vi "myRIO_BRig_RT_v0,86.vi"() -> ()   [LabVIEW 2014]
uses:
  myRIO_BRig_RT__Case_Exp_stateList.ctl
  myRIO_BRig_RT__Case_NonExp_stateList.ctl
  <vilib>/Platform/TimedLoop/XDataNode/timing_clust.ctl
  <vilib>/Platform/TimedLoop/XDataNode/nitl_modes.ctl
  <vilib>/Platform/TimedLoop/XDataNode/wakeup.ctl
  <vilib>/WebDAVClient/Advanced/SessionHandle.ctl
  <vilib>/myRIO/Common/Instrument Driver Framework/myRIO v1.0/UART/vis/myRIO v1.0 Close UART.vi
  <vilib>/FPGAPlugInAG/myRIO-1900/niLvFpga_Open_myRIO-1900.vi
  <vilib>/rvi/interface/common/dynamic/niFpgaDynamicAddResources.vi
  <vilib>/Utility/error.llb/Error Cluster From Error Code.vi
  <vilib>/rvi/errors/niLvFpgaAdjustHostInterfaceError.vi
  <vilib>/FPGAPlugInAG/Dynamic/niLvFpga_Close_Dynamic.vi
  <vilib>/myRIO/Common/Instrument Driver Framework/Utilities/vis/FPGA Ref Manager.vi
  <vilib>/myRIO/Common/Instrument Driver Framework/myRIO v1.0/myRIO v1.0 Reset FPGA.vi
  <vilib>/myRIO/Common/Instrument Driver Framework/myRIO v1.0/IRQ/vis/myRIO v1.0 IRQ Info FGV.vi
  <vilib>/myRIO/Common/Instrument Driver Framework/myRIO v1.0/IRQ/vis/myRIO v1.0 Timer IRQ Info FGV.vi
  <vilib>/myRIO/Common/Instrument Driver Framework/myRIO v1.0/IRQ/vis/myRIO v1.0 ISR Agent.vi
  <vilib>/rvi/interface/nirviOpenFPGA/nirviOpenFPGA.xnode
  myRIO_BRig_FPGA_v3,81_build.lvbitx
  myRIO_BRig_FPGA_v3,81.vi
  <vilib>/rvi/interface/nirviReadWriteControl/nirviReadWriteControl.xnode
  <vilib>/Platform/TimedLoop/XDataNode/XDataNode.xnode
  <vilib>/rvi/interface/nirviCloseFPGA/nirviCloseFPGA.xnode
  <vilib>/Platform/TimedLoop/XDataNode/XDNodeRunTimeDep.lvlib
  <vilib>/rvi/interface/Simulation/niFpgaSimulationCallBeginRW.vi
  <vilib>/myRIO/Instrument Drivers/Utilities/Utilities.lvlib
  <vilib>/WebDAVClient/NI_WebDAV.lvlib
  NiFpgaLv.dll
panel:
  in  "Laser2_baseline":bool
  in  "Laser1_baseline":bool
  in  "CueLed_baseline":bool
  out "allReward_R":bool
  out "allReward_L":bool
  in  "I_allReward":bool caption="NonSpecific Lick Direction"
  in  "Tcycle_Reward_max_R":u16=1000 caption="Max" min=5 max=5000 step=5
  in  "Tcycle_Reward_min_R":u16=1000 caption="Min" min=5 max=5000 step=5
  in  "Tcycle_Reward_step_R":u16=1000 caption="Penalty" min=1 max=10000 step=1
  in  "Tcycle_Reward_max_L":u16=1000 caption="Max" min=5 max=5000 step=5
  in  "Tcycle_Reward_min_L":u16=1000 caption="Min" min=5 max=5000 step=5
  in  "Tcycle_Reward_step_L":u16=1000 caption="Penalty" min=1 max=10000 step=1
  in  "MTrig_CueLed":bool
  out "Threshold":bool
  out "tLoop":dbl
  in  "Tcycle_Cue_LED_max":u16=1000 caption="Max" min=5 max=5000 step=5
  in  "Tcycle_Cue_LED_min":u16=1000 caption="Min" min=5 max=5000 step=5
  in  "Tcycle_CuePenalty_LED":u16=1000 caption="Penalty" min=1 max=10000 step=1
  out "power_l2":dbl
  in  "MTrig_Laser_Switch":bool
  in  "Cue1Param_AudioLed_Count_NS":u16
  in  "Cue1Param_AudioLed_Count_Switch":u16
  in  "Cue1Param_AudioLed_Probability_NS":u16
  in  "Cue1Param_CueType_NS":u16(slide) max=3 step=1 scale=0.0..3.0
  in  "Cue1Param_AudioLed_Probability_Switch":u16
  in  "Cue1Param_CueType_Switch":u16(slide) max=3 step=1 scale=0.0..3.0
  in  "CueLed_Freq":dbl=10.0
  in  "CueLed_Tpeak":dbl=2.0
  in  "Laser_power_step_l2":dbl
  in  "Laser_power_max_l2":dbl
  in  "Laser_power_min_l2":dbl
  in  "Laser_Tshutter_l2":dbl=2.0
  in  "Laser_Freq_l2":dbl=10.0
  in  "Laser_Tpeak_l2":dbl=2.0
  in  "Laser_duration_l2":u16
  in  "LC_Sel_Count_NS_l2":u16
  in  "LC_Sel_Count_Switch_l2":u16
  in  "LC_Sel_Probability_NS_l2":u16
  in  "LC_Sel_Block_NS_l2":u16(slide) max=2 step=1 scale=0.0..2.0
  in  "LC_Sel_OnOff_NS_l2":bool
  in  "LC_Sel_Probability_Switch_l2":u16
  in  "LC_Sel_Block_Switch_l2":u16(slide) max=2 step=1 scale=0.0..2.0
  in  "LC_Sel_OnOff_Switch_l2":bool
  in  "LC_Sel_Tdelay_NS_l2":u16
  in  "LC_Sel_Tdelay_Switch_l2":u16
  in  "LC_Cue1_Count_NS_l2":u16
  in  "LC_Cue1_Count_Switch_l2":u16
  in  "LC_Cue1_delayOpt_NS_l2":bool
  in  "LC_ENL1_delayOpt_NS_l2":bool
  in  "LC_ENL1_Count_NS_l2":u16
  in  "LC_ENL1_Count_Switch_l2":u16
  in  "LC_Cue1_delayOpt_Switch_l2":bool
  in  "LC_ENL1_delayOpt_Switch_l2":bool
  in  "LC_Cue1_Probability_NS_l2":u16
  in  "LC_Cue1_Block_NS_l2":u16(slide) max=2 step=1 scale=0.0..2.0
  in  "LC_Cue1_OnOff_NS_l2":bool
  in  "LC_Cue1_Probability_Switch_l2":u16
  in  "LC_Cue1_Block_Switch_l2":u16(slide) max=2 step=1 scale=0.0..2.0
  in  "LC_Cue1_OnOff_Switch_l2":bool
  in  "LC_ENL1_Probability_NS_l2":u16 max=100 step=1
  in  "LC_ENL1_Block_NS_l2":u16(slide) max=2 step=1 scale=0.0..2.0
  in  "LC_ENL1_OnOff_NS_l2":bool
  in  "LC_ENL1_Probability_Switch_l2":u16 max=100 step=1
  in  "LC_ENL1_Block_Switch_l2":u16(slide) max=2 step=1 scale=0.0..2.0
  in  "LC_Cue1_Tdelay_NS_l2":u16
  in  "LC_ENL1_Tdelay_NS_l2":u16
  in  "LC_Cue1_Tdelay_Switch_l2":u16
  in  "LC_ENL1_Tdelay_Switch_l2":u16
  in  "LC_ENL1_OnOff_Switch_l2":bool
  in  "LC_Wrong_Probability_l2":u16
  in  "LC_Wrong_Trial_l2":u16(slide) max=2 step=1 scale=0.0..2.0
  in  "LC_Wrong_Block_l2":u16(slide) max=2 step=1 scale=0.0..2.0
  in  "LC_Wrong_OnOff_l2":bool
  in  "LC_Reward_Probability_l2":u16
  in  "LC_Reward_Trial_l2":u16(slide) max=2 step=1 scale=0.0..2.0
  in  "LC_Reward_Block_l2":u16(slide) max=2 step=1 scale=0.0..2.0
  in  "LC_Reward_OnOff_l2":bool
  in  "LC_Wrong_Tdelay_l2":u16
  in  "LC_Reward_Tdelay_l2":u16
  in  "LC_Sel_Count_NS_l1":u16
  in  "LC_Sel_Count_Switch_l1":u16
  in  "LC_Sel_Probability_NS_l1":u16
  in  "LC_Sel_Block_NS_l1":u16(slide) max=2 step=1 scale=0.0..2.0
  in  "LC_Sel_OnOff_NS_l1":bool
  in  "LC_Sel_Probability_Switch_l1":u16
  in  "LC_Sel_Block_Switch_l1":u16(slide) max=2 step=1 scale=0.0..2.0
  in  "LC_Sel_OnOff_Switch_l1":bool
  in  "LC_Sel_Tdelay_NS_l1":u16
  in  "LC_Sel_Tdelay_Switch_l1":u16
  out "I_connect_TCP":bool
  in  "get_countPerMS":bool
  in  "count_warmup_R_reset":bool
  in  "count_warmup_L_reset":bool
  out "count_warmup_R":u16
  out "count_warmup_L":u16
  out "SolenoidReward":bool
  in  "SolenoidProbability_L":u16=100 caption="Reward Time [ms]" min=1 max=1000 step=1
  in  "SolenoidProbability_R":u16=100 caption="Reward Time [ms]" min=1 max=1000 step=1
  out "power_l1":dbl caption="LaserPower"
  in  "Laser_power_step_l1":dbl
  in  "Laser_power_max_l1":dbl
  in  "Recording":bool
  in  "Laser_power_min_l1":dbl
  in  "FPGA_count2ms":dbl=159.0
  in  "Laser_Tshutter_l1":dbl=2.0
  in  "Laser_Freq_l1":dbl=10.0
  in  "Laser_Tpeak_l1":dbl=2.0
  in  "Laser_duration_l1":u16
  out "error out":errorcluster
  in  "LC_Cue1_Count_NS_l1":u16
  in  "LC_Cue1_Count_Switch_l1":u16
  in  "LC_Cue1_delayOpt_NS_l1":bool
  in  "LC_ENL1_delayOpt_NS_l1":bool
  in  "LC_ENL1_Count_NS_l1":u16
  in  "LC_ENL1_Count_Switch_l1":u16
  in  "LC_Cue1_delayOpt_Switch_l1":bool
  in  "LC_ENL1_delayOpt_Switch_l1":bool
  in  "Tcycle_Cue_Audio_max":u16=1000 caption="Max" min=5 max=5000 step=5
  in  "Tcycle_Cue_Audio_min":u16=1000 caption="Min" min=5 max=5000 step=5
  in  "SendData":bool
  out "cSpout":enum16{"Left", "Right"}(ring) caption="Left or Right Spout"
  out "A4":u32 caption="LickCounter_Right"
  out "A2":u32 caption="LickCounter_Left"
  in  "LR_wrong_Event":bool
  out "SelectWrong":bool
  out "SelectReward":bool
  in  "Left(F)_or_Right(T)":bool
  in  "ignoreWrong":bool
  in  "SelectionState":bool
  in  "LR_wrong_Laser":bool
  in  "LR_reward_Laser":bool
  in  "LR_reward_Event":bool
  out "nRewards_Right":u16 caption="# Rewards Total (Right)"
  out "nRewards_Left":u16 caption="# Rewards Total (Left)"
  out "nRewards_cur":u16 caption="# Rewards in Current Block"
  out "TpB_target":u16 caption="Target Trials Per Block"
  out "cState_NonExp":T1 caption="WarmUp State"
  out "iBlock":u16 caption="Current Block"
  out "cState":T2 caption="Experimental State"
  out "iTrial":u16 caption="Current Trial"
  in  "warmupType":u8(slide) max=2 step=1 scale=0.0..2.0
  in  "TestConnection":bool
  in  "warmup":bool caption="WarmUp"
  in  "Data Set Prefix":string="Exp1_TM2"
  out "Connected To Host?":bool
  in  "Host Password":string="sabalab"
  in  "Host UserName":string="Test2"
  in  "sp_RightSpout":u16(slide)=2 max=2 step=1 scale=0.0..2.0
  in  "sp_LeftSpout":u16(slide)=2 max=2 step=1 scale=0.0..2.0
  in  "BUR_max":u16 caption="Count Reward Structure  (0 = off)"
  in  "LC_Wrong_Probability_l1":u16
  in  "LC_Wrong_Trial_l1":u16(slide) max=2 step=1 scale=0.0..2.0
  in  "LC_Wrong_Block_l1":u16(slide) max=2 step=1 scale=0.0..2.0
  in  "LC_Wrong_OnOff_l1":bool
  in  "LC_Reward_Probability_l1":u16
  in  "LC_Reward_Trial_l1":u16(slide) max=2 step=1 scale=0.0..2.0
  in  "LC_Reward_Block_l1":u16(slide) max=2 step=1 scale=0.0..2.0
  in  "LC_Reward_OnOff_l1":bool
  in  "LC_Cue1_Probability_NS_l1":u16
  in  "LC_Cue1_Block_NS_l1":u16(slide) max=2 step=1 scale=0.0..2.0
  in  "LC_Cue1_OnOff_NS_l1":bool
  in  "LC_Cue1_Probability_Switch_l1":u16
  in  "LC_Cue1_Block_Switch_l1":u16(slide) max=2 step=1 scale=0.0..2.0
  in  "LC_Cue1_OnOff_Switch_l1":bool
  in  "LC_ENL1_Probability_NS_l1":u16 max=100 step=1
  in  "LC_ENL1_Block_NS_l1":u16(slide) max=2 step=1 scale=0.0..2.0
  in  "LC_ENL1_OnOff_NS_l1":bool
  in  "LC_ENL1_Probability_Switch_l1":u16 max=100 step=1
  in  "LC_ENL1_Block_Switch_l1":u16(slide) max=2 step=1 scale=0.0..2.0
  in  "Tcycle_Timeout":u16=1000 caption="Timeout Time [ms]" min=10 max=10000 step=1
  in  "Tcycle_Wrong":u16=1000 caption="Wrong Time [ms]" min=10 max=10000 step=1
  in  "Tcycle_Selection":u16=1000 caption="Answer Time [ms]" min=1 max=10000 step=1
  in  "Tcycle_RewardPost":u16=1000 caption="Consumption Time [ms]" min=250 max=10000 step=250
  in  "TpB_Max_R":u16=4 caption="Max TrialsPerBlock" min=1 max=12 step=1
  in  "TpB_Min_R":u16=4 caption="Min TrialsPerBlock" min=1 max=12 step=1
  in  "TpB_Max_L":u16=4 caption="Max TrialsPerBlock" min=1 max=12 step=1
  in  "TpB_Min_L":u16=4 caption="Min TrialsPerBlock" min=1 max=12 step=1
  in  "BUR_min":u16 caption="Count Reward Structure\n(0 = off)"
  in  "TrialUntilReward":bool caption="Ignore Wrong Selection"
  in  "CueCycles":u16=1 caption="Cue Structure" min=1 max=1 step=1
  in  "MTrig_Laser_Tcycle":u16=10 caption="Time [ms]"
  in  "MTrig_Laser_trig":bool
  in  "MTrig_Audio_trig__R":bool caption="Trigger Audio"
  in  "MTrig_Audio_trig__L":bool caption="Trigger Audio"
  in  "RewCalib_Trig_R":bool caption="Calibrate_R"
  in  "RewCalib_Trig_L":bool caption="Calibrate_L"
  in  "MTrig_Solenoid_Tcycle__R":u16=300 caption="Time [ms]"
  in  "MTrig_Solenoid_Tcycle__L":u16=300 caption="Time [ms]"
  in  "MTrig_Solenoid_trig__R":bool caption="Solenoid"
  in  "MTrig_Solenoid_trig__L":bool caption="Solenoid"
  in  "STOP_abort":bool caption="Stop LabView\n(Stops myRio and FPGA)"
  in  "STOP_endBlock":bool caption="Stop Experiment\n@ End of Block"
  in  "STOP_endTrial":bool caption="Stop Experiment\n@ End of Trial"
  in  "START":bool caption="Start Experiment"
  in  "Tcycle_CuePenalty_Audio":u16=1000 caption="Penalty" min=1 max=10000 step=1
  in  "Audio_Amp__R":u16=100 caption="Amp"
  in  "Audio_Freq__R":u8=5 caption="Freq [kHz]" max=14 step=1
  in  "Audio_Amp__L":u16=100 caption="Amp"
  in  "Audio_Freq__L":u8=5 caption="Freq [kHz]" max=14 step=1
  in  "LC_Wrong_Tdelay_l1":u16
  in  "LC_Cue1_Tdelay_NS_l1":u16
  in  "LC_ENL1_Tdelay_NS_l1":u16
  in  "LC_Reward_Tdelay_l1":u16
  in  "LC_Cue1_Tdelay_Switch_l1":u16
  in  "LC_ENL1_Tdelay_Switch_l1":u16
  in  "LC_ENL1_OnOff_Switch_l1":bool
  in  "Tcycle_ENLPenalty":u16=100 caption="Penalty" min=10 max=10000 step=10
  in  "Tcycle_ENL_max":u16=1000 caption="Max" min=250 max=10000 step=250
  in  "Tcycle_ENL_min":u16=1000 caption="Min" min=250 max=10000 step=250
  # "Communication (Host PC)"
  # "Recording Rig"
  # "Experimental Run"
  # "Experiment Task Structure"
  # "STOP experiment at"
  # "(1) = Switching\n(2) = Two Choice"
  # "Min            Max            Penalty"
  # "Enforced\nNonLick"
  # "FPGA Count per [ms]"
  # "Cue Audio"
  # "Current State"
  # "Cue LED"
  # "Global Parameters                                                         Trial Parameters"
  # "Selection"
  # "WarmUp"
  # "Reward - Dispense Water"
  # "Left/Right        Give Reward?        Laser Power [V]"
  # "Min            Max            StepSize"
  # "Laser1      Laser2"
  # "Left"
  # "Cue then reward (no lick)\n \nLeft                    Right"
  # "Right"
  # "Min"
  # "Max"
  # "Dispense Water Probability"
  # "Block                   Trial            Target Trials       # Rewards \n                                                            Per Block             Current"
  # "%"
  # "Left"
  # "WarmUp State"
  # "Trial Per Block Structure \n               Left                        Right"
  # "Lick Counter"
  # "Right"
  # "%"
  # "Left           Right"
  # "Reward - Consumption"
  # "Manual Control"
  # "Min"
  # "# Rewards Total\n                                                                  Left                    Right"
  # "Experimental State"
  # "Penalty - Wrong Choice"
  # "Solenoid\n \nLeft              Right"
  # "Speaker\n \nLeft                    Right"
  # "Laser 1  |  Laser 2"
  # "Max"
  # "Penalty - Choice Timeout"
  # "Time\n[ms]"
  # "Time\n[ms]"
  # "Time = Cue Min"
  # "Cue LED"
  # "Power = Min"
  # "Cue1 Control\n                                  Cue Type           LED Probability [%]      Count"
  # "Laser1 Control\n                               On/Off      Block        Probability [%]   Delay [ms]                              Count"
  # "Laser2 Control\n                               On/Off      Block        Probability [%]   Delay [ms]                              Count"
  # "Audio or LED"
  # "Cue 1"
  # "Enforced\nNonLick\n      1"
  # "Enforced\nNonLick\n      1"
  # "from end"
  # "from end"
  # "Switch\nTrial"
  # "Switch\nTrial"
  # "Switch\nTrial"
  # "from start"
  # "from start"
  # "from end"
  # "from end"
  # "NonSwitch\nTrials"
  # "NonSwitch\nTrials"
  # "NonSwitch\nTrials"
  # "from start"
  # "from start"
  # "Cue 1"
  # "Cue 1"
  # "from end"
  # "from end"
  # "Switch\nTrial"
  # "Switch\nTrial"
  # "Cue Audio Parameters"
  # "Cue LED Parameters"
  # "from start"
  # "from start"
  # "Left                  Right"
  # "Frequency\n[Hz]"
  # "Frequency\n[kHz]"
  # "from end"
  # "from end"
  # "NonSwitch\nTrials"
  # "NonSwitch\nTrials"
  # "Timing [ms]\n                    Peak Width"
  # "from start"
  # "from start"
  # "Amp\n(0 - 32,000)"
  # "Selection"
  # "Selection"
  # "from start"
  # "from start"
  # "Switch\nTrial"
  # "Switch\nTrial"
  # "Speaker\nPattern\nDuring Cue"
  # "from start"
  # "from start"
  # "NonSwitch\nTrials"
  # "NonSwitch\nTrials"
  # "Laser1 Parameters"
  # "Laser2 Parameters"
  # "Laser1 Response\n                               On/Off      Block       Trial       Probability [%]   Delay [ms]"
  # "Laser2 Response\n                               On/Off      Block       Trial       Probability [%]   Delay [ms]"
  # "Frequency\n[Hz]"
  # "Frequency\n[Hz]"
  # "Timing [ms]\n Duration     Peak Width   Shutter"
  # "Timing [ms]\n Duration     Peak Width   Shutter"
  # "Selection Reward"
  # "Selection Reward"
  # "Laser Power [V]\nMin          Max              Step"
  # "Laser Power [V]\nMin          Max              Step"
  # "Selection Wrong"
  # "Selection Wrong"
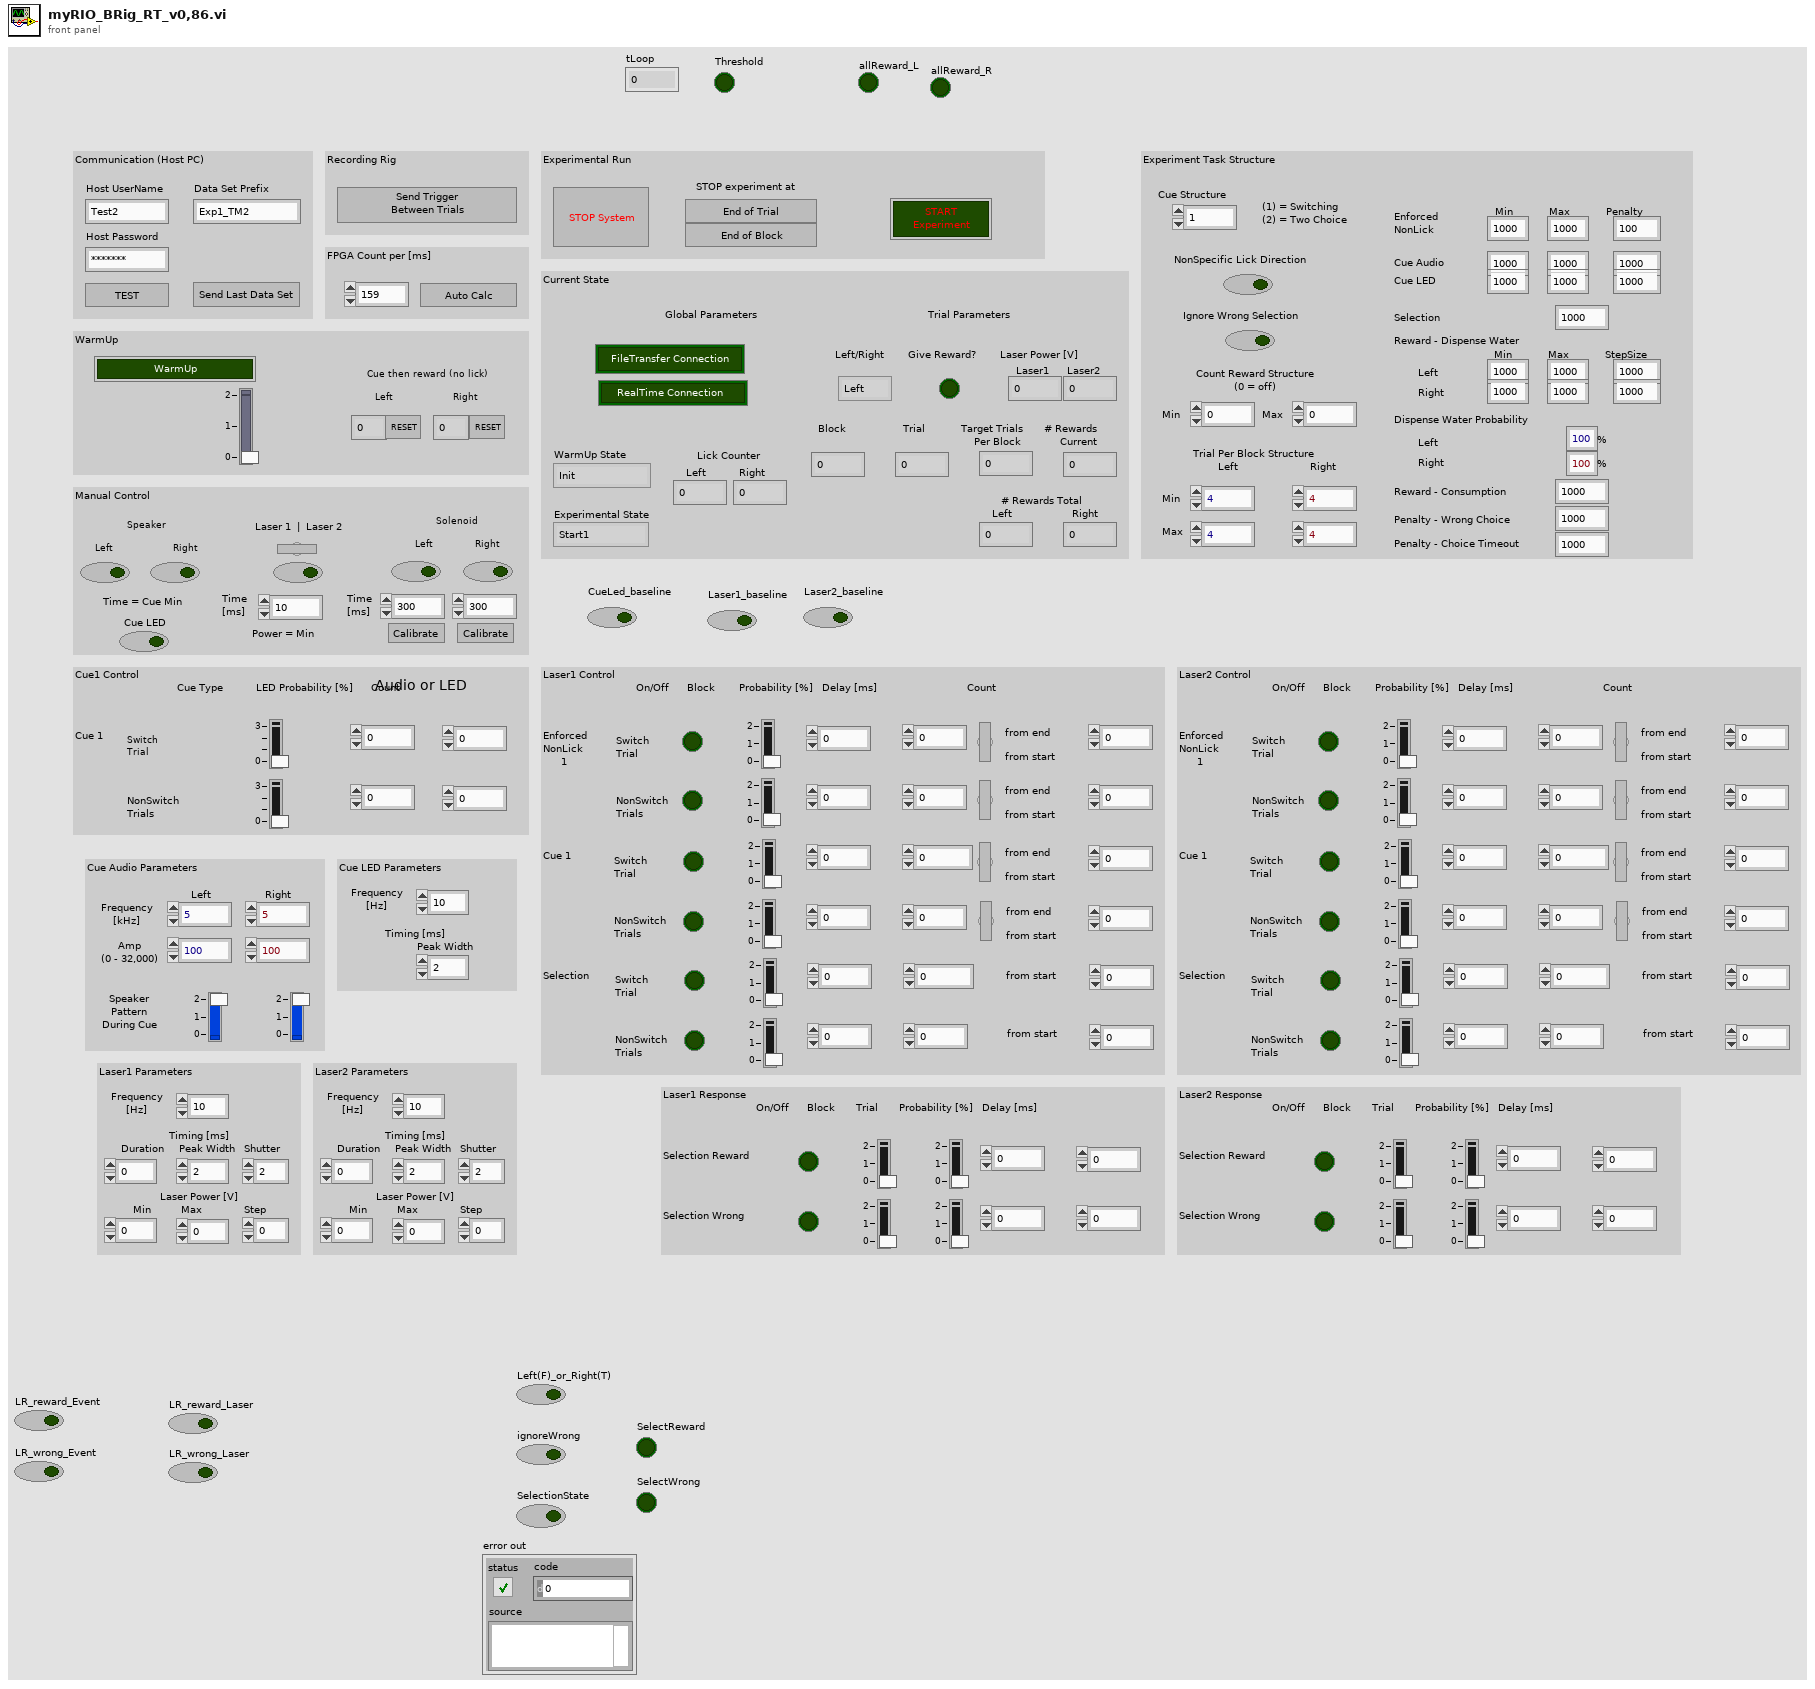
[diagram p1: front panel]
types:
  T1 = typedef "myRIO_BRig_RT__Case_NonExp_stateList.ctl" = enum16{"Init", "UploadSettings_pre", "UploadSettings_Read_dataExp", "UploadSettings_dataExp_1", "UploadSettings_dataExp_2", "UploadSettings_Read_dataLC", "UploadSettings_dataLC_1", "UploadSettings_dataLC_2", "UploadSettings_dataLC_3", "UploadSettings_dataLC_4", "UploadSettings_Read_dataMTrig", "UploadSettings_dataMTrig_1", "UploadSettings_post", "Idle_pre", "IdleEmpty", "IdleEmpty2", "IdleEmpty3", "IdleEmpty4", "Idle", "Idle_2", "Idle_3", "Idle_4", "Idle_5", "Idle_6", "Idle_post", "Cue_pre__pre", "Cue_pre", "Cue", "Cue_LED", "Cue_post", "RewardCalibration_pre", "DispenseWater_pre__pre", "DispenseWater_pre", "DispenseWater", "DispenseWater_post", "TestConnection", "SendData", "Get_FPGA_count_per_ms", "End"}
  T2 = typedef "myRIO_BRig_RT__Case_Exp_stateList.ctl" = enum16{"Start1", "Start2", "Start3", "saveSettings1", "saveSettings2", "saveSettings3", "saveSettings4", "saveSettings_LC_ENL_l1", "saveSettings_LC_ENL_l2", "saveSettings_LC_Cue_l1", "saveSettings_LC_Cue_l2", "saveSettings6_LC_l1_Other", "SaveSettings6_LC_l2_Other", "setSettings_Audio", "setSettings_Laser", "initBlock_pre", "initBlock", "initBlock2", "initBlock_post", "initTrial_pre", "initTrial", "initTrial2", "initTrial3", "initTrial4", "initTrial_LC_ENL1", "initTrial_LC_Cue1", "initTrial_LC_Cue1_2", "initTrial_LC_Sel", "initTrial_post", "ENL1_pre", "ENL1", "ENL1_post", "ENL1Penalty_pre", "ENL1Penalty", "ENL2_pre", "ENL2", "ENL2Penalty_pre", "ENL2Penalty", "Cue1_pre", "Cue1", "Cue1_post", "Cue1Penalty_pre", "Cue1Penalty", "Cue2_pre", "Cue2", "Cue2Penalty_pre", "Cue2Penalty", "Selection_pre", "Selection", "Select_post", "SelectReward_pre", "SelectReward", "SelectRewardPost_pre", "SelectRewardPost", "SelectWrong_pre", "SelectWrong", "SelectWrong_post", "SelectTimeout_pre", "SelectTimeout", "SelectTimeout_post", "endTrial_pre", "endTrial1", "endTrial2", "endTrial3", "endTrial_post", "endBlock_pre", "endBlock", "endBlock_post", "endExp", "commConnect", "commUpload_pre", "commUpload_dataBlock", "commUpload_dataCurrent", "commUpload_dataExp", "commUpload_dataLC", "commUpload_dataTrial", "commUpload_post", "saveData_pre", "saveData_dataBlock", "saveData_dataCurrent", "saveData_dataExp", "saveData_dataLC", "saveData_dataTrial", "saveData_post", "empty_endBlock1", "empty_endBlock2", "empty_endTrial1", "empty_endTrial2", "empty_endTrial3", "empty_endTrial4", "empty_endTrial5", "dummyState", "dummyState_endBlock"}
  T3 = typedef "XDNodeRunTimeDep.lvlib/timing_clust.ctl" = cluster{"Expected End [f-1]":u64, "Actual End [f-1]":u64, "Finished Late? [f-1]":bool, "Expected End [i-1]":u64, "Actual End [i-1]":u64, "Finished Late? [i-1]":bool, "Expected Start [i]":u64, "Actual Start [i]":u64, "Expected Start [f]":u64, "Actual Start [f]":u64, "Source Name":string, "Structure Name":string, "Period":i64, "Deadline":i64, "Offset":i64, "Start":i64, "Priority":i32, "Timeout":i32, "Mode":T4, "Wakeup Reason":T5, "Error":errorcluster, "Source Type":string, "Secondary Source Type":string, "Global End Time":u64, "Global Start Time":u64, "Frame Duration":u64, "Iteration Duration":u64, "Assigned CPU":i32, "I/O Scan Engine Mode":u32}
  T4 = typedef "XDNodeRunTimeDep.lvlib/nitl_modes.ctl" = enum32{"No Change", "Process missed periods, maintain original phase", "Discard missed periods, maintain original phase", "Process missed periods, ignore original phase", "Discard missed periods, ignore original phase"}
  T5 = typedef "XDNodeRunTimeDep.lvlib/wakeup.ctl" = enum32{"Normal", "Aborted", "Asynchronous wakeup", "Timing source error", "Timed loop error", "Timeout"}
  T6 = typedef "NI_WebDAV.lvlib/SessionHandle.ctl" = refnum<k1>
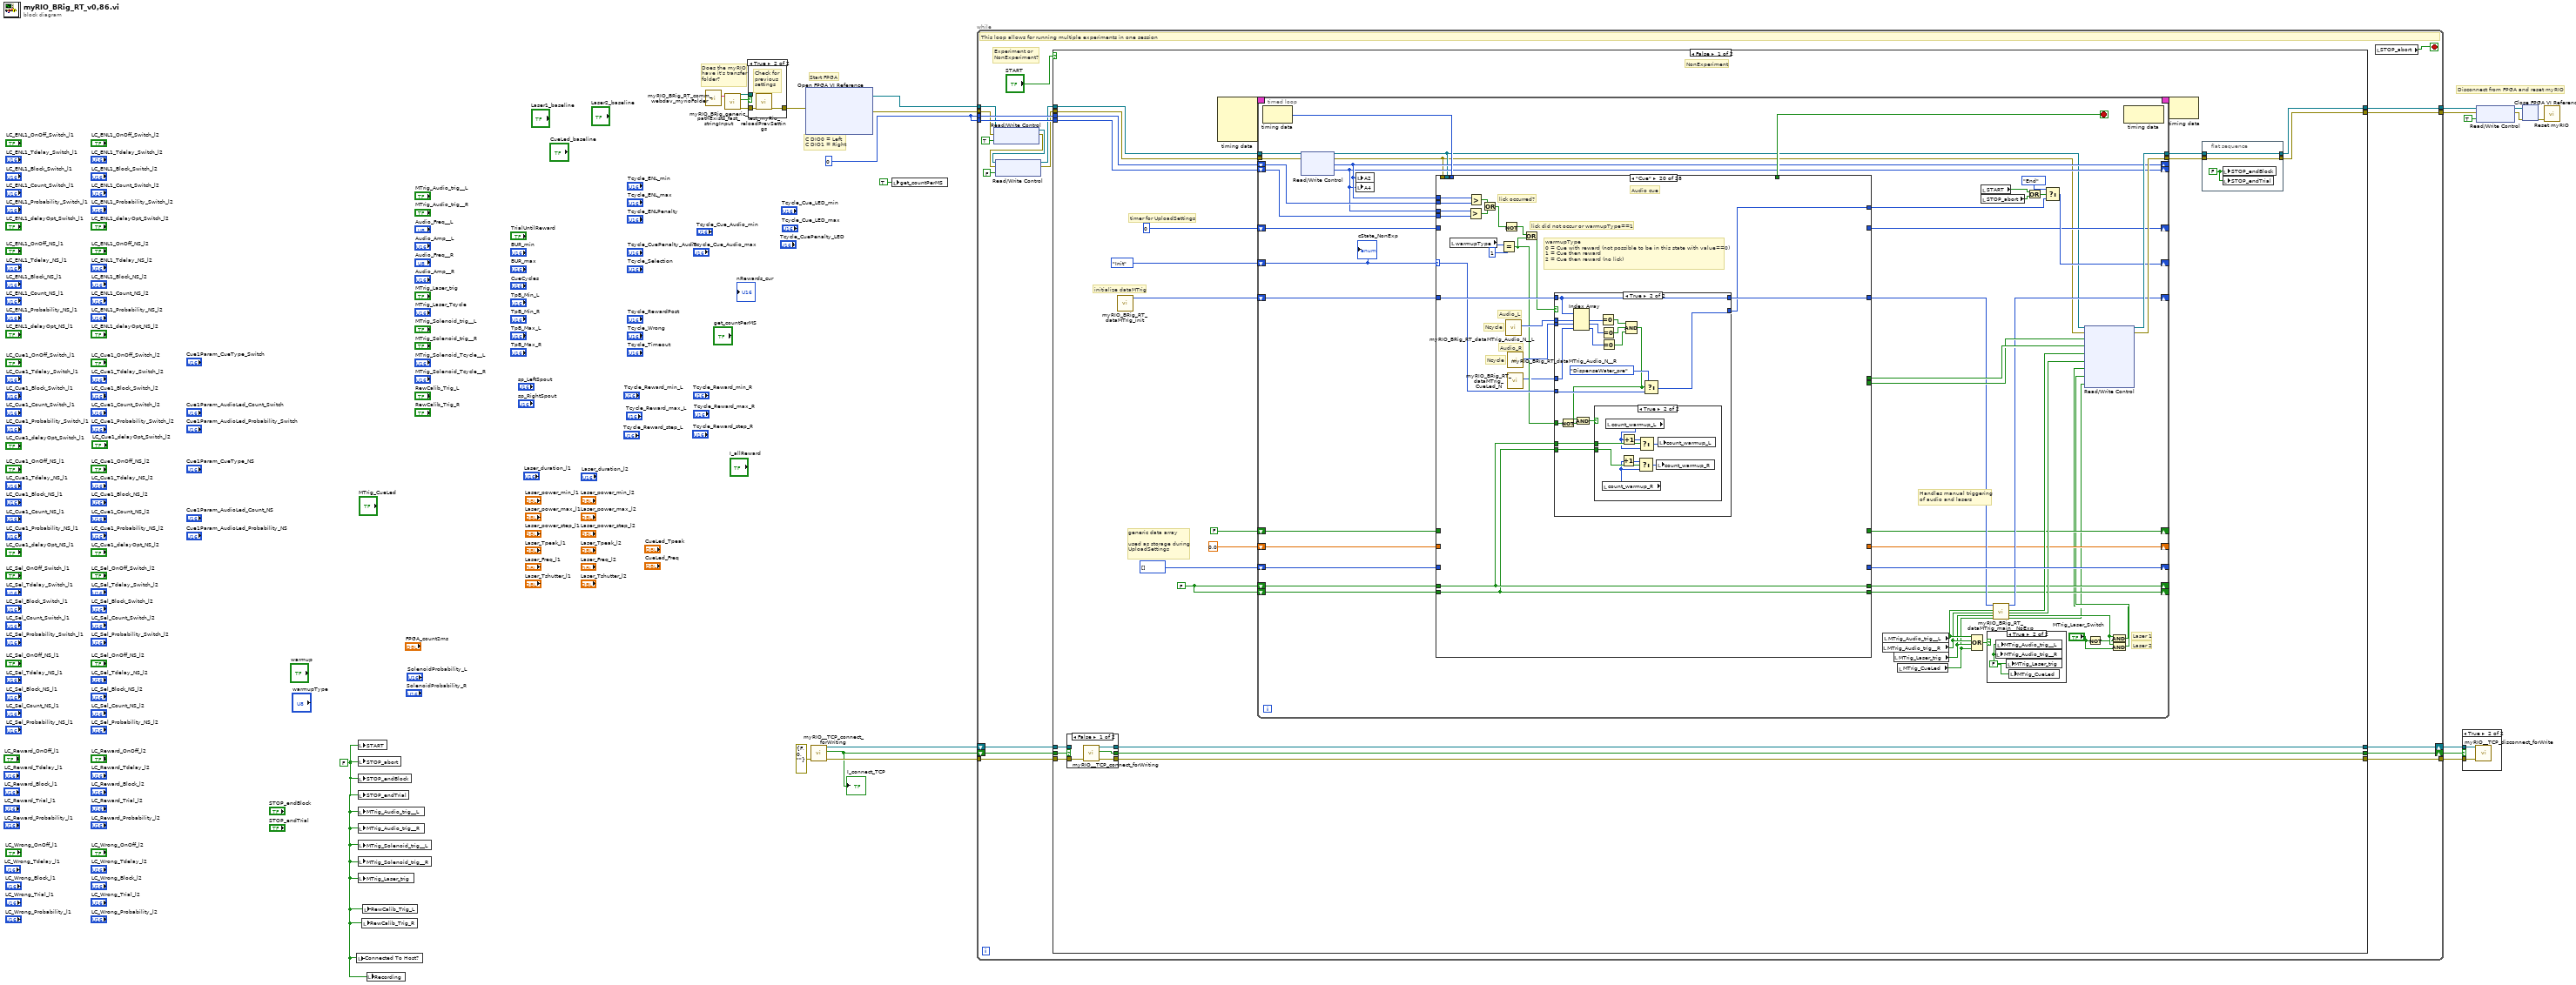
[diagram p0: block diagram]
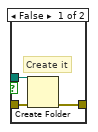
[diagram p3: hidden frame]
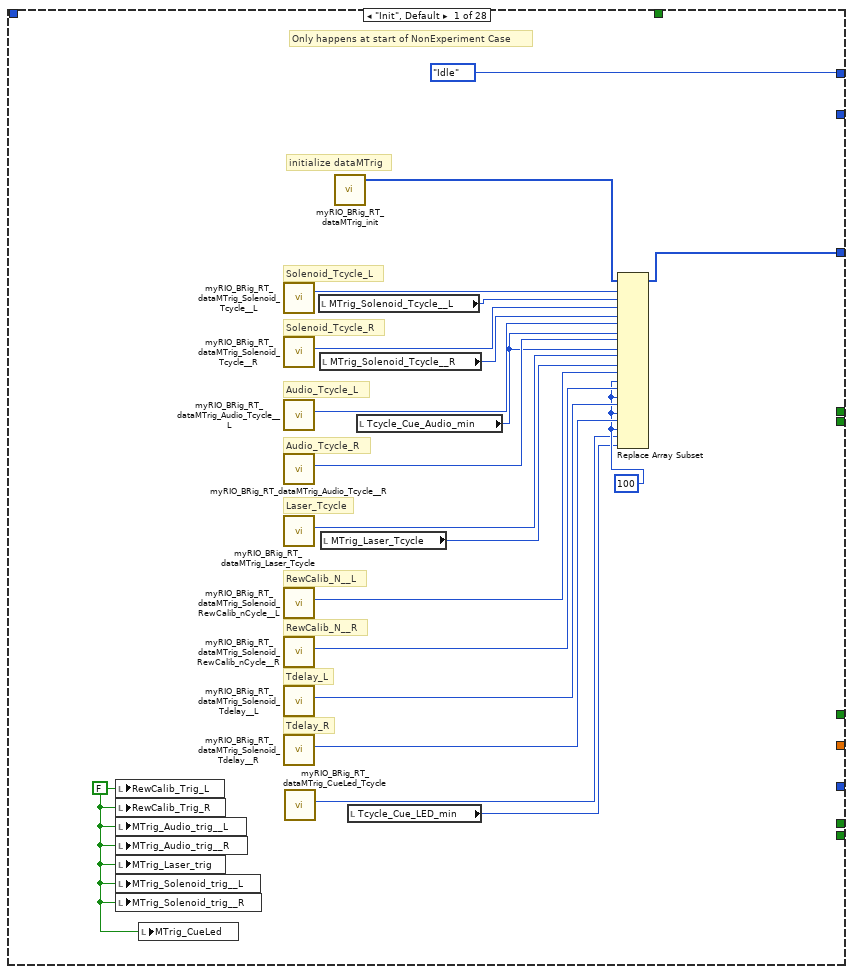
[diagram p6: hidden frame]
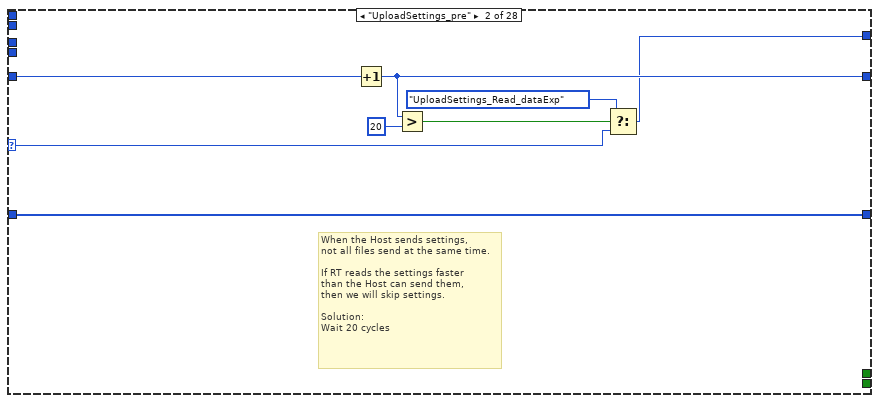
[diagram p7: hidden frame]
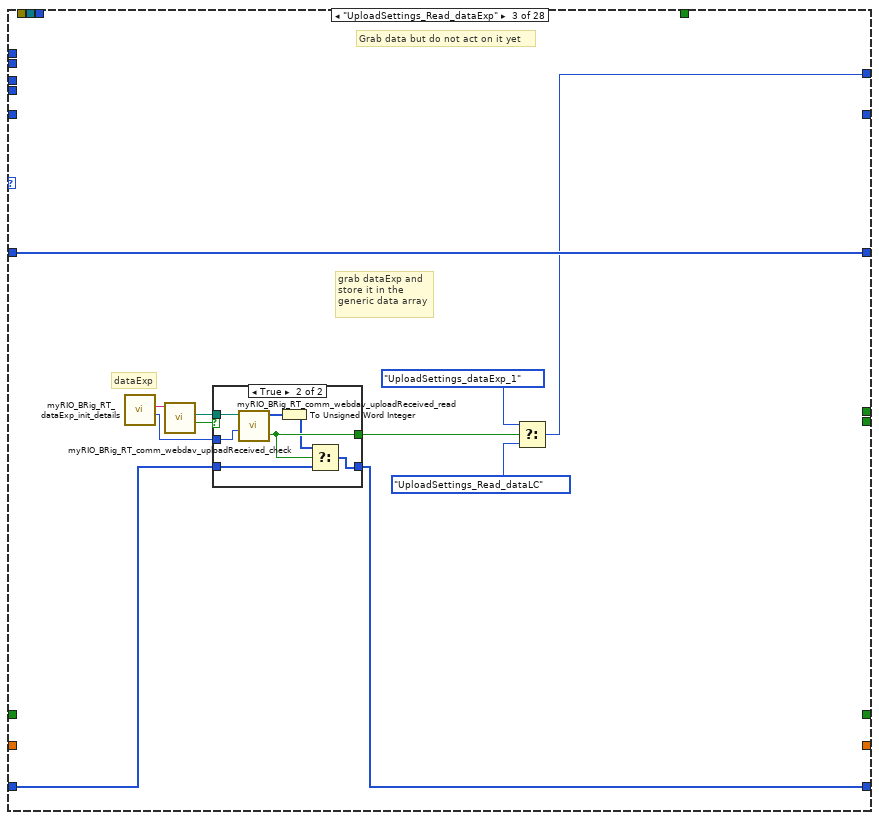
[diagram p8: hidden frame]
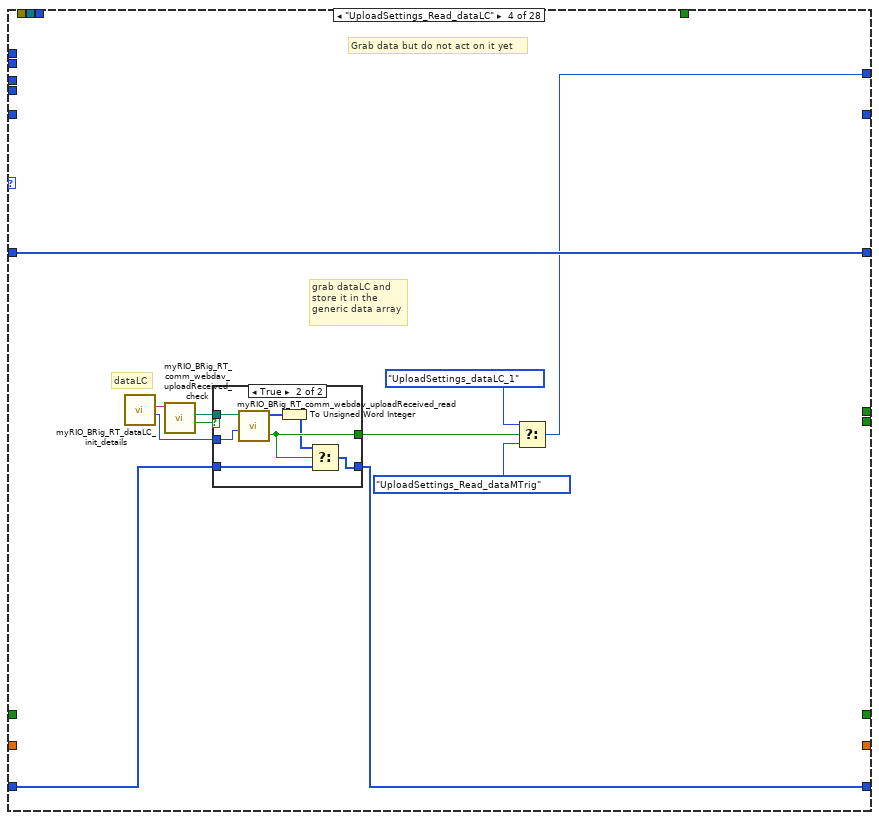
[diagram p10: hidden frame]
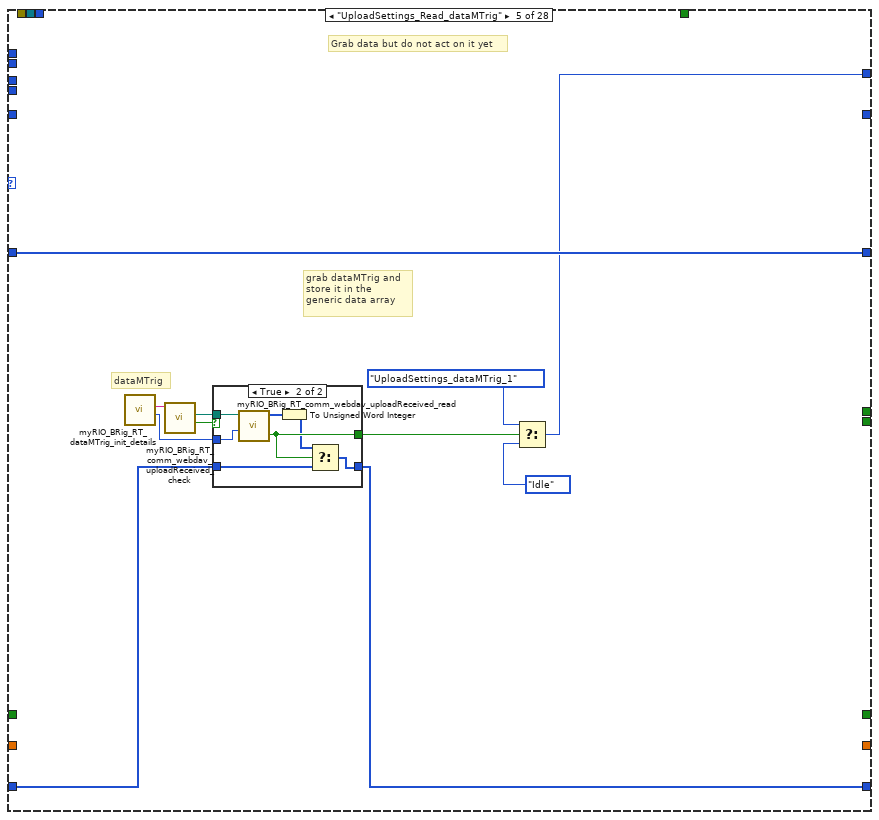
[diagram p12: hidden frame]
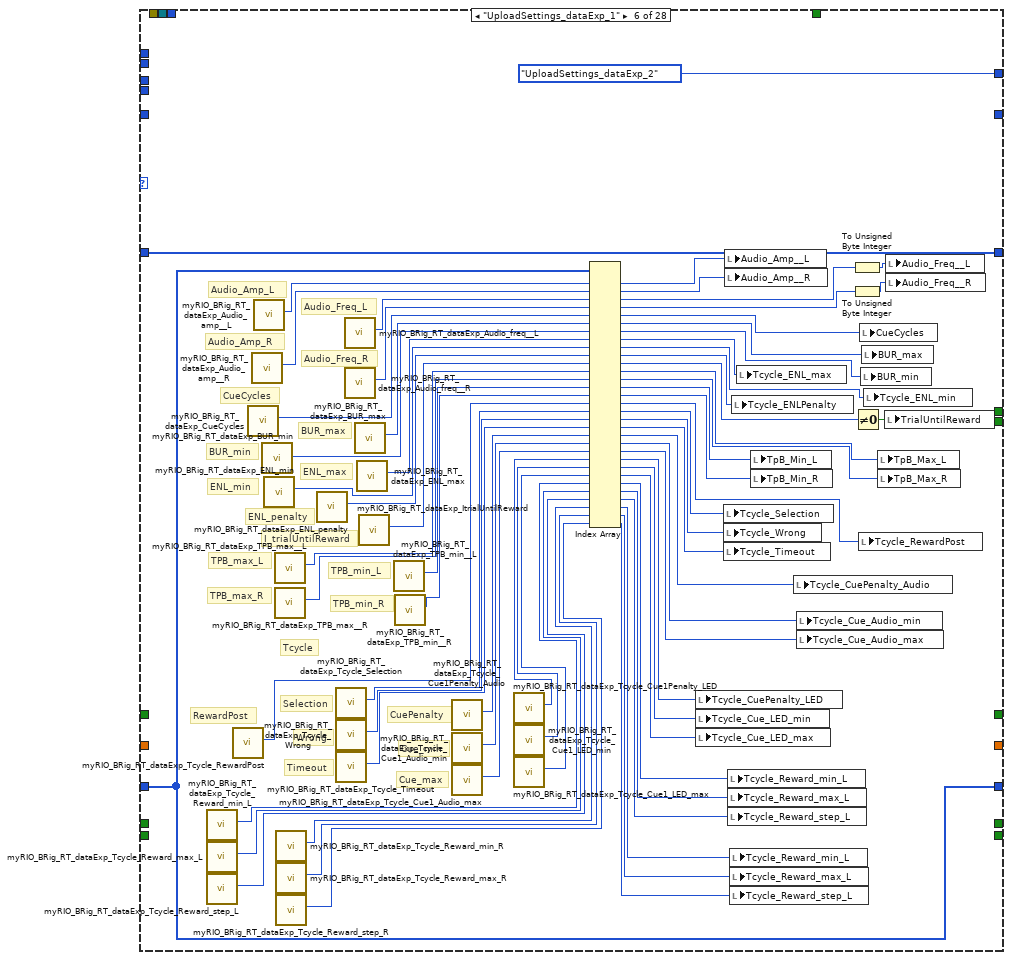
[diagram p14: hidden frame]
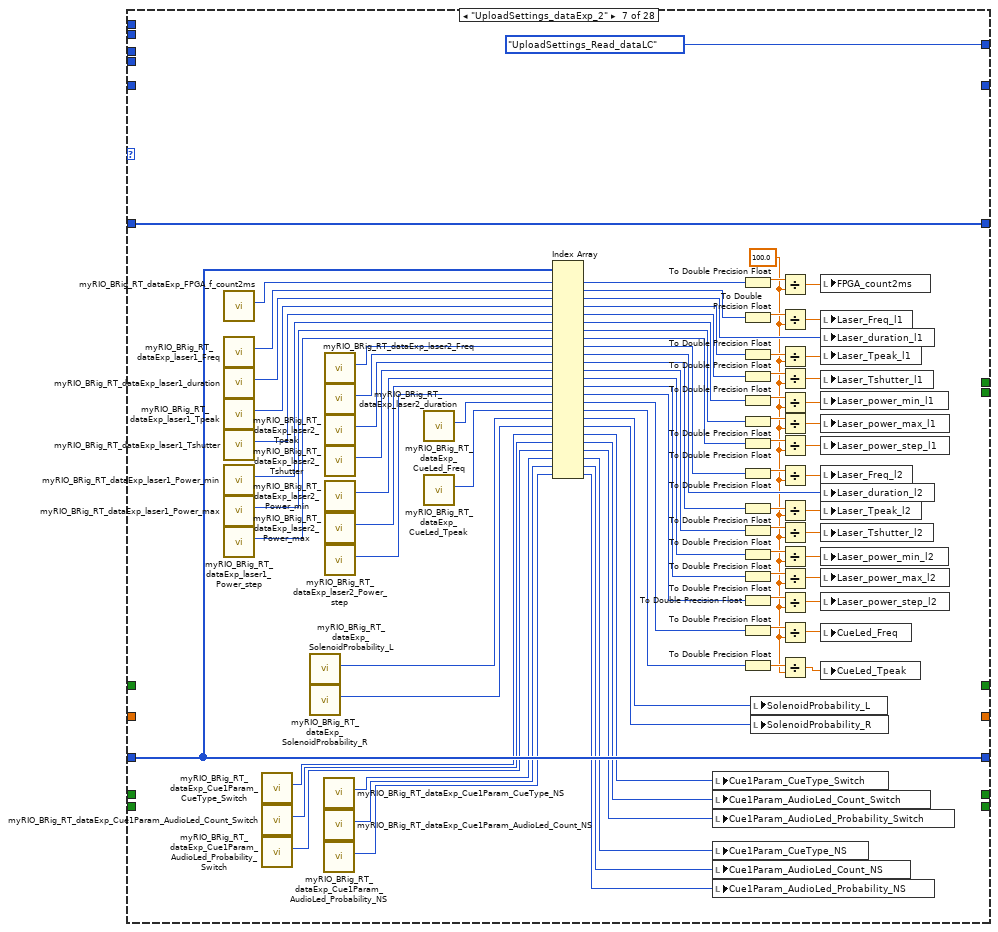
[diagram p15: hidden frame]
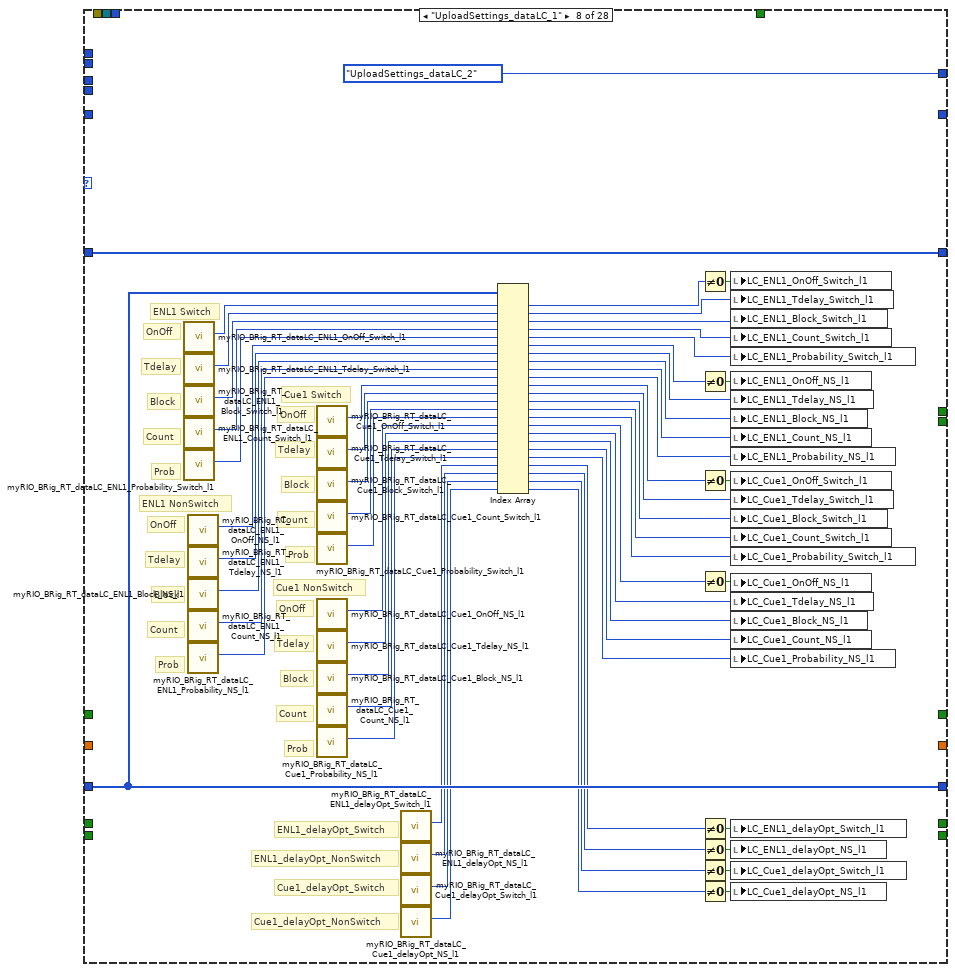
[diagram p16: hidden frame]
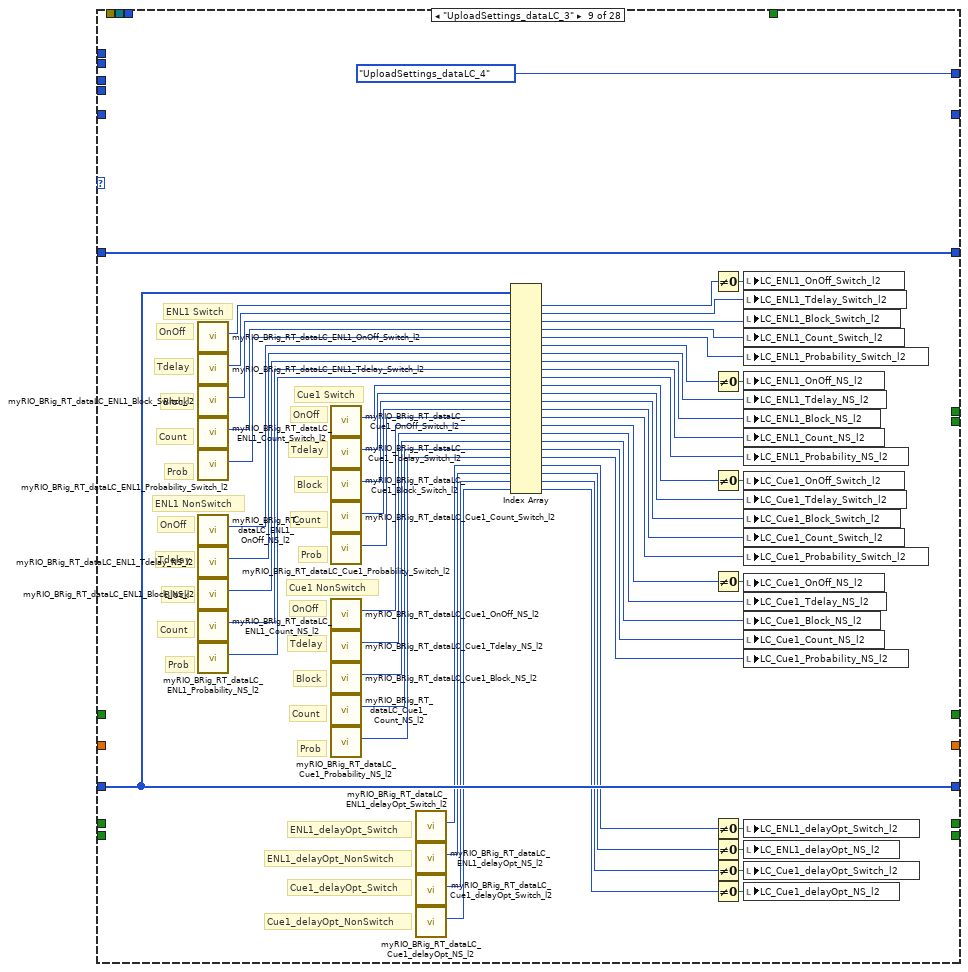
[diagram p17: hidden frame]
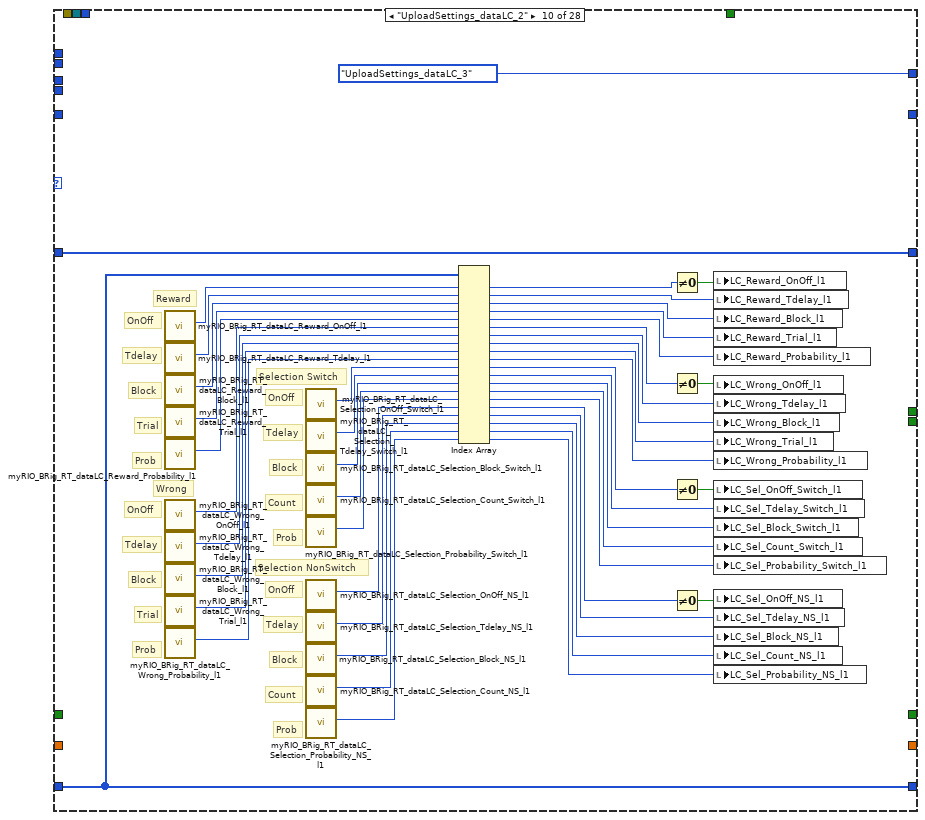
[diagram p18: hidden frame]
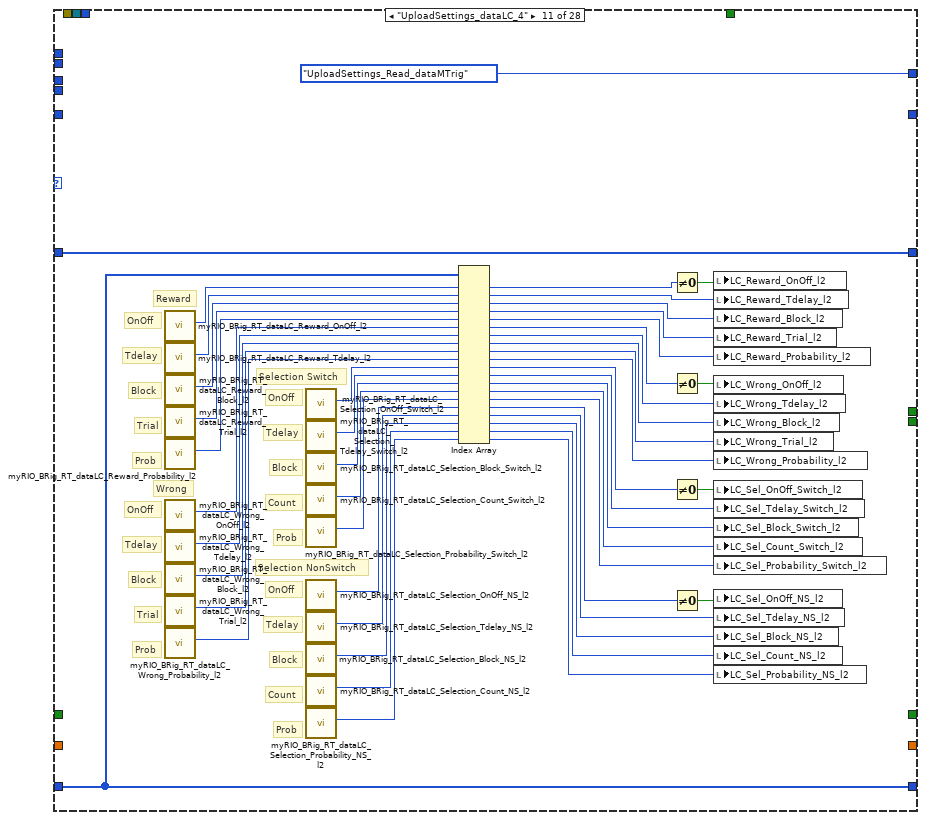
[diagram p19: hidden frame]
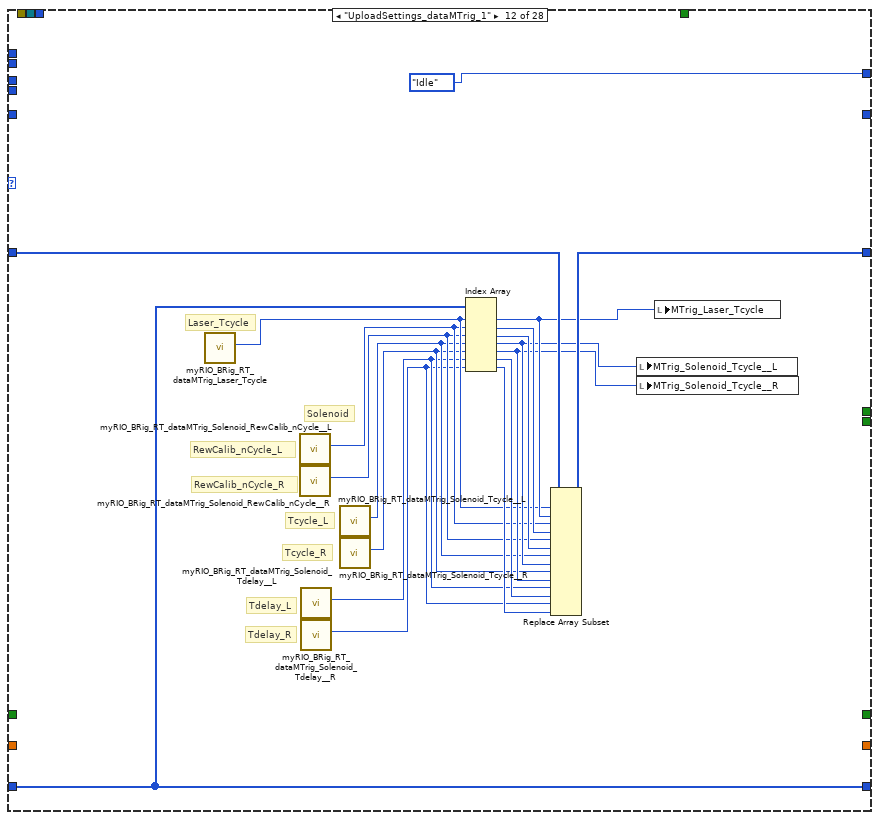
[diagram p20: hidden frame]
diagram:
  w17 = u32 0
  w1 = FALSE
  # "Does the myRIO\nhave it's transfer\nfolder?"
  # "C DIO0 = Left\nC DIO1 = Right"
  # "Start FPGA"
  # "Disconnect from FPGA and reset myRIO"
  n1 = local write "Connected To Host?"(w1) -> ()
  n2 = local write "START"(w1) -> ()
  n3 = local write "STOP_abort"(w1) -> ()
  n4 = local write "STOP_endBlock"(w1) -> ()
  n5 = local write "STOP_endTrial"(w1) -> ()
  n6 = local write "MTrig_Audio_trig__L"(w1) -> ()
  n7 = local write "MTrig_Audio_trig__R"(w1) -> ()
  n8 = local write "MTrig_Solenoid_trig__L"(w1) -> ()
  n9 = local write "MTrig_Solenoid_trig__R"(w1) -> ()
  n10 = local write "MTrig_Laser_trig"(w1) -> ()
  n11 = local write "RewCalib_Trig_R"(w1) -> ()
  n12 = local write "RewCalib_Trig_L"(w1) -> ()
  n13 = local write "Recording"(w1) -> ()
  n14 = call "myRIO_BRig_RT_comm_webdav_myrioFolder.vi"() -> ("output_myrioFolder"=w14:string)  [unwired: 11 in]
  n15 = call "myRIO_BRig_generic_pathExists_fast_stringInput.vi"("input_filePath"=w14) -> ("output_error"=w13:errorcluster, "output_Iexist"=w12:bool, "output_filePath"=w11:path)  [unwired: 8 in]
  n16 = case shown="True" w12 {
    tunnel: w11 -> [w26 _]
    tunnel: w13 -> [w25 w28]
    tunnel: [w24 w27] -> w9
    frame False {
      # "Create it"
      n17 = Create Folder(path (use dialog)=w26, error in=w25) -> (error out=w24:errorcluster)  [unwired: 1 in, 2 out]
    }
    frame True {
      # "Check for\nprevious\nsettings"
      n18 = call "test_myRio_reloadPrevSettings.vi"("input_error"=w28) -> ("output_error"=w27:errorcluster)  [unwired: 10 in]
    }
  }
  n19 = xnode "Open FPGA VI Reference"("error in"=w9) -> ("FPGA VI Reference Out"=w19:refnum<k20>, "error out"=w18:errorcluster)  [unwired: 1 in]
  n20 = call "myRIO__TCP_connect_forWriting.vi"("input_error"=errorcluster {"status"=FALSE, "code"=0, "source"=""}) -> ("output_error"=w7:errorcluster, "output_connected"=w6:bool, "output_hTCP"=w10:refnum<k5>)  [unwired: 8 in]
  "I_connect_TCP" <- w6
  n21 = local write "get_countPerMS"(TRUE ("get_countPerMS")) -> ()
  n22 = while {
    tunnel: w19 -> [w38]
    tunnel: w18 -> [w43]
    tunnel: w17 -> [w46]
    tunnel: w17 -> [w45]
    tunnel: [w36] -> w16
    tunnel: [w35] -> w15
    shift-right: [w32] -> w5
    shift-left: w6 -> [w33]
    tunnel: w7 -> [w31]
    shift-right: [w30] -> w4
    shift-left: w10 -> [w34]
    tunnel: [w29] -> w3
    stop <- w44 stop-if-true
    # "Experiment or\nNonExperiment?"
    # "This loop allows for running multiple experiments in one session"
    n23 = xnode "Read/Write Control"("FPGA VI Reference In"=w38, "error in"=w43, "Counts_Reset"=TRUE) -> ("FPGA VI Reference Out"=w40:refnum<k20>, "error out"=w41:errorcluster)
    n24 = xnode "Read/Write Control"("FPGA VI Reference In"=w40, "error in"=w41, "Counts_Reset"=FALSE) -> ("FPGA VI Reference Out"=w37:refnum<k20>, "error out"=w39:errorcluster)
    n25 = case shown="False" "START" {
      tunnel: w46 -> [w67 w1436]
      tunnel: w45 -> [w66 w1435]
      tunnel: w39 -> [w64 w1370]
      tunnel: w37 -> [w65 w1371]
      tunnel: [w62 w1432] -> w36
      tunnel: [w60 w1427] -> w35
      tunnel: w34 -> [w53 w1381]
      tunnel: [w51 w1385] -> w30
      tunnel: w33 -> [w52 w1383]
      tunnel: [w50 w1384] -> w32
      tunnel: w31 -> [w54 w1382]
      tunnel: [w49 w1380] -> w29
      frame False {
        w57 = FALSE
        # "generic data array\n\nused as storage during\nUploadSettings"
        # "timer for UploadSettings"
        # "initialize dataMTrig"
        # "NonExperiment"
        n26 = case shown="False" w52 {
          selector: w52 -> [_ w76]
          tunnel: w54 -> [w73 w78]
          tunnel: [w74 w78] -> w49
          tunnel: w53 -> [_ w77]
          tunnel: [w75 w77] -> w51
          tunnel: [w72 w76] -> w50
          frame False {
            n27 = call "myRIO__TCP_connect_forWriting.vi"("input_error"=w73) -> ("output_error"=w74:errorcluster, "output_connected"=w72:bool, "output_hTCP"=w75:refnum<k5>)  [unwired: 8 in]
          }
          frame True {
          }
        }
        n28 = call "myRIO_BRig_RT_dataMTrig_init.vi"() -> ("output_dataMTrig"=w68:u16[])  [unwired: 5 in]
        n29 = node-c288() -> (w71:T3)  [unwired: 4 in]
        n30 = timed-loop {
          timing: w71 -> [_]
          timing-out: [_] -> w70
          shift-right: [w117] -> _
          shift-left: w68 -> [w129]
          shift-right: [w111] -> _
          shift-left: myRIO_BRig_RT__Case_NonExp_stateList."Init" ("Enum") -> [w123]
          shift-right: [w105] -> _
          shift-left: w67 -> [w106]
          shift-right: [w103] -> _
          shift-left: w66 -> [w104]
          tunnel: [w125] -> w63
          tunnel: [w124] -> w61
          tunnel: w64 -> [w127]
          tunnel: w65 -> [w126]
          shift-right: [w122] -> _
          shift-left: u16[] [] ("output_data") -> [w121]
          shift-right: [w107] -> _
          shift-left: u16 0 ("Audio_Amp__L") -> [w108]
          shift-right: [w100] -> _
          shift-left: w57 -> [w102]
          shift-right: [w99] -> _
          shift-left: w57 -> [w101]
          shift-right: [w95] -> _
          shift-left: FALSE -> [w96]
          shift-right: [w93] -> _
          shift-left: 0.0 -> [w94]
          stop <- w130 stop-if-true
          # "Laser 2"
          # "Laser 1"
          # "Handles manual triggering\nof audio and lasers"
          n31 = node-c288() -> (w128:i64)  [unwired: 1 in]
          n32 = xnode "Read/Write Control"("FPGA VI Reference In"=w126, "error in"=w127) -> ("FPGA VI Reference Out"=w98:refnum<k20>, "error out"=w97:errorcluster, "A2_LickL"=w105:u32, "A4_LickR"=w103:u32)
          n33 = local write "A2"(w105) -> ()
          n34 = local write "A4"(w103) -> ()
          n35 = case shown="\"Cue\"" w123 {
            selector: w123 -> [_ w155 _ _ _ _ _ _ _ _ _ _ _ _ _ _ _ _ _ w1042 _ _ w1249 _ _ _ w1322 w1363]
            tunnel: [myRIO_BRig_RT__Case_NonExp_stateList."Idle" ("Enum") w153 w160 w179 w198 myRIO_BRig_RT__Case_NonExp_stateList."UploadSettings_dataExp_2" ("Enum") myRIO_BRig_RT__Case_NonExp_stateList."UploadSettings_Read_dataLC" ("Enum") myRIO_BRig_RT__Case_NonExp_stateList."UploadSettings_dataLC_2" ("Enum") myRIO_BRig_RT__Case_NonExp_stateList."UploadSettings_dataLC_4" ("Enum") myRIO_BRig_RT__Case_NonExp_stateList."UploadSettings_dataLC_3" ("f") myRIO_BRig_RT__Case_NonExp_stateList."UploadSettings_Read_dataMTrig" ("f") myRIO_BRig_RT__Case_NonExp_stateList."Idle" ("Enum") w621 w657 myRIO_BRig_RT__Case_NonExp_stateList."Idle_5" ("Enum") w730 w849 w978 myRIO_BRig_RT__Case_NonExp_stateList."Cue" ("t") w1037 myRIO_BRig_RT__Case_NonExp_stateList."DispenseWater_pre" ("Enum") w1195 w1247 w1269 myRIO_BRig_RT__Case_NonExp_stateList."Idle" ("Enum") myRIO_BRig_RT__Case_NonExp_stateList."Idle" ("Enum") w1321 w1363] -> w112
            tunnel: [w143 w152 w170 w189 w208 w284 w368 w421 w480 w533 w580 w596 w625 w672 w716 w735 w853 w976 w1014 w1043 w1106 w1232 w1254 w1280 w1314 w1319 w1331 w1361] -> w118
            tunnel: [_ _ _ _ _ _ _ _ _ _ _ _ _ _ _ _ _ _ _ _ _ _ _ _ _ _ _ TRUE] -> w130
            tunnel: w129 -> [_ w152 w170 w189 w208 w284 w368 w421 w480 w533 w580 w597 w624 w672 w716 w736 w854 w976 w1015 w1044 w1092 w1228 w1255 w1281 w1314 w1319 w1331 w1361]
            tunnel: w128 -> [_ _ _ _ _ _ _ _ _ _ _ _ _ _ _ _ _ _ _ _ _ _ w1259 _ _ _ _ _]
            tunnel: [_ _ w161 w180 w199 w249 w366 w422 w481 w529 w576 w581 _ _ _ _ _ _ w1006 _ _ _ _ _ _ _ _ _] -> w122
            tunnel: w121 -> [_ _ w162 w181 w200 w249 w366 w422 w481 w529 w576 w581 _ _ _ _ _ _ _ _ _ _ _ _ _ _ _ _]
            tunnel: [_ _ _ _ _ _ _ _ _ _ _ _ _ _ _ _ _ _ _ _ _ _ w1256 _ _ _ _ _] -> w120
            tunnel: [_ _ _ _ _ _ _ _ _ _ _ _ _ _ _ _ _ _ _ _ _ _ w1238 _ _ _ _ _] -> w119
            tunnel: w108 -> [_ w159 _ _ _ _ _ _ _ _ _ _ _ _ _ _ _ _ _ _ _ _ _ _ _ _ _ _]
            tunnel: [_ w158 _ _ _ _ _ _ _ _ _ _ _ _ _ _ _ _ _ _ _ _ _ _ _ _ _ _] -> w107
            tunnel: w106 -> [_ _ _ _ _ _ _ _ _ _ _ _ _ _ _ _ _ _ _ w1048 _ _ _ _ _ _ _ _]
            tunnel: w105 -> [_ _ _ _ _ _ _ _ _ _ _ _ _ _ _ _ _ _ _ w1049 _ _ _ _ _ _ _ _]
            tunnel: w104 -> [_ _ _ _ _ _ _ _ _ _ _ _ _ _ _ _ _ _ _ w1046 _ _ _ _ _ _ _ _]
            tunnel: w103 -> [_ _ _ _ _ _ _ _ _ _ _ _ _ _ _ _ _ _ _ w1047 _ _ _ _ _ _ _ _]
            tunnel: w102 -> [_ _ _ _ _ _ _ _ _ _ _ _ _ _ _ _ _ _ _ w1034 _ _ _ _ _ _ _ _]
            tunnel: w101 -> [_ _ _ _ _ _ _ _ _ _ _ _ _ _ _ _ _ _ _ w1033 _ _ _ _ _ _ _ _]
            tunnel: [_ _ _ _ _ _ _ _ _ _ _ _ _ _ _ _ _ _ w1008 w1034 _ _ _ _ _ _ _ _] -> w100
            tunnel: [_ _ _ _ _ _ _ _ _ _ _ _ _ _ _ _ _ _ w1007 w1033 _ _ _ _ _ _ _ _] -> w99
            tunnel: w98 -> [_ _ _ _ _ _ _ _ _ _ _ _ w614 w630 w718 _ _ _ _ _ _ _ _ _ _ _ w1326 _]
            tunnel: w97 -> [_ _ _ _ _ _ _ _ _ _ _ _ w613 w631 w717 _ _ _ _ _ _ _ _ _ _ _ w1325 _]
            tunnel: w96 -> [_ _ _ _ _ _ _ _ _ _ _ _ _ _ _ _ _ _ _ _ _ _ _ _ _ _ w1330 _]
            tunnel: [_ _ _ _ _ _ _ _ _ _ _ _ _ _ _ _ _ _ _ _ _ _ _ _ _ _ TRUE _] -> w95
            tunnel: w94 -> [_ _ _ _ _ _ _ _ _ _ _ _ _ _ _ _ _ _ _ _ _ _ _ _ _ _ w1328 _]
            tunnel: [_ _ _ _ _ _ _ _ _ _ _ _ _ _ _ _ _ _ _ _ _ _ _ _ _ _ w1327 _] -> w93
            frame "Init", Default {
              w134 = FALSE ("RewCalib_Trig_L")
              w135 = u16 100 ("new element/subarray")
              # "Only happens at start of NonExperiment Case"
              # "Tdelay_R"
              # "Tdelay_L"
              # "RewCalib_N__R"
              # "RewCalib_N__L"
              # "Solenoid_Tcycle_R"
              # "Solenoid_Tcycle_L"
              # "Laser_Tcycle"
              # "Audio_Tcycle_R"
              # "Audio_Tcycle_L"
              # "initialize dataMTrig"
              n36 = local write "RewCalib_Trig_L"(w134) -> ()
              n37 = local write "RewCalib_Trig_R"(w134) -> ()
              n38 = local write "MTrig_Audio_trig__L"(w134) -> ()
              n39 = local write "MTrig_Audio_trig__R"(w134) -> ()
              n40 = local write "MTrig_Laser_trig"(w134) -> ()
              n41 = local write "MTrig_Solenoid_trig__L"(w134) -> ()
              n42 = local write "MTrig_Solenoid_trig__R"(w134) -> ()
              n43 = local write "MTrig_CueLed"(w134) -> ()
              n44 = call "myRIO_BRig_RT_dataMTrig_Solenoid_Tcycle__L.vi"() -> ("output_Solenoid_Tcycle__L"=w145:i32)  [unwired: 11 in]
              n45 = call "myRIO_BRig_RT_dataMTrig_Solenoid_Tcycle__R.vi"() -> ("output_Solenoid_Tcycle__R"=w146:i32)  [unwired: 11 in]
              n46 = call "myRIO_BRig_RT_dataMTrig_Audio_Tcycle__L.vi"() -> ("output_Audio_Tcycle__L"=w147:i32)  [unwired: 11 in]
              n47 = call "myRIO_BRig_RT_dataMTrig_Audio_Tcycle__R.vi"() -> ("output_Audio_Tcycle__R"=w148:i32)  [unwired: 11 in]
              n48 = call "myRIO_BRig_RT_dataMTrig_Laser_Tcycle.vi"() -> ("output_Laser_Tcycle"=w149:i32)  [unwired: 11 in]
              n49 = call "myRIO_BRig_RT_dataMTrig_Solenoid_RewCalib_nCycle__L.vi"() -> ("output_Solenoid_RewCalib_nCycle__L"=w141:i32)  [unwired: 11 in]
              n50 = call "myRIO_BRig_RT_dataMTrig_Solenoid_RewCalib_nCycle__R.vi"() -> ("output_Solenoid_RewCalib_nCycle__R"=w140:i32)  [unwired: 11 in]
              n51 = call "myRIO_BRig_RT_dataMTrig_Solenoid_Tdelay__L.vi"() -> ("output_Solenoid_Tdelay__L"=w139:i32)  [unwired: 11 in]
              n52 = call "myRIO_BRig_RT_dataMTrig_Solenoid_Tdelay__R.vi"() -> ("output_Solenoid_Tdelay__R"=w138:i32)  [unwired: 11 in]
              n53 = call "myRIO_BRig_RT_dataMTrig_CueLed_Tcycle.vi"() -> ("output_CueLed_Tcycle"=w133:i32)  [unwired: 11 in]
              n54 = local read "MTrig_Solenoid_Tcycle__L"() -> (w150:u16)
              n55 = local read "MTrig_Solenoid_Tcycle__R"() -> (w151:u16)
              n56 = local read "MTrig_Laser_Tcycle"() -> (w136:u16)
              n57 = call "myRIO_BRig_RT_dataMTrig_init.vi"() -> ("output_dataMTrig"=w144:u16[])  [unwired: 5 in]
              n58 = local read "Tcycle_Cue_LED_min"() -> (w132:u16)
              n59 = local read "Tcycle_Cue_Audio_min"() -> (w137:u16)
              n60 = Replace Array Subset(array=w144, new element #1=w150, index #1=w145, new element #2=w151, index #2=w146, new element #3=w137, index #3=w147, new element #4=w137, index #4=w148, new element #5=w136, index #5=w149, new element #6=w135, index #6=w141, new element #7=w135, index #7=w140, new element #8=w135, index #8=w139, new element #9=w135, index #9=w138, new element #10=w132, index #10=w133) -> (w143:u16[])
            }
            frame "UploadSettings_pre" {
              # "When the Host sends settings,\nnot all files send at the same time.\n\nIf RT reads the settings faster\nthan the Host can send them,\nthen we will skip settings.\n\nSolution:\nWait 20 cycles"
              n61 = Increment(x=w159) -> (x+1=w158:u16)
              n62 = Greater?(x=w158, y=u16 20) -> (0:w156:bool)
              n63 = Select(t=myRIO_BRig_RT__Case_NonExp_stateList."UploadSettings_Read_dataExp", s=w156, f=w155) -> (s? t:f=w153:T1)
            }
            frame "UploadSettings_Read_dataExp" {
              # "Grab data but do not act on it yet"
              # "grab dataExp and\nstore it in the\ngeneric data array"
              # "dataExp"
              n64 = call "myRIO_BRig_RT_dataExp_init_details.vi"() -> ("output_dataSize"=w166:i32, "output_dataName"=w169:string)  [unwired: 10 in]
              n65 = call "myRIO_BRig_RT_comm_webdav_uploadReceived_check.vi"("input_dataName"=w169) -> ("output_Iexist"=w168:bool, "output_dataPath"=w167:path)  [unwired: 9 in]
              n66 = case shown="True" w168 {
                tunnel: w167 -> [_ w178]
                tunnel: w166 -> [_ w177]
                tunnel: [_ w176] -> w165
                tunnel: w162 -> [w171 w175]
                tunnel: [w171 w172] -> w161
                frame False {
                }
                frame True {
                  n67 = call "myRIO_BRig_RT_comm_webdav_uploadReceived_read.vi"("input_dataSize"=w177, "input_filePath"=w178) -> ("output_Ivalid"=w176:bool, "output_data"=w174:i64[])  [unwired: 8 in]
                  n68 = To Unsigned Word Integer(number=w174) -> (unsigned 16bit integer=w173:u16[])
                  n69 = Select(t=w173, s=w176, f=w175) -> (s? t:f=w172:u16[])
                }
              }
              n70 = Select(t=myRIO_BRig_RT__Case_NonExp_stateList."UploadSettings_dataExp_1", s=w165, f=myRIO_BRig_RT__Case_NonExp_stateList."UploadSettings_Read_dataLC" ("t")) -> (s? t:f=w160:T1)
            }
            frame "UploadSettings_Read_dataLC" {
              # "Grab data but do not act on it yet"
              # "grab dataLC and\nstore it in the\ngeneric data array"
              # "dataLC"
              n71 = call "myRIO_BRig_RT_dataLC_init_details.vi"() -> ("output_dataSize"=w185:i32, "output_dataName"=w188:string)  [unwired: 10 in]
              n72 = call "myRIO_BRig_RT_comm_webdav_uploadReceived_check.vi"("input_dataName"=w188) -> ("output_Iexist"=w187:bool, "output_dataPath"=w186:path)  [unwired: 9 in]
              n73 = case shown="True" w187 {
                tunnel: w186 -> [_ w197]
                tunnel: w185 -> [_ w196]
                tunnel: [_ w195] -> w184
                tunnel: w181 -> [w190 w194]
                tunnel: [w190 w191] -> w180
                frame False {
                }
                frame True {
                  n74 = call "myRIO_BRig_RT_comm_webdav_uploadReceived_read.vi"("input_dataSize"=w196, "input_filePath"=w197) -> ("output_Ivalid"=w195:bool, "output_data"=w193:i64[])  [unwired: 8 in]
                  n75 = To Unsigned Word Integer(number=w193) -> (unsigned 16bit integer=w192:u16[])
                  n76 = Select(t=w192, s=w195, f=w194) -> (s? t:f=w191:u16[])
                }
              }
              n77 = Select(t=myRIO_BRig_RT__Case_NonExp_stateList."UploadSettings_dataLC_1", s=w184, f=myRIO_BRig_RT__Case_NonExp_stateList."UploadSettings_Read_dataMTrig" ("t")) -> (s? t:f=w179:T1)
            }
            frame "UploadSettings_Read_dataMTrig" {
              # "Grab data but do not act on it yet"
              # "grab dataMTrig and\nstore it in the\ngeneric data array"
              # "dataMTrig"
              n78 = call "myRIO_BRig_RT_dataMTrig_init_details.vi"() -> ("output_dataSize"=w204:i32, "output_dataName"=w207:string)  [unwired: 10 in]
              n79 = call "myRIO_BRig_RT_comm_webdav_uploadReceived_check.vi"("input_dataName"=w207) -> ("output_Iexist"=w206:bool, "output_dataPath"=w205:path)  [unwired: 9 in]
              n80 = case shown="True" w206 {
                tunnel: w205 -> [_ w216]
                tunnel: w204 -> [_ w215]
                tunnel: [_ w214] -> w203
                tunnel: w200 -> [w209 w213]
                tunnel: [w209 w210] -> w199
                frame False {
                }
                frame True {
                  n81 = call "myRIO_BRig_RT_comm_webdav_uploadReceived_read.vi"("input_dataSize"=w215, "input_filePath"=w216) -> ("output_Ivalid"=w214:bool, "output_data"=w212:i64[])  [unwired: 8 in]
                  n82 = To Unsigned Word Integer(number=w212) -> (unsigned 16bit integer=w211:u16[])
                  n83 = Select(t=w211, s=w214, f=w213) -> (s? t:f=w210:u16[])
                }
              }
              n84 = Select(t=myRIO_BRig_RT__Case_NonExp_stateList."UploadSettings_dataMTrig_1", s=w203, f=myRIO_BRig_RT__Case_NonExp_stateList."Idle" ("t")) -> (s? t:f=w198:T1)
            }
            frame "UploadSettings_dataExp_1" {
              # "Cue_max"
              # "Cue_min"
              # "CuePenalty"
              # "Timeout"
              # "Wrong"
              # "Selection"
              # "RewardPost"
              # "Tcycle"
              # "TPB_min_R"
              # "TPB_min_L"
              # "TPB_max_R"
              # "TPB_max_L"
              # "I_trialUntilReward"
              # "ENL_penalty"
              # "ENL_min"
              # "ENL_max"
              # "BUR_max"
              # "BUR_min"
              # "CueCycles"
              # "Audio_Freq_R"
              # "Audio_Freq_L"
              # "Audio_Amp_R"
              # "Audio_Amp_L"
              n85 = call "myRIO_BRig_RT_dataExp_Tcycle_Reward_min_L.vi"() -> ("output_Tcycle_Reward_min_L"=w228:i32)  [unwired: 11 in]
              n86 = call "myRIO_BRig_RT_dataExp_Tcycle_Reward_max_L.vi"() -> ("output_Tcycle_Reward_max_L"=w227:i32)  [unwired: 11 in]
              n87 = call "myRIO_BRig_RT_dataExp_Tcycle_Reward_step_L.vi"() -> ("output_Tcycle_Reward_step_L"=w226:i32)  [unwired: 11 in]
              n88 = call "myRIO_BRig_RT_dataExp_Tcycle_RewardPost.vi"() -> ("output_Tcycle_RewardPost"=w248:i32)  [unwired: 11 in]
              n89 = call "myRIO_BRig_RT_dataExp_CueCycles.vi"() -> ("output_CueCycles"=w276:i32)  [unwired: 11 in]
              n90 = call "myRIO_BRig_RT_dataExp_Audio_amp__R.vi"() -> ("output_Audio_amp__R"=w280:i32)  [unwired: 11 in]
              n91 = call "myRIO_BRig_RT_dataExp_Audio_amp__L.vi"() -> ("output_Audio_amp__L"=w282:i32)  [unwired: 11 in]
              n92 = call "myRIO_BRig_RT_dataExp_BUR_min.vi"() -> ("output_BUR_min"=w273:i32)  [unwired: 11 in]
              n93 = call "myRIO_BRig_RT_dataExp_ENL_min.vi"() -> ("output_ENL_min"=w269:i32)  [unwired: 11 in]
              n94 = call "myRIO_BRig_RT_dataExp_TPB_max__L.vi"() -> ("output_TPB_max__L"=w261:i32)  [unwired: 11 in]
              n95 = call "myRIO_BRig_RT_dataExp_TPB_max__R.vi"() -> ("output_TPB_max__R"=w260:i32)  [unwired: 11 in]
              n96 = call "myRIO_BRig_RT_dataExp_Tcycle_Reward_min_R.vi"() -> ("output_Tcycle_Reward_min_R"=w225:i32)  [unwired: 11 in]
              n97 = call "myRIO_BRig_RT_dataExp_Tcycle_Reward_max_R.vi"() -> ("output_Tcycle_Reward_max_R"=w224:i32)  [unwired: 11 in]
              n98 = call "myRIO_BRig_RT_dataExp_Tcycle_Reward_step_R.vi"() -> ("output_Tcycle_Reward_step_R"=w223:i32)  [unwired: 11 in]
              n99 = call "myRIO_BRig_RT_dataExp_ENL_penalty.vi"() -> ("output_ENL_penalty"=w268:i32)  [unwired: 11 in]
              n100 = call "myRIO_BRig_RT_dataExp_Tcycle_Selection.vi"() -> ("output_Tcycle_Selection"=w247:i32)  [unwired: 11 in]
              n101 = call "myRIO_BRig_RT_dataExp_Tcycle_Wrong.vi"() -> ("output_Tcycle_Wrong"=w246:i32)  [unwired: 11 in]
              n102 = call "myRIO_BRig_RT_dataExp_Tcycle_Timeout.vi"() -> ("output_Tcycle_Timeout"=w242:i32)  [unwired: 11 in]
              n103 = call "myRIO_BRig_RT_dataExp_Audio_freq__L.vi"() -> ("output_Audio_freq__L"=w278:i32)  [unwired: 11 in]
              n104 = call "myRIO_BRig_RT_dataExp_Audio_freq__R.vi"() -> ("output_Audio_freq__R"=w277:i32)  [unwired: 11 in]
              n105 = call "myRIO_BRig_RT_dataExp_BUR_max.vi"() -> ("output_BUR_max"=w274:i32)  [unwired: 11 in]
              n106 = call "myRIO_BRig_RT_dataExp_ENL_max.vi"() -> ("output_ENL_max"=w270:i32)  [unwired: 11 in]
              n107 = call "myRIO_BRig_RT_dataExp_ItrialUntilReward.vi"() -> ("output_I_trialUntilReward"=w264:i32)  [unwired: 11 in]
              n108 = call "myRIO_BRig_RT_dataExp_TPB_min__L.vi"() -> ("output_TPB_min__L"=w259:i32)  [unwired: 11 in]
              n109 = call "myRIO_BRig_RT_dataExp_TPB_min__R.vi"() -> ("output_TPB_min__R"=w258:i32)  [unwired: 11 in]
              n110 = call "myRIO_BRig_RT_dataExp_Tcycle_Cue1Penalty_Audio.vi"() -> ("output_Tcycle_Cue1Penalty_Audio"=w240:i32)  [unwired: 11 in]
              n111 = call "myRIO_BRig_RT_dataExp_Tcycle_Cue1_Audio_min.vi"() -> ("output_Tcycle_Cue1_Audio_min"=w238:i32)  [unwired: 11 in]
              n112 = call "myRIO_BRig_RT_dataExp_Tcycle_Cue1_Audio_max.vi"() -> ("output_Tcycle_Cue1_Audio_max"=w236:i32)  [unwired: 11 in]
              n113 = call "myRIO_BRig_RT_dataExp_Tcycle_Cue1Penalty_LED.vi"() -> ("output_Tcycle_Cue1Penalty_LED"=w234:i32)  [unwired: 11 in]
              n114 = call "myRIO_BRig_RT_dataExp_Tcycle_Cue1_LED_min.vi"() -> ("output_Tcycle_Cue1_LED_min"=w233:i32)  [unwired: 11 in]
              n115 = call "myRIO_BRig_RT_dataExp_Tcycle_Cue1_LED_max.vi"() -> ("output_Tcycle_Cue1_LED_max"=w232:i32)  [unwired: 11 in]
              n116 = Index Array(array=w249, index #1=w282, index #2=w280, index #3=w278, index #4=w277, index #5=w276, index #6=w274, index #7=w273, index #8=w270, index #9=w269, index #10=w268, index #11=w264, index #12=w261, index #13=w260, index #14=w259, index #15=w258, index #16=w248, index #17=w247, index #18=w246, index #19=w242, index #20=w240, index #21=w238, index #22=w236, index #23=w234, index #24=w233, index #25=w232, index #26=w228, index #27=w227, index #28=w226, index #29=w225, index #30=w224, index #31=w223) -> (element #1=w281:u16, element #2=w279:u16, element #3=w252:u16, element #4=w251:u16, element #5=w275:u16, element #6=w272:u16, element #7=w271:u16, element #8=w267:u16, element #9=w266:u16, element #10=w265:u16, element #11=w262:u16, element #12=w257:u16, element #13=w256:u16, element #14=w255:u16, element #15=w254:u16, element #16=w245:u16, element #17=w244:u16, element #18=w243:u16, element #19=w241:u16, element #20=w239:u16, element #21=w237:u16, element #22=w235:u16, element #23=w231:u16, element #24=w230:u16, element #25=w229:u16, element #26=w222:u16, element #27=w221:u16, element #28=w220:u16, element #29=w219:u16, element #30=w218:u16, element #31=w217:u16)
              n117 = local write "Tcycle_CuePenalty_LED"(w231) -> ()
              n118 = local write "Tcycle_Cue_LED_min"(w230) -> ()
              n119 = local write "Tcycle_Cue_LED_max"(w229) -> ()
              n120 = local write "Tcycle_Selection"(w244) -> ()
              n121 = local write "Tcycle_Wrong"(w243) -> ()
              n122 = local write "Tcycle_Timeout"(w241) -> ()
              n123 = local write "Audio_Amp__L"(w281) -> ()
              n124 = local write "Audio_Amp__R"(w279) -> ()
              n125 = local write "Tcycle_Reward_min_L"(w222) -> ()
              n126 = local write "Tcycle_Reward_max_L"(w221) -> ()
              n127 = local write "Tcycle_Reward_step_L"(w220) -> ()
              n128 = local write "Tcycle_Reward_min_L"(w219) -> ()
              n129 = local write "Tcycle_Reward_max_L"(w218) -> ()
              n130 = local write "Tcycle_Reward_step_L"(w217) -> ()
              n131 = local write "Tcycle_ENLPenalty"(w265) -> ()
              n132 = local write "Tcycle_ENL_max"(w267) -> ()
              n133 = local write "TpB_Min_L"(w255) -> ()
              n134 = local write "TpB_Min_R"(w254) -> ()
              n135 = local write "Tcycle_CuePenalty_Audio"(w239) -> ()
              n136 = local write "Tcycle_Cue_Audio_min"(w237) -> ()
              n137 = local write "Tcycle_Cue_Audio_max"(w235) -> ()
              n138 = To Unsigned Byte Integer(number=w252) -> (unsigned 8bit integer=w253:u8)
              n139 = To Unsigned Byte Integer(number=w251) -> (unsigned 8bit integer=w250:u8)
              n140 = Not Equal To 0?(x=w262) -> (x != 0?=w263:bool)
              n141 = local write "Tcycle_RewardPost"(w245) -> ()
              n142 = local write "CueCycles"(w275) -> ()
              n143 = local write "BUR_min"(w271) -> ()
              n144 = local write "BUR_max"(w272) -> ()
              n145 = local write "Tcycle_ENL_min"(w266) -> ()
              n146 = local write "TpB_Max_L"(w257) -> ()
              n147 = local write "TpB_Max_R"(w256) -> ()
              n148 = local write "TrialUntilReward"(w263) -> ()
              n149 = local write "Audio_Freq__L"(w253) -> ()
              n150 = local write "Audio_Freq__R"(w250) -> ()
            }
            frame "UploadSettings_dataExp_2" {
              w304 = 100.0 ("y")
              n151 = call "myRIO_BRig_RT_dataExp_FPGA_f_count2ms.vi"() -> ("output_FPGA_f_count2ms"=w365:i32)  [unwired: 11 in]
              n152 = call "myRIO_BRig_RT_dataExp_laser1_Freq.vi"() -> ("output_laser1_Freq"=w353:i32)  [unwired: 11 in]
              n153 = call "myRIO_BRig_RT_dataExp_laser1_duration.vi"() -> ("output_laser1_duration"=w352:i32)  [unwired: 11 in]
              n154 = call "myRIO_BRig_RT_dataExp_laser1_Tpeak.vi"() -> ("output_laser1_Tpeak"=w351:i32)  [unwired: 11 in]
              n155 = call "myRIO_BRig_RT_dataExp_laser1_Tshutter.vi"() -> ("output_laser1_Tshutter"=w350:i32)  [unwired: 11 in]
              n156 = call "myRIO_BRig_RT_dataExp_laser1_Power_min.vi"() -> ("output_laser1_Power_min"=w349:i32)  [unwired: 11 in]
              n157 = call "myRIO_BRig_RT_dataExp_laser1_Power_max.vi"() -> ("output_laser1_Power_max"=w348:i32)  [unwired: 11 in]
              n158 = call "myRIO_BRig_RT_dataExp_laser1_Power_step.vi"() -> ("output_laser1_Power_step"=w347:i32)  [unwired: 11 in]
              n159 = call "myRIO_BRig_RT_dataExp_Cue1Param_CueType_Switch.vi"() -> ("output_Cue1Param_CueType_Switch"=w298:i32)  [unwired: 11 in]
              n160 = call "myRIO_BRig_RT_dataExp_Cue1Param_AudioLed_Count_Switch.vi"() -> ("output_Cue1Param_AudioLed_Count_Switch"=w297:i32)  [unwired: 11 in]
              n161 = call "myRIO_BRig_RT_dataExp_Cue1Param_AudioLed_Probability_Switch.vi"() -> ("output_Cue1Param_AudioLed_Probability_Switch"=w296:i32)  [unwired: 11 in]
              n162 = call "myRIO_BRig_RT_dataExp_SolenoidProbability_L.vi"() -> ("output_SolenoidProbability_L"=w300:i32)  [unwired: 11 in]
              n163 = call "myRIO_BRig_RT_dataExp_SolenoidProbability_R.vi"() -> ("output_SolenoidProbability_R"=w299:i32)  [unwired: 11 in]
              n164 = call "myRIO_BRig_RT_dataExp_Cue1Param_CueType_NS.vi"() -> ("output_Cue1Param_CueType_NS"=w295:i32)  [unwired: 11 in]
              n165 = call "myRIO_BRig_RT_dataExp_Cue1Param_AudioLed_Count_NS.vi"() -> ("output_Cue1Param_AudioLed_Count_NS"=w294:i32)  [unwired: 11 in]
              n166 = call "myRIO_BRig_RT_dataExp_Cue1Param_AudioLed_Probability_NS.vi"() -> ("output_Cue1Param_AudioLed_Probability_NS"=w293:i32)  [unwired: 11 in]
              n167 = call "myRIO_BRig_RT_dataExp_laser2_Freq.vi"() -> ("output_laser2_Freq"=w346:i32)  [unwired: 11 in]
              n168 = call "myRIO_BRig_RT_dataExp_laser2_duration.vi"() -> ("output_laser2_duration"=w345:i32)  [unwired: 11 in]
              n169 = call "myRIO_BRig_RT_dataExp_laser2_Tpeak.vi"() -> ("output_laser2_Tpeak"=w344:i32)  [unwired: 11 in]
              n170 = call "myRIO_BRig_RT_dataExp_laser2_Tshutter.vi"() -> ("output_laser2_Tshutter"=w343:i32)  [unwired: 11 in]
              n171 = call "myRIO_BRig_RT_dataExp_laser2_Power_min.vi"() -> ("output_laser2_Power_min"=w342:i32)  [unwired: 11 in]
              n172 = call "myRIO_BRig_RT_dataExp_laser2_Power_max.vi"() -> ("output_laser2_Power_max"=w341:i32)  [unwired: 11 in]
              n173 = call "myRIO_BRig_RT_dataExp_laser2_Power_step.vi"() -> ("output_laser2_Power_step"=w340:i32)  [unwired: 11 in]
              n174 = call "myRIO_BRig_RT_dataExp_CueLed_Freq.vi"() -> ("output_CueLed_Freq"=w309:i32)  [unwired: 11 in]
              n175 = call "myRIO_BRig_RT_dataExp_CueLed_Tpeak.vi"() -> ("output_CueLed_Tpeak"=w302:i32)  [unwired: 11 in]
              n176 = Index Array(array=w366, index #1=w365, index #2=w353, index #3=w352, index #4=w351, index #5=w350, index #6=w349, index #7=w348, index #8=w347, index #9=w346, index #10=w345, index #11=w344, index #12=w343, index #13=w342, index #14=w341, index #15=w340, index #16=w309, index #17=w302, index #18=w300, index #19=w299, index #20=w298, index #21=w297, index #22=w296, index #23=w295, index #24=w294, index #25=w293) -> (element #1=w364:u16, element #2=w339:u16, element #3=w338:u16, element #4=w337:u16, element #5=w336:u16, element #6=w335:u16, element #7=w325:u16, element #8=w324:u16, element #9=w320:u16, element #10=w319:u16, element #11=w318:u16, element #12=w317:u16, element #13=w316:u16, element #14=w311:u16, element #15=w310:u16, element #16=w303:u16, element #17=w301:u16, element #18=w292:u16, element #19=w291:u16, element #20=w290:u16, element #21=w289:u16, element #22=w288:u16, element #23=w287:u16, element #24=w286:u16, element #25=w285:u16)
              n177 = local write "Cue1Param_CueType_Switch"(w290) -> ()
              n178 = local write "Cue1Param_AudioLed_Count_Switch"(w289) -> ()
              n179 = local write "Cue1Param_AudioLed_Probability_Switch"(w288) -> ()
              n180 = local write "Cue1Param_CueType_NS"(w287) -> ()
              n181 = local write "Cue1Param_AudioLed_Count_NS"(w286) -> ()
              n182 = local write "Cue1Param_AudioLed_Probability_NS"(w285) -> ()
              n183 = To Double Precision Float(number=w364) -> (double precision float=w363:dbl)
              n184 = To Double Precision Float(number=w339) -> (double precision float=w361:dbl)
              n185 = To Double Precision Float(number=w337) -> (double precision float=w358:dbl)
              n186 = To Double Precision Float(number=w336) -> (double precision float=w357:dbl)
              n187 = To Double Precision Float(number=w335) -> (double precision float=w359:dbl)
              n188 = To Double Precision Float(number=w325) -> (double precision float=w330:dbl)
              n189 = To Double Precision Float(number=w324) -> (double precision float=w326:dbl)
              n190 = To Double Precision Float(number=w320) -> (double precision float=w331:dbl)
              n191 = To Double Precision Float(number=w318) -> (double precision float=w333:dbl)
              n192 = To Double Precision Float(number=w317) -> (double precision float=w334:dbl)
              n193 = To Double Precision Float(number=w316) -> (double precision float=w332:dbl)
              n194 = To Double Precision Float(number=w311) -> (double precision float=w314:dbl)
              n195 = To Double Precision Float(number=w310) -> (double precision float=w315:dbl)
              n196 = To Double Precision Float(number=w303) -> (double precision float=w308:dbl)
              n197 = To Double Precision Float(number=w301) -> (double precision float=w307:dbl)
              n198 = local write "SolenoidProbability_L"(w292) -> ()
              n199 = local write "SolenoidProbability_R"(w291) -> ()
              n200 = Divide(x=w363, y=w304) -> (x/y=w362:dbl)
              n201 = Divide(x=w361, y=w304) -> (x/y=w360:dbl)
              n202 = Divide(x=w358, y=w304) -> (x/y=w355:dbl)
              n203 = Divide(x=w357, y=w304) -> (x/y=w354:dbl)
              n204 = Divide(x=w359, y=w304) -> (x/y=w356:dbl)
              n205 = Divide(x=w330, y=w304) -> (x/y=w328:dbl)
              n206 = Divide(x=w326, y=w304) -> (x/y=w327:dbl)
              n207 = Divide(x=w331, y=w304) -> (x/y=w329:dbl)
              n208 = Divide(x=w333, y=w304) -> (x/y=w323:dbl)
              n209 = Divide(x=w334, y=w304) -> (x/y=w322:dbl)
              n210 = Divide(x=w332, y=w304) -> (x/y=w321:dbl)
              n211 = Divide(x=w314, y=w304) -> (x/y=w313:dbl)
              n212 = Divide(x=w315, y=w304) -> (x/y=w312:dbl)
              n213 = Divide(x=w308, y=w304) -> (x/y=w306:dbl)
              n214 = Divide(x=w307, y=w304) -> (x/y=w305:dbl)
              n215 = local write "FPGA_count2ms"(w362) -> ()
              n216 = local write "Laser_Freq_l1"(w360) -> ()
              n217 = local write "Laser_duration_l1"(w338) -> ()
              n218 = local write "Laser_Tpeak_l1"(w355) -> ()
              n219 = local write "Laser_Tshutter_l1"(w354) -> ()
              n220 = local write "Laser_power_min_l1"(w356) -> ()
              n221 = local write "Laser_power_max_l1"(w328) -> ()
              n222 = local write "Laser_power_step_l1"(w327) -> ()
              n223 = local write "Laser_Freq_l2"(w329) -> ()
              n224 = local write "Laser_duration_l2"(w319) -> ()
              n225 = local write "Laser_Tpeak_l2"(w323) -> ()
              n226 = local write "Laser_Tshutter_l2"(w322) -> ()
              n227 = local write "Laser_power_min_l2"(w321) -> ()
              n228 = local write "Laser_power_max_l2"(w313) -> ()
              n229 = local write "Laser_power_step_l2"(w312) -> ()
              n230 = local write "CueLed_Freq"(w306) -> ()
              n231 = local write "CueLed_Tpeak"(w305) -> ()
            }
            frame "UploadSettings_dataLC_1" {
              # "Cue1_delayOpt_NonSwitch"
              # "ENL1_delayOpt_NonSwitch"
              # "Cue1_delayOpt_Switch"
              # "ENL1_delayOpt_Switch"
              # "Count"
              # "Tdelay"
              # "Prob"
              # "OnOff"
              # "Block"
              # "Count"
              # "Tdelay"
              # "Prob"
              # "OnOff"
              # "Block"
              # "Count"
              # "Tdelay"
              # "Prob"
              # "OnOff"
              # "Block"
              # "ENL1 Switch"
              # "Cue1 NonSwitch"
              # "Cue1 Switch"
              # "ENL1 NonSwitch"
              # "Count"
              # "Tdelay"
              # "Prob"
              # "OnOff"
              # "Block"
              n232 = call "myRIO_BRig_RT_dataLC_ENL1_OnOff_Switch_l1.vi"() -> ("output_ENL1_OnOff_Switch_l1"=w420:i32)  [unwired: 11 in]
              n233 = call "myRIO_BRig_RT_dataLC_ENL1_Tdelay_Switch_l1.vi"() -> ("output_ENL1_Tdelay_Switch_l1"=w419:i32)  [unwired: 11 in]
              n234 = call "myRIO_BRig_RT_dataLC_ENL1_Block_Switch_l1.vi"() -> ("output_ENL1_Block_Switch_l1"=w418:i32)  [unwired: 11 in]
              n235 = call "myRIO_BRig_RT_dataLC_ENL1_Count_Switch_l1.vi"() -> ("output_ENL1_Count_Switch_l1"=w417:i32)  [unwired: 11 in]
              n236 = call "myRIO_BRig_RT_dataLC_ENL1_Probability_Switch_l1.vi"() -> ("output_ENL1_Probability_Switch_l1"=w416:i32)  [unwired: 11 in]
              n237 = call "myRIO_BRig_RT_dataLC_ENL1_OnOff_NS_l1.vi"() -> ("output_ENL1_OnOff_NS_l1"=w415:i32)  [unwired: 11 in]
              n238 = call "myRIO_BRig_RT_dataLC_ENL1_Tdelay_NS_l1.vi"() -> ("output_ENL1_Tdelay_NS_l1"=w414:i32)  [unwired: 11 in]
              n239 = call "myRIO_BRig_RT_dataLC_ENL1_Block_NS_l1.vi"() -> ("output_ENL1_All_Block"=w413:i32)  [unwired: 11 in]
              n240 = call "myRIO_BRig_RT_dataLC_ENL1_Count_NS_l1.vi"() -> ("output_ENL1_Count_NS_l1"=w412:i32)  [unwired: 11 in]
              n241 = call "myRIO_BRig_RT_dataLC_ENL1_Probability_NS_l1.vi"() -> ("output_ENL1_Probability_NS_l1"=w411:i32)  [unwired: 11 in]
              n242 = call "myRIO_BRig_RT_dataLC_Cue1_OnOff_Switch_l1.vi"() -> ("output_Cue1_OnOff_Switch_l1"=w410:i32)  [unwired: 11 in]
              n243 = call "myRIO_BRig_RT_dataLC_Cue1_Tdelay_Switch_l1.vi"() -> ("output_Cue1_Tdelay_Switch_l1"=w409:i32)  [unwired: 11 in]
              n244 = call "myRIO_BRig_RT_dataLC_Cue1_Block_Switch_l1.vi"() -> ("output_Cue1_Block_Switch_l1"=w408:i32)  [unwired: 11 in]
              n245 = call "myRIO_BRig_RT_dataLC_Cue1_Count_Switch_l1.vi"() -> ("output_Cue1_Count_Switch_l1"=w407:i32)  [unwired: 11 in]
              n246 = call "myRIO_BRig_RT_dataLC_Cue1_Probability_Switch_l1.vi"() -> ("output_Cue1_Probability_Switch_l1"=w406:i32)  [unwired: 11 in]
              n247 = call "myRIO_BRig_RT_dataLC_Cue1_OnOff_NS_l1.vi"() -> ("output_Cue1_OnOff_NS_l1"=w405:i32)  [unwired: 11 in]
              n248 = call "myRIO_BRig_RT_dataLC_Cue1_Tdelay_NS_l1.vi"() -> ("output_Cue1_Tdelay_NS_l1"=w404:i32)  [unwired: 11 in]
              n249 = call "myRIO_BRig_RT_dataLC_Cue1_Block_NS_l1.vi"() -> ("output_Cue1_Block_NS_l1"=w403:i32)  [unwired: 11 in]
              n250 = call "myRIO_BRig_RT_dataLC_Cue1_Count_NS_l1.vi"() -> ("output_Cue1_Count_NS_l1"=w402:i32)  [unwired: 11 in]
              n251 = call "myRIO_BRig_RT_dataLC_Cue1_Probability_NS_l1.vi"() -> ("output_Cue1_l1_All_Probability"=w401:i32)  [unwired: 11 in]
              n252 = call "myRIO_BRig_RT_dataLC_ENL1_delayOpt_Switch_l1.vi"() -> ("output_ENL1_delayOpt_Switch_l1"=w380:i32)  [unwired: 11 in]
              n253 = call "myRIO_BRig_RT_dataLC_ENL1_delayOpt_NS_l1.vi"() -> ("output_ENL1_delayOpt_NS_l1"=w379:i32)  [unwired: 11 in]
              n254 = call "myRIO_BRig_RT_dataLC_Cue1_delayOpt_Switch_l1.vi"() -> ("output_Cue1_delayOpt_Switch_l1"=w378:i32)  [unwired: 11 in]
              n255 = call "myRIO_BRig_RT_dataLC_Cue1_delayOpt_NS_l1.vi"() -> ("output_Cue1_delayOpt_NS_l1"=w377:i32)  [unwired: 11 in]
              n256 = Index Array(array=w422, index #1=w420, index #2=w419, index #3=w418, index #4=w417, index #5=w416, index #6=w415, index #7=w414, index #8=w413, index #9=w412, index #10=w411, index #11=w410, index #12=w409, index #13=w408, index #14=w407, index #15=w406, index #16=w405, index #17=w404, index #18=w403, index #19=w402, index #20=w401, index #21=w380, index #22=w379, index #23=w378, index #24=w377) -> (element #1=w400:u16, element #2=w399:u16, element #3=w398:u16, element #4=w397:u16, element #5=w396:u16, element #6=w395:u16, element #7=w394:u16, element #8=w393:u16, element #9=w392:u16, element #10=w391:u16, element #11=w390:u16, element #12=w389:u16, element #13=w388:u16, element #14=w387:u16, element #15=w386:u16, element #16=w385:u16, element #17=w384:u16, element #18=w383:u16, element #19=w382:u16, element #20=w381:u16, element #21=w372:u16, element #22=w371:u16, element #23=w370:u16, element #24=w369:u16)
              n257 = Not Equal To 0?(x=w400) -> (x != 0?=w424:bool)
              n258 = Not Equal To 0?(x=w395) -> (x != 0?=w423:bool)
              n259 = Not Equal To 0?(x=w390) -> (x != 0?=w426:bool)
              n260 = Not Equal To 0?(x=w385) -> (x != 0?=w425:bool)
              n261 = Not Equal To 0?(x=w372) -> (x != 0?=w374:bool)
              n262 = Not Equal To 0?(x=w371) -> (x != 0?=w375:bool)
              n263 = Not Equal To 0?(x=w370) -> (x != 0?=w376:bool)
              n264 = Not Equal To 0?(x=w369) -> (x != 0?=w373:bool)
              n265 = local write "LC_ENL1_OnOff_Switch_l1"(w424) -> ()
              n266 = local write "LC_ENL1_Tdelay_Switch_l1"(w399) -> ()
              n267 = local write "LC_ENL1_Block_Switch_l1"(w398) -> ()
              n268 = local write "LC_ENL1_Count_Switch_l1"(w397) -> ()
              n269 = local write "LC_ENL1_Probability_Switch_l1"(w396) -> ()
              n270 = local write "LC_ENL1_OnOff_NS_l1"(w423) -> ()
              n271 = local write "LC_ENL1_Tdelay_NS_l1"(w394) -> ()
              n272 = local write "LC_ENL1_Block_NS_l1"(w393) -> ()
              n273 = local write "LC_ENL1_Count_NS_l1"(w392) -> ()
              n274 = local write "LC_ENL1_Probability_NS_l1"(w391) -> ()
              n275 = local write "LC_Cue1_OnOff_Switch_l1"(w426) -> ()
              n276 = local write "LC_Cue1_Tdelay_Switch_l1"(w389) -> ()
              n277 = local write "LC_Cue1_Block_Switch_l1"(w388) -> ()
              n278 = local write "LC_Cue1_Count_Switch_l1"(w387) -> ()
              n279 = local write "LC_Cue1_Probability_Switch_l1"(w386) -> ()
              n280 = local write "LC_Cue1_OnOff_NS_l1"(w425) -> ()
              n281 = local write "LC_Cue1_Tdelay_NS_l1"(w384) -> ()
              n282 = local write "LC_Cue1_Block_NS_l1"(w383) -> ()
              n283 = local write "LC_Cue1_Count_NS_l1"(w382) -> ()
              n284 = local write "LC_Cue1_Probability_NS_l1"(w381) -> ()
              n285 = local write "LC_ENL1_delayOpt_Switch_l1"(w374) -> ()
              n286 = local write "LC_ENL1_delayOpt_NS_l1"(w375) -> ()
              n287 = local write "LC_Cue1_delayOpt_Switch_l1"(w376) -> ()
              n288 = local write "LC_Cue1_delayOpt_NS_l1"(w373) -> ()
            }
            frame "UploadSettings_dataLC_3" {
              # "Cue1_delayOpt_NonSwitch"
              # "ENL1_delayOpt_NonSwitch"
              # "Cue1_delayOpt_Switch"
              # "ENL1_delayOpt_Switch"
              # "Count"
              # "Tdelay"
              # "Prob"
              # "OnOff"
              # "Block"
              # "Count"
              # "Tdelay"
              # "Prob"
              # "OnOff"
              # "Block"
              # "Count"
              # "Tdelay"
              # "Prob"
              # "OnOff"
              # "Block"
              # "ENL1 Switch"
              # "Cue1 NonSwitch"
              # "Cue1 Switch"
              # "ENL1 NonSwitch"
              # "Count"
              # "Tdelay"
              # "Prob"
              # "OnOff"
              # "Block"
              n289 = call "myRIO_BRig_RT_dataLC_ENL1_OnOff_Switch_l2.vi"() -> ("output_ENL1_OnOff_Switch_l2"=w447:i32)  [unwired: 11 in]
              n290 = call "myRIO_BRig_RT_dataLC_ENL1_Tdelay_Switch_l2.vi"() -> ("output_ENL1_Tdelay_Switch_l2"=w448:i32)  [unwired: 11 in]
              n291 = call "myRIO_BRig_RT_dataLC_ENL1_Block_Switch_l2.vi"() -> ("output_ENL1_Block_Switch_l2"=w449:i32)  [unwired: 11 in]
              n292 = call "myRIO_BRig_RT_dataLC_ENL1_Count_Switch_l2.vi"() -> ("output_ENL1_Count_Switch_l2"=w450:i32)  [unwired: 11 in]
              n293 = call "myRIO_BRig_RT_dataLC_ENL1_Probability_Switch_l2.vi"() -> ("output_ENL1_Probability_Switch_l2"=w451:i32)  [unwired: 11 in]
              n294 = call "myRIO_BRig_RT_dataLC_ENL1_OnOff_NS_l2.vi"() -> ("output_ENL1_OnOff_NS_l2"=w442:i32)  [unwired: 11 in]
              n295 = call "myRIO_BRig_RT_dataLC_ENL1_Tdelay_NS_l2.vi"() -> ("output_ENL1_Tdelay_NS_l2"=w443:i32)  [unwired: 11 in]
              n296 = call "myRIO_BRig_RT_dataLC_ENL1_Block_NS_l2.vi"() -> ("output_ENL1_Block_NS_l2"=w444:i32)  [unwired: 11 in]
              n297 = call "myRIO_BRig_RT_dataLC_ENL1_Count_NS_l2.vi"() -> ("output_ENL1_Count_NS_l2"=w445:i32)  [unwired: 11 in]
              n298 = call "myRIO_BRig_RT_dataLC_ENL1_Probability_NS_l2.vi"() -> ("output_ENL1_Probability_NS_l2"=w446:i32)  [unwired: 11 in]
              n299 = call "myRIO_BRig_RT_dataLC_Cue1_OnOff_Switch_l2.vi"() -> ("output_Cue1_OnOff_Switch_l2"=w437:i32)  [unwired: 11 in]
              n300 = call "myRIO_BRig_RT_dataLC_Cue1_Tdelay_Switch_l2.vi"() -> ("output_Cue1_Tdelay_Switch_l2"=w438:i32)  [unwired: 11 in]
              n301 = call "myRIO_BRig_RT_dataLC_Cue1_Block_Switch_l2.vi"() -> ("output_Cue1_Block_Switch_l2"=w439:i32)  [unwired: 11 in]
              n302 = call "myRIO_BRig_RT_dataLC_Cue1_Count_Switch_l2.vi"() -> ("output_Cue1_Count_Switch_l2"=w440:i32)  [unwired: 11 in]
              n303 = call "myRIO_BRig_RT_dataLC_Cue1_Probability_Switch_l2.vi"() -> ("output_Cue1_l2_First_Probability"=w441:i32)  [unwired: 11 in]
              n304 = call "myRIO_BRig_RT_dataLC_Cue1_OnOff_NS_l2.vi"() -> ("output_Cue1_OnOff_NS_l2"=w432:i32)  [unwired: 11 in]
              n305 = call "myRIO_BRig_RT_dataLC_Cue1_Tdelay_NS_l2.vi"() -> ("output_Cue1_Tdelay_NS_l2"=w433:i32)  [unwired: 11 in]
              n306 = call "myRIO_BRig_RT_dataLC_Cue1_Block_NS_l2.vi"() -> ("output_Cue1_Block_NS_l2"=w434:i32)  [unwired: 11 in]
              n307 = call "myRIO_BRig_RT_dataLC_Cue1_Count_NS_l2.vi"() -> ("output_Cue1_Count_NS_l2"=w435:i32)  [unwired: 11 in]
              n308 = call "myRIO_BRig_RT_dataLC_Cue1_Probability_NS_l2.vi"() -> ("output_Cue1_l2_All_Probability"=w436:i32)  [unwired: 11 in]
              n309 = call "myRIO_BRig_RT_dataLC_ENL1_delayOpt_Switch_l2.vi"() -> ("output_ENL1_delayOpt_Switch_l2"=w428:i32)  [unwired: 11 in]
              n310 = call "myRIO_BRig_RT_dataLC_ENL1_delayOpt_NS_l2.vi"() -> ("output_ENL1_delayOpt_NS_l2"=w429:i32)  [unwired: 11 in]
              n311 = call "myRIO_BRig_RT_dataLC_Cue1_delayOpt_Switch_l2.vi"() -> ("output_Cue1_delayOpt_Switch_l2"=w430:i32)  [unwired: 11 in]
              n312 = call "myRIO_BRig_RT_dataLC_Cue1_delayOpt_NS_l2.vi"() -> ("output_Cue1_delayOpt_NS_l2"=w431:i32)  [unwired: 11 in]
              n313 = Index Array(array=w481, index #1=w447, index #2=w448, index #3=w449, index #4=w450, index #5=w451, index #6=w442, index #7=w443, index #8=w444, index #9=w445, index #10=w446, index #11=w437, index #12=w438, index #13=w439, index #14=w440, index #15=w441, index #16=w432, index #17=w433, index #18=w434, index #19=w435, index #20=w436, index #21=w428, index #22=w429, index #23=w430, index #24=w431) -> (element #1=w479:u16, element #2=w478:u16, element #3=w477:u16, element #4=w476:u16, element #5=w475:u16, element #6=w474:u16, element #7=w473:u16, element #8=w472:u16, element #9=w471:u16, element #10=w470:u16, element #11=w469:u16, element #12=w468:u16, element #13=w467:u16, element #14=w466:u16, element #15=w465:u16, element #16=w464:u16, element #17=w463:u16, element #18=w462:u16, element #19=w461:u16, element #20=w460:u16, element #21=w455:u16, element #22=w454:u16, element #23=w453:u16, element #24=w452:u16)
              n314 = Not Equal To 0?(x=w479) -> (x != 0?=w483:bool)
              n315 = Not Equal To 0?(x=w474) -> (x != 0?=w482:bool)
              n316 = Not Equal To 0?(x=w469) -> (x != 0?=w485:bool)
              n317 = Not Equal To 0?(x=w464) -> (x != 0?=w484:bool)
              n318 = Not Equal To 0?(x=w455) -> (x != 0?=w457:bool)
              n319 = Not Equal To 0?(x=w454) -> (x != 0?=w458:bool)
              n320 = Not Equal To 0?(x=w453) -> (x != 0?=w459:bool)
              n321 = Not Equal To 0?(x=w452) -> (x != 0?=w456:bool)
              n322 = local write "LC_ENL1_OnOff_Switch_l2"(w483) -> ()
              n323 = local write "LC_ENL1_Tdelay_Switch_l2"(w478) -> ()
              n324 = local write "LC_ENL1_Block_Switch_l2"(w477) -> ()
              n325 = local write "LC_ENL1_Count_Switch_l2"(w476) -> ()
              n326 = local write "LC_ENL1_Probability_Switch_l2"(w475) -> ()
              n327 = local write "LC_ENL1_OnOff_NS_l2"(w482) -> ()
              n328 = local write "LC_ENL1_Tdelay_NS_l2"(w473) -> ()
              n329 = local write "LC_ENL1_Block_NS_l2"(w472) -> ()
              n330 = local write "LC_ENL1_Count_NS_l2"(w471) -> ()
              n331 = local write "LC_ENL1_Probability_NS_l2"(w470) -> ()
              n332 = local write "LC_Cue1_OnOff_Switch_l2"(w485) -> ()
              n333 = local write "LC_Cue1_Tdelay_Switch_l2"(w468) -> ()
              n334 = local write "LC_Cue1_Block_Switch_l2"(w467) -> ()
              n335 = local write "LC_Cue1_Count_Switch_l2"(w466) -> ()
              n336 = local write "LC_Cue1_Probability_Switch_l2"(w465) -> ()
              n337 = local write "LC_Cue1_OnOff_NS_l2"(w484) -> ()
              n338 = local write "LC_Cue1_Tdelay_NS_l2"(w463) -> ()
              n339 = local write "LC_Cue1_Block_NS_l2"(w462) -> ()
              n340 = local write "LC_Cue1_Count_NS_l2"(w461) -> ()
              n341 = local write "LC_Cue1_Probability_NS_l2"(w460) -> ()
              n342 = local write "LC_ENL1_delayOpt_Switch_l2"(w457) -> ()
              n343 = local write "LC_ENL1_delayOpt_NS_l2"(w458) -> ()
              n344 = local write "LC_Cue1_delayOpt_Switch_l2"(w459) -> ()
              n345 = local write "LC_Cue1_delayOpt_NS_l2"(w456) -> ()
            }
            frame "UploadSettings_dataLC_2" {
              # "Count"
              # "Tdelay"
              # "Prob"
              # "OnOff"
              # "Block"
              # "Selection NonSwitch"
              # "Count"
              # "Tdelay"
              # "Prob"
              # "OnOff"
              # "Block"
              # "Selection Switch"
              # "Trial"
              # "Tdelay"
              # "Prob"
              # "OnOff"
              # "Block"
              # "Wrong"
              # "Reward"
              # "Trial"
              # "Tdelay"
              # "Prob"
              # "OnOff"
              # "Block"
              n346 = call "myRIO_BRig_RT_dataLC_Reward_OnOff_l1.vi"() -> ("output_Reward_OnOff_l1"=w528:i32)  [unwired: 11 in]
              n347 = call "myRIO_BRig_RT_dataLC_Reward_Tdelay_l1.vi"() -> ("output_Reward_Tdelay_l1"=w527:i32)  [unwired: 11 in]
              n348 = call "myRIO_BRig_RT_dataLC_Reward_Block_l1.vi"() -> ("output_Reward_Block_l1"=w526:i32)  [unwired: 11 in]
              n349 = call "myRIO_BRig_RT_dataLC_Reward_Trial_l1.vi"() -> ("output_Reward_Trial_l1"=w525:i32)  [unwired: 11 in]
              n350 = call "myRIO_BRig_RT_dataLC_Reward_Probability_l1.vi"() -> ("output_Reward_Probability_l1"=w524:i32)  [unwired: 11 in]
              n351 = call "myRIO_BRig_RT_dataLC_Wrong_OnOff_l1.vi"() -> ("output_Wrong_OnOff_l1"=w517:i32)  [unwired: 11 in]
              n352 = call "myRIO_BRig_RT_dataLC_Wrong_Tdelay_l1.vi"() -> ("output_Wrong_Tdelay_l1"=w516:i32)  [unwired: 11 in]
              n353 = call "myRIO_BRig_RT_dataLC_Wrong_Block_l1.vi"() -> ("output_Wrong_Block_l1"=w515:i32)  [unwired: 11 in]
              n354 = call "myRIO_BRig_RT_dataLC_Wrong_Trial_l1.vi"() -> ("output_Wrong_Trial_l1"=w514:i32)  [unwired: 11 in]
              n355 = call "myRIO_BRig_RT_dataLC_Wrong_Probability_l1.vi"() -> ("output_Wrong_Probability_l1"=w513:i32)  [unwired: 11 in]
              n356 = call "myRIO_BRig_RT_dataLC_Selection_OnOff_Switch_l1.vi"() -> ("output_Selection_OnOff_Switch_l1"=w508:i32)  [unwired: 11 in]
              n357 = call "myRIO_BRig_RT_dataLC_Selection_Tdelay_Switch_l1.vi"() -> ("output_Selection_Tdelay_Switch_l1"=w507:i32)  [unwired: 11 in]
              n358 = call "myRIO_BRig_RT_dataLC_Selection_Block_Switch_l1.vi"() -> ("output_Selection_Block_Switch_l1"=w506:i32)  [unwired: 11 in]
              n359 = call "myRIO_BRig_RT_dataLC_Selection_Count_Switch_l1.vi"() -> ("output_Selection_Count_Switch_l1"=w505:i32)  [unwired: 11 in]
              n360 = call "myRIO_BRig_RT_dataLC_Selection_Probability_Switch_l1.vi"() -> ("output_Selection_Probability_Switch_l1"=w504:i32)  [unwired: 11 in]
              n361 = call "myRIO_BRig_RT_dataLC_Selection_OnOff_NS_l1.vi"() -> ("output_Selection_OnOff_NS_l1"=w503:i32)  [unwired: 11 in]
              n362 = call "myRIO_BRig_RT_dataLC_Selection_Tdelay_NS_l1.vi"() -> ("output_Selection_Tdelay_NS_l1"=w502:i32)  [unwired: 11 in]
              n363 = call "myRIO_BRig_RT_dataLC_Selection_Block_NS_l1.vi"() -> ("output_Selection_Block_NS_l1"=w501:i32)  [unwired: 11 in]
              n364 = call "myRIO_BRig_RT_dataLC_Selection_Count_NS_l1.vi"() -> ("output_Selection_Count_NS_l1"=w500:i32)  [unwired: 11 in]
              n365 = call "myRIO_BRig_RT_dataLC_Selection_Probability_NS_l1.vi"() -> ("output_Selection_Probability_NS_l1"=w499:i32)  [unwired: 11 in]
              n366 = Index Array(array=w529, index #1=w528, index #2=w527, index #3=w526, index #4=w525, index #5=w524, index #6=w517, index #7=w516, index #8=w515, index #9=w514, index #10=w513, index #11=w508, index #12=w507, index #13=w506, index #14=w505, index #15=w504, index #16=w503, index #17=w502, index #18=w501, index #19=w500, index #20=w499) -> (element #1=w523:u16, element #2=w522:u16, element #3=w521:u16, element #4=w520:u16, element #5=w519:u16, element #6=w518:u16, element #7=w512:u16, element #8=w511:u16, element #9=w510:u16, element #10=w509:u16, element #11=w496:u16, element #12=w495:u16, element #13=w494:u16, element #14=w493:u16, element #15=w492:u16, element #16=w491:u16, element #17=w490:u16, element #18=w489:u16, element #19=w488:u16, element #20=w487:u16)
              n367 = Not Equal To 0?(x=w523) -> (x != 0?=w531:bool)
              n368 = Not Equal To 0?(x=w518) -> (x != 0?=w530:bool)
              n369 = Not Equal To 0?(x=w496) -> (x != 0?=w498:bool)
              n370 = Not Equal To 0?(x=w491) -> (x != 0?=w497:bool)
              n371 = local write "LC_Reward_OnOff_l1"(w531) -> ()
              n372 = local write "LC_Reward_Tdelay_l1"(w522) -> ()
              n373 = local write "LC_Reward_Block_l1"(w521) -> ()
              n374 = local write "LC_Reward_Trial_l1"(w520) -> ()
              n375 = local write "LC_Reward_Probability_l1"(w519) -> ()
              n376 = local write "LC_Wrong_OnOff_l1"(w530) -> ()
              n377 = local write "LC_Wrong_Tdelay_l1"(w512) -> ()
              n378 = local write "LC_Wrong_Block_l1"(w511) -> ()
              n379 = local write "LC_Wrong_Trial_l1"(w510) -> ()
              n380 = local write "LC_Wrong_Probability_l1"(w509) -> ()
              n381 = local write "LC_Sel_OnOff_Switch_l1"(w498) -> ()
              n382 = local write "LC_Sel_Tdelay_Switch_l1"(w495) -> ()
              n383 = local write "LC_Sel_Block_Switch_l1"(w494) -> ()
              n384 = local write "LC_Sel_Count_Switch_l1"(w493) -> ()
              n385 = local write "LC_Sel_Probability_Switch_l1"(w492) -> ()
              n386 = local write "LC_Sel_OnOff_NS_l1"(w497) -> ()
              n387 = local write "LC_Sel_Tdelay_NS_l1"(w490) -> ()
              n388 = local write "LC_Sel_Block_NS_l1"(w489) -> ()
              n389 = local write "LC_Sel_Count_NS_l1"(w488) -> ()
              n390 = local write "LC_Sel_Probability_NS_l1"(w487) -> ()
            }
            frame "UploadSettings_dataLC_4" {
              # "Count"
              # "Tdelay"
              # "Prob"
              # "OnOff"
              # "Block"
              # "Selection NonSwitch"
              # "Count"
              # "Tdelay"
              # "Prob"
              # "OnOff"
              # "Block"
              # "Selection Switch"
              # "Trial"
              # "Tdelay"
              # "Prob"
              # "OnOff"
              # "Block"
              # "Wrong"
              # "Reward"
              # "Trial"
              # "Tdelay"
              # "Prob"
              # "OnOff"
              # "Block"
              n391 = call "myRIO_BRig_RT_dataLC_Reward_OnOff_l2.vi"() -> ("output_Reward_OnOff_l2"=w539:i32)  [unwired: 11 in]
              n392 = call "myRIO_BRig_RT_dataLC_Reward_Tdelay_l2.vi"() -> ("output_Reward_Tdelay_l2"=w540:i32)  [unwired: 11 in]
              n393 = call "myRIO_BRig_RT_dataLC_Reward_Block_l2.vi"() -> ("output_Reward_Block_l2"=w541:i32)  [unwired: 11 in]
              n394 = call "myRIO_BRig_RT_dataLC_Reward_Trial_l2.vi"() -> ("output_Reward_Trial_l2"=w542:i32)  [unwired: 11 in]
              n395 = call "myRIO_BRig_RT_dataLC_Reward_Probability_l2.vi"() -> ("output_Reward_Probability_l2"=w543:i32)  [unwired: 11 in]
              n396 = call "myRIO_BRig_RT_dataLC_Wrong_OnOff_l2.vi"() -> ("output_Wrong_OnOff_l2"=w534:i32)  [unwired: 11 in]
              n397 = call "myRIO_BRig_RT_dataLC_Wrong_Tdelay_l2.vi"() -> ("output_Wrong_Tdelay_l2"=w535:i32)  [unwired: 11 in]
              n398 = call "myRIO_BRig_RT_dataLC_Wrong_Block_l2.vi"() -> ("output_Wrong_Block_l2"=w536:i32)  [unwired: 11 in]
              n399 = call "myRIO_BRig_RT_dataLC_Wrong_Trial_l2.vi"() -> ("output_Wrong_Trial_l2"=w537:i32)  [unwired: 11 in]
              n400 = call "myRIO_BRig_RT_dataLC_Wrong_Probability_l2.vi"() -> ("output_Wrong_Probability_l2"=w538:i32)  [unwired: 11 in]
              n401 = call "myRIO_BRig_RT_dataLC_Selection_OnOff_Switch_l2.vi"() -> ("output_Selection_OnOff_Switch_l2"=w549:i32)  [unwired: 11 in]
              n402 = call "myRIO_BRig_RT_dataLC_Selection_Tdelay_Switch_l2.vi"() -> ("output_Selection_Tdelay_Switch_l2"=w550:i32)  [unwired: 11 in]
              n403 = call "myRIO_BRig_RT_dataLC_Selection_Block_Switch_l2.vi"() -> ("output_Selection_Block_Switch_l2"=w551:i32)  [unwired: 11 in]
              n404 = call "myRIO_BRig_RT_dataLC_Selection_Count_Switch_l2.vi"() -> ("output_Selection_Count_Switch_l2"=w552:i32)  [unwired: 11 in]
              n405 = call "myRIO_BRig_RT_dataLC_Selection_Probability_Switch_l2.vi"() -> ("output_Selection_Probability_Switch_l1"=w553:i32)  [unwired: 11 in]
              n406 = call "myRIO_BRig_RT_dataLC_Selection_OnOff_NS_l2.vi"() -> ("output_Selection_OnOff_NS_l2"=w544:i32)  [unwired: 11 in]
              n407 = call "myRIO_BRig_RT_dataLC_Selection_Tdelay_NS_l2.vi"() -> ("output_Selection_Tdelay_NS_l2"=w545:i32)  [unwired: 11 in]
              n408 = call "myRIO_BRig_RT_dataLC_Selection_Block_NS_l2.vi"() -> ("output_Selection_Block_NS_l2"=w546:i32)  [unwired: 11 in]
              n409 = call "myRIO_BRig_RT_dataLC_Selection_Count_NS_l2.vi"() -> ("output_Selection_Count_NS_l2"=w547:i32)  [unwired: 11 in]
              n410 = call "myRIO_BRig_RT_dataLC_Selection_Probability_NS_l2.vi"() -> ("output_Selection_Probability_NS_l2"=w548:i32)  [unwired: 11 in]
              n411 = Index Array(array=w576, index #1=w539, index #2=w540, index #3=w541, index #4=w542, index #5=w543, index #6=w534, index #7=w535, index #8=w536, index #9=w537, index #10=w538, index #11=w549, index #12=w550, index #13=w551, index #14=w552, index #15=w553, index #16=w544, index #17=w545, index #18=w546, index #19=w547, index #20=w548) -> (element #1=w575:u16, element #2=w574:u16, element #3=w573:u16, element #4=w572:u16, element #5=w571:u16, element #6=w570:u16, element #7=w569:u16, element #8=w568:u16, element #9=w567:u16, element #10=w566:u16, element #11=w563:u16, element #12=w562:u16, element #13=w561:u16, element #14=w560:u16, element #15=w559:u16, element #16=w558:u16, element #17=w557:u16, element #18=w556:u16, element #19=w555:u16, element #20=w554:u16)
              n412 = Not Equal To 0?(x=w575) -> (x != 0?=w578:bool)
              n413 = Not Equal To 0?(x=w570) -> (x != 0?=w577:bool)
              n414 = Not Equal To 0?(x=w563) -> (x != 0?=w565:bool)
              n415 = Not Equal To 0?(x=w558) -> (x != 0?=w564:bool)
              n416 = local write "LC_Reward_OnOff_l2"(w578) -> ()
              n417 = local write "LC_Reward_Tdelay_l2"(w574) -> ()
              n418 = local write "LC_Reward_Block_l2"(w573) -> ()
              n419 = local write "LC_Reward_Trial_l2"(w572) -> ()
              n420 = local write "LC_Reward_Probability_l2"(w571) -> ()
              n421 = local write "LC_Wrong_OnOff_l2"(w577) -> ()
              n422 = local write "LC_Wrong_Tdelay_l2"(w569) -> ()
              n423 = local write "LC_Wrong_Block_l2"(w568) -> ()
              n424 = local write "LC_Wrong_Trial_l2"(w567) -> ()
              n425 = local write "LC_Wrong_Probability_l2"(w566) -> ()
              n426 = local write "LC_Sel_OnOff_Switch_l2"(w565) -> ()
              n427 = local write "LC_Sel_Tdelay_Switch_l2"(w562) -> ()
              n428 = local write "LC_Sel_Block_Switch_l2"(w561) -> ()
              n429 = local write "LC_Sel_Count_Switch_l2"(w560) -> ()
              n430 = local write "LC_Sel_Probability_Switch_l2"(w559) -> ()
              n431 = local write "LC_Sel_OnOff_NS_l2"(w564) -> ()
              n432 = local write "LC_Sel_Tdelay_NS_l2"(w557) -> ()
              n433 = local write "LC_Sel_Block_NS_l2"(w556) -> ()
              n434 = local write "LC_Sel_Count_NS_l2"(w555) -> ()
              n435 = local write "LC_Sel_Probability_NS_l2"(w554) -> ()
            }
            frame "UploadSettings_dataMTrig_1" {
              # "Tdelay_R"
              # "Tdelay_L"
              # "Tcycle_R"
              # "Tcycle_L"
              # "RewCalib_nCycle_R"
              # "RewCalib_nCycle_L"
              # "Solenoid"
              # "Laser_Tcycle"
              n436 = call "myRIO_BRig_RT_dataMTrig_Laser_Tcycle.vi"() -> ("output_Laser_Tcycle"=w588:i32)  [unwired: 11 in]
              n437 = call "myRIO_BRig_RT_dataMTrig_Solenoid_RewCalib_nCycle__L.vi"() -> ("output_Solenoid_RewCalib_nCycle__L"=w587:i32)  [unwired: 11 in]
              n438 = call "myRIO_BRig_RT_dataMTrig_Solenoid_RewCalib_nCycle__R.vi"() -> ("output_Solenoid_RewCalib_nCycle__R"=w586:i32)  [unwired: 11 in]
              n439 = call "myRIO_BRig_RT_dataMTrig_Solenoid_Tdelay__L.vi"() -> ("output_Solenoid_Tdelay__L"=w583:i32)  [unwired: 11 in]
              n440 = call "myRIO_BRig_RT_dataMTrig_Solenoid_Tdelay__R.vi"() -> ("output_Solenoid_Tdelay__R"=w582:i32)  [unwired: 11 in]
              n441 = call "myRIO_BRig_RT_dataMTrig_Solenoid_Tcycle__L.vi"() -> ("output_Solenoid_Tcycle__L"=w585:i32)  [unwired: 11 in]
              n442 = call "myRIO_BRig_RT_dataMTrig_Solenoid_Tcycle__R.vi"() -> ("output_Solenoid_Tcycle__R"=w584:i32)  [unwired: 11 in]
              n443 = Index Array(array=w581, index #1=w588, index #2=w587, index #3=w586, index #4=w585, index #5=w584, index #6=w583, index #7=w582) -> (element #1=w595:u16, element #2=w594:u16, element #3=w593:u16, element #4=w592:u16, element #5=w591:u16, element #6=w590:u16, element #7=w589:u16)
              n444 = Replace Array Subset(array=w597, new element #1=w595, index #1=w588, new element #2=w594, index #2=w587, new element #3=w593, index #3=w586, new element #4=w592, index #4=w585, new element #5=w591, index #5=w584, new element #6=w590, index #6=w583, new element #7=w589, index #7=w582) -> (w596:u16[])
              n445 = local write "MTrig_Solenoid_Tcycle__L"(w592) -> ()
              n446 = local write "MTrig_Solenoid_Tcycle__R"(w591) -> ()
              n447 = local write "MTrig_Laser_Tcycle"(w595) -> ()
            }
            frame "Idle" {
              # "There are a number of tasks we need to perform\nwhile idling. To preserve our timing loop, we\nbreak up the IDLE state into smaller states"
              # "Laser_Tcycle"
              # "Audio_Tcycle_R"
              # "Audio_Tcycle_L"
              n448 = local read "Laser_power_min_l1"() -> (w608:dbl)
              n449 = local read "Laser_power_min_l2"() -> (w607:dbl)
              n450 = local read "Audio_Amp__R"() -> (w610:u16)
              n451 = local read "Audio_Amp__L"() -> (w612:u16)
              n452 = local read "Audio_Freq__R"() -> (w609:u8)
              n453 = local read "Audio_Freq__L"() -> (w611:u8)
              n454 = local read "CueLed_baseline"() -> (w603:bool)
              n455 = local read "Laser2_baseline"() -> (w602:bool)
              n456 = local read "Laser1_baseline"() -> (w601:bool)
              n457 = Select(t=myRIO_BRig_RT__Case_NonExp_stateList."SendData" ("Enum"), s="SendData", f=myRIO_BRig_RT__Case_NonExp_stateList."Idle_2" ("Enum")) -> (s? t:f=w617:T1)
              n458 = call "myRIO__convert__Voltage_to_FPGAvalue.vi"("input_voltage"=w608) -> ("output_PortA"=w599:u16)  [unwired: 9 in, 1 out]
              n459 = call "myRIO__convert__Voltage_to_FPGAvalue.vi"("input_voltage"=w607) -> ("output_PortA"=w600:u16)  [unwired: 9 in, 1 out]
              n460 = Select(t=myRIO_BRig_RT__Case_NonExp_stateList."TestConnection" ("Enum"), s="TestConnection", f=w617) -> (s? t:f=w621:T1)
              n461 = xnode "Read/Write Control"("FPGA VI Reference In"=w614, "error in"=w613, "audioAmp_L"=w612, "audioFreq_L_kHz"=w611, "audioAmp_R"=w610, "audioFreq_R_kHz"=w609, "AnaOut_0"=w599, "AnaOut_1"=w600, "CueLed_Baseline"=w603, "L2Led_Baseline"=w602, "L1Led_Baseline"=w601) -> ("error out"=w606:errorcluster)  [unwired: 1 out]
              n462 = call "myRIO_BRig_RT_dataMTrig_Audio_Tcycle__L.vi"() -> ("output_Audio_Tcycle__L"=w628:i32)  [unwired: 11 in]
              n463 = call "myRIO_BRig_RT_dataMTrig_Audio_Tcycle__R.vi"() -> ("output_Audio_Tcycle__R"=w627:i32)  [unwired: 11 in]
              n464 = call "myRIO_BRig_RT_dataMTrig_Laser_Tcycle.vi"() -> ("output_Laser_Tcycle"=w626:i32)  [unwired: 11 in]
              n465 = call "myRIO_BRig_RT_dataMTrig_CueLed_Tcycle.vi"() -> ("output_CueLed_Tcycle"=w605:i32)  [unwired: 11 in]
              n466 = local write "error out"(w606) -> ()
              n467 = local read "Tcycle_Cue_Audio_min"() -> (w616:u16)
              n468 = local read "MTrig_Laser_Tcycle"() -> (w615:u16)
              n469 = local read "Tcycle_Cue_LED_min"() -> (w604:u16)
              n470 = Replace Array Subset(array=w624, new element #1=w616, index #1=w628, new element #2=w616, index #2=w627, new element #3=w615, index #3=w626, new element #4=w604, index #4=w605) -> (w625:u16[])
            }
            frame "Idle_2" {
              w651 = u16 0 ("t")
              # "There are a number of tasks we need to perform\nwhile idling. To preserve our timing loop, we\nbreak up the IDLE state into smaller states"
              # "Ncycles"
              # "Ncycles"
              # "RewCalib"
              # "RewCalib"
              # "Solenoid R"
              # "Solenoid L"
              n471 = local read "MTrig_Laser_Switch"() -> (w644:bool)
              n472 = local read "count_warmup_R"() -> (w650:u16)
              n473 = local read "count_warmup_L"() -> (w655:u16)
              n474 = call "myRIO_BRig_RT_dataMTrig_Solenoid_RewCalib_OnOff__R.vi"() -> ("output_Solenoid_RewCalib_OnOff__R"=w666:i32)  [unwired: 11 in]
              n475 = call "myRIO_BRig_RT_dataMTrig_Solenoid_N__R.vi"() -> ("output_Solenoid_N__R"=w665:i32)  [unwired: 11 in]
              n476 = call "myRIO_BRig_RT_dataMTrig_Solenoid_RewCalib_OnOff__L.vi"() -> ("output_Solenoid_RewCalib_OnOff__L"=w681:i32)  [unwired: 11 in]
              n477 = call "myRIO_BRig_RT_dataMTrig_Solenoid_N__L.vi"() -> ("output_Solenoid_N__L"=w669:i32)  [unwired: 11 in]
              n478 = case shown="False" w644 {
                tunnel: "LR_reward_Event" -> [w687 w691]
                tunnel: "LR_wrong_Event" -> [w686 w690]
                tunnel: "LR_reward_Laser" -> [w685 w689]
                tunnel: "LR_wrong_Laser" -> [w684 w688]
                tunnel: [w687 _] -> w639
                tunnel: [w686 _] -> w638
                tunnel: [w685 _] -> w637
                tunnel: [w684 _] -> w636
                tunnel: [_ w691] -> w635
                tunnel: [_ w690] -> w634
                tunnel: [_ w689] -> w633
                tunnel: [_ w688] -> w632
                frame False {
                }
                frame True {
                }
              }
              n479 = Index Array(array=w672, index #1=w681, index #2=w669, index #3=w666, index #4=w665) -> (element #1=w668:u16, element #2=w663:u16, element #3=w664:u16, element #4=w662:u16)
              n480 = Select(t=w651, s="count_warmup_L_reset", f=w655) -> (s? t:f=→"count_warmup_L":u16)
              n481 = Select(t=w651, s="count_warmup_R_reset", f=w650) -> (s? t:f=→"count_warmup_R":u16)
              n482 = local read "RewCalib_Trig_L"() -> (w661:bool)
              n483 = local read "RewCalib_Trig_R"() -> (w660:bool)
              n484 = Equal To 0?(x=w663) -> (x = 0?=w671:bool)
              n485 = Equal To 0?(x=w662) -> (x = 0?=w670:bool)
              n486 = Not Equal To 0?(x=w664) -> (x != 0?=w682:bool)
              n487 = Not Equal To 0?(x=w668) -> (x != 0?=w683:bool)
              n488 = And(x=w671, y=w670) -> (x .and. y?=w675:bool)
              n489 = Or(x=w661, y=w660) -> (x .or. y?=w676:bool)
              n490 = Not Exclusive Or(1:w683, 2:w661) -> (0:w678:bool)
              n491 = xnode "Read/Write Control"("FPGA VI Reference In"=w630, "error in"=w631, "Left(F)_or_Right(T)"="Left(F)_or_Right(T)", "SelectionState"="SelectionState", "ignoreWrong"="ignoreWrong", "LR_reward_Event_l1"=w639, "LR_wrong_Event_l1"=w638, "LR_reward_Laser_l1"=w637, "LR_wrong_Laser_l1"=w636, "LR_reward_Event_l2"=w635, "LR_wrong_Event_l2"=w634, "LR_reward_Laser_l2"=w633, "LR_wrong_laser_l2"=w632) -> ("error out"=w629:errorcluster, "SelectReward"=→"SelectReward":bool, "SelectWrong"=→"SelectWrong":bool)  [unwired: 1 out]
              n492 = Not Exclusive Or(1:w682, 2:w660) -> (0:w680:bool)
              n493 = And(x=w676, y=w675) -> (x .and. y?=w658:bool)
              n494 = Not(x=w678) -> (.not. x?=w677:bool)
              n495 = Not(x=w680) -> (.not. x?=w679:bool)
              n496 = Or(x=w677, y=w679) -> (x .or. y?=w659:bool)
              n497 = Or(x=w658, y=w659) -> (x .or. y?=w674:bool)
              n498 = local write "error out"(w629) -> ()
              n499 = Select(t=myRIO_BRig_RT__Case_NonExp_stateList."RewardCalibration_pre" ("Enum"), s=w674, f=myRIO_BRig_RT__Case_NonExp_stateList."Idle_3" ("Enum")) -> (s? t:f=w657:T1)
            }
            frame "Idle_3" {
              # "There are a number of tasks we need to perform\nwhile idling. To preserve our timing loop, we\nbreak up the IDLE state into smaller states"
              n500 = local read "Laser_Tshutter_l1"() -> (w710:dbl)
              n501 = local read "Laser_duration_l1"() -> (w709:u16)
              n502 = local read "Laser_Tshutter_l2"() -> (w706:dbl)
              n503 = local read "Laser_duration_l2"() -> (w705:u16)
              n504 = local read "Laser_Tpeak_l1"() -> (w712:dbl)
              n505 = local read "Laser_Tpeak_l2"() -> (w708:dbl)
              n506 = local read "CueLed_Tpeak"() -> (w703:dbl)
              n507 = local read "Laser_Freq_l1"() -> (w711:dbl)
              n508 = local read "Laser_Freq_l2"() -> (w707:dbl)
              n509 = local read "CueLed_Freq"() -> (w702:dbl)
              n510 = local read "FPGA_count2ms"() -> (w704:dbl)
              n511 = To Unsigned Word Integer(number=w704) -> (unsigned 16bit integer=w713:u16)
              n512 = call "myRIO_BRig_RT__calc_laser_FPGA_N.vi"("input_FPGA_ms2count"=w704, "input_Tpeak"=w712, "input_Freq"=w711, "input_Tshutter"=w710, "input_duration"=w709) -> ("output_laser_Npeak"=w701:u32, "output_laser_Nvalley"=w699:u32, "output_laser_Nshutter"=w697:u32, "output_laser_Nduration"=w695:u32)  [unwired: 6 in, 1 out]
              n513 = call "myRIO_BRig_RT__calc_laser_FPGA_N.vi"("input_FPGA_ms2count"=w704, "input_Tpeak"=w708, "input_Freq"=w707, "input_Tshutter"=w706, "input_duration"=w705) -> ("output_laser_Npeak"=w700:u32, "output_laser_Nvalley"=w698:u32, "output_laser_Nshutter"=w696:u32, "output_laser_Nduration"=w694:u32)  [unwired: 6 in, 1 out]
              n514 = call "myRIO_BRig_RT__calc_laser_FPGA_N__CueLed.vi"("input_FPGA_ms2count"=w704, "input_Tpeak"=w703, "input_Freq"=w702) -> ("output_laser_Npeak"=w693:u32, "output_laser_Nvalley"=w692:u32)  [unwired: 11 in]
              n515 = xnode "Read/Write Control"("FPGA VI Reference In"=w718, "error in"=w717, "k1__counter_per_ms"=w713, "LC_nPeak_l1"=w701, "LC_nPeak_l2"=w700, "LC_nValley_l1"=w699, "LC_nValley_l2"=w698, "LC_nShutter_l1"=w697, "LC_nShutter_l2"=w696, "LR_reward_nTotal_l1"=w695, "LR_wrong_nTotal_l1"=w695, "LR_reward_nTotal_l2"=w694, "LR_wrong_nTotal_l2"=w694, "CueLed_nPeak"=w693, "CueLed_nValley"=w692) -> ("error out"=w714:errorcluster)  [unwired: 1 out]
              n516 = local write "error out"(w714) -> ()
            }
            frame "Idle_4" {
              w740 = u8 0 ("f")
              # "There are a number of tasks we need to perform\nwhile idling. To preserve our timing loop, we\nbreak up the IDLE state into smaller states"
              n517 = local read "MTrig_Solenoid_trig__L"() -> (w731:bool)
              n518 = local read "MTrig_Solenoid_trig__R"() -> (w741:bool)
              n519 = local read "warmupType"() -> (w724:u8)
              n520 = local read "warmup"() -> (w733:bool)
              n521 = Not Equal To 0?(x=w724) -> (x != 0?=w723:bool)
              n522 = Not(x=w723) -> (.not. x?=w734:bool)
              n523 = Select(t=u8 1, s=w731, f=w740) -> (s? t:f=w739:u8)
              n524 = Select(t=u8 2, s=w741, f=w740) -> (s? t:f=w738:u8)
              n525 = And(x=w733, y=w734) -> (x .and. y?=w732:bool)
              n526 = And(x=w733, y=w723) -> (x .and. y?=w727:bool)
              n527 = Add(x=w739, y=w738) -> (x+y=w737:u8)
              n528 = case shown="3" w737 {
                tunnel: w736 -> [w744 w748 w781 w812]
                tunnel: [w744 w747 w780 w811] -> w735
                tunnel: w732 -> [_ w746 w779 w810]
                tunnel: [_ TRUE TRUE TRUE] -> w729
                frame 0, Default {
                }
                frame 1 {
                  n529 = case shown="False" w746 {
                    tunnel: w748 -> [w761 w776]
                    tunnel: [w760 w775] -> w747
                    frame True {
                      # "Audio_L"
                      # "Solenoid_L"
                      n530 = call "myRIO_BRig_RT_dataMTrig_Solenoid_N__L.vi"() -> ("output_Solenoid_N__L"=w758:i32)  [unwired: 11 in]
                      n531 = call "myRIO_BRig_RT_dataMTrig_Audio_N__L.vi"() -> ("output_Audio_N__L"=w756:i32)  [unwired: 11 in]
                      n532 = call "myRIO_BRig_RT_dataMTrig_Audio_N__R.vi"() -> ("output_Audio_N__R"=w751:i32)  [unwired: 11 in]
                      n533 = local read "sp_LeftSpout"() -> (w755:u16)
                      n534 = Index Array(array=w761, index #1=w758, index #2=w756, index #3=w751) -> (element #1=w759:u16, element #2=w754:u16, element #3=w753:u16)
                      n535 = Increment(x=w759) -> (x+1=w757:u16)
                      n536 = case shown="2" w755 {
                        tunnel: w754 -> [w764 w767 w769]
                        tunnel: w753 -> [w762 w766 w771]
                        tunnel: [w763 w767 w768] -> w752
                        tunnel: [w762 w765 w770] -> w750
                        frame 0, Default {
                          n537 = Increment(x=w764) -> (x+1=w763:u16)
                        }
                        frame 1 {
                          n538 = Increment(x=w766) -> (x+1=w765:u16)
                        }
                        frame 2 {
                          n539 = Increment(x=w771) -> (x+1=w770:u16)
                          n540 = Increment(x=w769) -> (x+1=w768:u16)
                        }
                      }
                      n541 = Replace Array Subset(array=w761, new element #1=w757, index #1=w758, new element #2=w752, index #2=w756, new element #3=w750, index #3=w751) -> (w760:u16[])
                    }
                    frame False {
                      # "Solenoid_L"
                      n542 = call "myRIO_BRig_RT_dataMTrig_Solenoid_N__L.vi"() -> ("output_Solenoid_N__L"=w773:i32)  [unwired: 11 in]
                      n543 = Index Array(array=w776, index=w773) -> (element=w774:u16)
                      n544 = Increment(x=w774) -> (x+1=w772:u16)
                      n545 = Replace Array Subset(array=w776, new element=w772, index=w773) -> (w775:u16[])
                    }
                  }
                  n546 = local write "MTrig_Solenoid_trig__L"(FALSE) -> ()
                }
                frame 2 {
                  n547 = case shown="True" w779 {
                    tunnel: w781 -> [w793 w808]
                    tunnel: [w792 w807] -> w780
                    frame True {
                      # "Solenoid_R"
                      n548 = call "myRIO_BRig_RT_dataMTrig_Solenoid_N__R.vi"() -> ("output_Solenoid_N__R"=w782:i32)  [unwired: 11 in]
                      n549 = call "myRIO_BRig_RT_dataMTrig_Audio_N__L.vi"() -> ("output_Audio_N__L"=w789:i32)  [unwired: 11 in]
                      n550 = call "myRIO_BRig_RT_dataMTrig_Audio_N__R.vi"() -> ("output_Audio_N__R"=w784:i32)  [unwired: 11 in]
                      n551 = local read "sp_RightSpout"() -> (w788:u16)
                      n552 = Index Array(array=w793, index #1=w782, index #2=w789, index #3=w784) -> (element #1=w791:u16, element #2=w787:u16, element #3=w786:u16)
                      n553 = Increment(x=w791) -> (x+1=w790:u16)
                      n554 = case shown="2" w788 {
                        tunnel: w787 -> [w796 w799 w801]
                        tunnel: w786 -> [w794 w798 w803]
                        tunnel: [w795 w799 w800] -> w785
                        tunnel: [w794 w797 w802] -> w783
                        frame 0, Default {
                          n555 = Increment(x=w796) -> (x+1=w795:u16)
                        }
                        frame 1 {
                          n556 = Increment(x=w798) -> (x+1=w797:u16)
                        }
                        frame 2 {
                          n557 = Increment(x=w803) -> (x+1=w802:u16)
                          n558 = Increment(x=w801) -> (x+1=w800:u16)
                        }
                      }
                      n559 = Replace Array Subset(array=w793, new element #1=w790, index #1=w782, new element #2=w785, index #2=w789, new element #3=w783, index #3=w784) -> (w792:u16[])
                    }
                    frame False {
                      # "Solenoid_R"
                      n560 = call "myRIO_BRig_RT_dataMTrig_Solenoid_N__R.vi"() -> ("output_Solenoid_N__R"=w804:i32)  [unwired: 11 in]
                      n561 = Index Array(array=w808, index=w804) -> (element=w806:u16)
                      n562 = Increment(x=w806) -> (x+1=w805:u16)
                      n563 = Replace Array Subset(array=w808, new element=w805, index=w804) -> (w807:u16[])
                    }
                  }
                  n564 = local write "MTrig_Solenoid_trig__R"(FALSE) -> ()
                }
                frame 3 {
                  w813 = FALSE
                  n565 = case shown="True" w810 {
                    tunnel: w812 -> [w827 w835]
                    tunnel: [w826 w834] -> w811
                    frame True {
                      # "Audio_R"
                      # "Solenoid_R"
                      # "Audio_L"
                      # "Solenoid_L"
                      n566 = call "myRIO_BRig_RT_dataMTrig_Solenoid_N__L.vi"() -> ("output_Solenoid_N__L"=w821:i32)  [unwired: 11 in]
                      n567 = call "myRIO_BRig_RT_dataMTrig_Audio_N__L.vi"() -> ("output_Audio_N__L"=w819:i32)  [unwired: 11 in]
                      n568 = call "myRIO_BRig_RT_dataMTrig_Solenoid_N__R.vi"() -> ("output_Solenoid_N__R"=w817:i32)  [unwired: 11 in]
                      n569 = call "myRIO_BRig_RT_dataMTrig_Audio_N__R.vi"() -> ("output_Audio_N__R"=w816:i32)  [unwired: 11 in]
                      n570 = Index Array(array=w827, index #1=w821, index #2=w819, index #3=w817, index #4=w816) -> (element #1=w825:u16, element #2=w824:u16, element #3=w823:u16, element #4=w822:u16)
                      n571 = Increment(x=w822) -> (x+1=w814:u16)
                      n572 = Increment(x=w825) -> (x+1=w820:u16)
                      n573 = Increment(x=w824) -> (x+1=w818:u16)
                      n574 = Increment(x=w823) -> (x+1=w815:u16)
                      n575 = Replace Array Subset(array=w827, new element #1=w820, index #1=w821, new element #2=w818, index #2=w819, new element #3=w815, index #3=w817, new element #4=w814, index #4=w816) -> (w826:u16[])
                    }
                    frame False {
                      # "Solenoid_R"
                      # "Solenoid_L"
                      n576 = call "myRIO_BRig_RT_dataMTrig_Solenoid_N__L.vi"() -> ("output_Solenoid_N__L"=w831:i32)  [unwired: 11 in]
                      n577 = call "myRIO_BRig_RT_dataMTrig_Solenoid_N__R.vi"() -> ("output_Solenoid_N__R"=w828:i32)  [unwired: 11 in]
                      n578 = Index Array(array=w835, index #1=w831, index #2=w828) -> (element #1=w833:u16, element #2=w832:u16)
                      n579 = Increment(x=w833) -> (x+1=w830:u16)
                      n580 = Increment(x=w832) -> (x+1=w829:u16)
                      n581 = Replace Array Subset(array=w835, new element #1=w830, index #1=w831, new element #2=w829, index #2=w828) -> (w834:u16[])
                    }
                  }
                  n582 = local write "MTrig_Solenoid_trig__L"(w813) -> ()
                  n583 = local write "MTrig_Solenoid_trig__R"(w813) -> ()
                }
              }
              n584 = local read "get_countPerMS"() -> (w722:bool)
              n585 = Select(t=myRIO_BRig_RT__Case_NonExp_stateList."Get_FPGA_count_per_ms" ("Enum"), s=w722, f=myRIO_BRig_RT__Case_NonExp_stateList."Idle_6" ("Enum")) -> (s? t:f=w720:T1)
              n586 = Select(t=myRIO_BRig_RT__Case_NonExp_stateList."Cue_pre", s=w727, f=myRIO_BRig_RT__Case_NonExp_stateList."DispenseWater_pre" ("Enum")) -> (s? t:f=w725:T1)
              n587 = Select(t=w725, s=w729, f=w720) -> (s? t:f=w730:T1)
            }
            frame "Idle_5" {
              w858 = u8 0 ("f")
              # "There are a number of tasks we need to perform\nwhile idling. To preserve our timing loop, we\nbreak up the IDLE state into smaller states"
              n588 = local read "MTrig_Solenoid_trig__L"() -> (w850:bool)
              n589 = local read "MTrig_Solenoid_trig__R"() -> (w859:bool)
              n590 = local read "warmup"() -> (w837:bool)
              n591 = local read "warmupType"() -> (w839:u8)
              n592 = local read "Cue1Param_CueType_Switch"() -> (w838:u16)
              n593 = Not Equal To 0?(x=w839) -> (x != 0?=w836:bool)
              n594 = Not(x=w836) -> (.not. x?=w852:bool)
              n595 = And(x=w836, y=w837) -> (x .and. y?=w846:bool)
              n596 = Select(t=u8 1, s=w850, f=w858) -> (s? t:f=w857:u8)
              n597 = Select(t=u8 2, s=w859, f=w858) -> (s? t:f=w856:u8)
              n598 = And(x=w837, y=w852) -> (x .and. y?=w851:bool)
              n599 = Add(x=w857, y=w856) -> (x+y=w855:u8)
              n600 = case shown="3" w855 {
                tunnel: w854 -> [w862 w867 w904 w941]
                tunnel: [w862 w866 w905 w942] -> w853
                tunnel: w851 -> [_ w865 w903 w944]
                tunnel: [_ TRUE TRUE TRUE] -> w848
                tunnel: w838 -> [_ w863 w902 w943]
                frame 0, Default {
                }
                frame 1 {
                  n601 = case shown="True" w865 {
                    tunnel: w867 -> [w889 w901]
                    tunnel: [w890 w900] -> w866
                    tunnel: w863 -> [w869 _]
                    frame True {
                      n602 = case shown="2" w869 {
                        tunnel: [TRUE _ w894 w896] -> w878
                        tunnel: [_ TRUE w893 w896] -> w885
                        frame 0, Default {
                          # "Audio"
                        }
                        frame 1 {
                          # "LED"
                        }
                        frame 2 {
                          # "Audio or LED"
                          n603 = local read "Cue1Param_AudioLed_Probability_Switch"() -> (w895:u16)
                          n604 = call "myRIO__convert__Probability_to_TrueFalse.vi"("input_probability_u16"=w895) -> ("output_TF"=w893:bool)  [unwired: 10 in]
                          n605 = Not(x=w893) -> (.not. x?=w894:bool)
                        }
                        frame 3 {
                          w896 = TRUE
                          # "Audio and LED"
                        }
                      }
                      n606 = local read "sp_LeftSpout"() -> (w881:u16)
                      n607 = call "myRIO_BRig_RT_dataMTrig_Solenoid_N__L.vi"() -> ("output_Solenoid_N__L"=w888:i32)  [unwired: 11 in]
                      n608 = call "myRIO_BRig_RT_dataMTrig_CueLed_N.vi"() -> ("output_CueLed_N"=w886:i32)  [unwired: 11 in]
                      n609 = call "myRIO_BRig_RT_dataMTrig_Audio_N__L.vi"() -> ("output_Audio_N__L"=w873:i32)  [unwired: 11 in]
                      n610 = call "myRIO_BRig_RT_dataMTrig_Audio_N__R.vi"() -> ("output_Audio_N__R"=w871:i32)  [unwired: 11 in]
                      n611 = Boolean To (0,1)(Boolean=w885) -> (0, 1=w884:i16)
                      n612 = To Unsigned Word Integer(number=w884) -> (unsigned 16bit integer=w883:u16)
                      n613 = Not Equal?(x=u16 1, y=w881) -> (x != y?=w880:bool)
                      n614 = Not Equal To 0?(x=w881) -> (x != 0?=w879:bool)
                      n615 = And(x=w880, y=w878) -> (x .and. y?=w876:bool)
                      n616 = And(x=w879, y=w878) -> (x .and. y?=w874:bool)
                      n617 = Boolean To (0,1)(Boolean=w876) -> (0, 1=w877:i16)
                      n618 = Boolean To (0,1)(Boolean=w874) -> (0, 1=w875:i16)
                      n619 = To Unsigned Word Integer(number=w877) -> (unsigned 16bit integer=w872:u16)
                      n620 = To Unsigned Word Integer(number=w875) -> (unsigned 16bit integer=w870:u16)
                      n621 = Replace Array Subset(array=w889, new element #1=u16 1 ("new element/subarray"), index #1=w888, new element #2=w883, index #2=w886, new element #3=w872, index #3=w873, new element #4=w870, index #4=w871) -> (w890:u16[])
                    }
                    frame False {
                      n622 = call "myRIO_BRig_RT_dataMTrig_Solenoid_N__L.vi"() -> ("output_Solenoid_N__L"=w898:i32)  [unwired: 11 in]
                      n623 = Index Array(array=w901, index=w898) -> (element=w899:u16)
                      n624 = Increment(x=w899) -> (x+1=w897:u16)
                      n625 = Replace Array Subset(array=w901, new element=w897, index=w898) -> (w900:u16[])
                    }
                  }
                  n626 = local write "MTrig_Solenoid_trig__L"(FALSE) -> ()
                }
                frame 2 {
                  n627 = case shown="True" w903 {
                    tunnel: [w929 w940] -> w905
                    tunnel: w904 -> [w909 w936]
                    tunnel: w902 -> [w908 _]
                    frame True {
                      n628 = case shown="2" w908 {
                        tunnel: [TRUE _ w933 w935] -> w918
                        tunnel: [_ TRUE w932 w935] -> w925
                        frame 0, Default {
                          # "Audio"
                        }
                        frame 1 {
                          # "LED"
                        }
                        frame 2 {
                          # "Audio or LED"
                          n629 = local read "Cue1Param_AudioLed_Probability_Switch"() -> (w934:u16)
                          n630 = call "myRIO__convert__Probability_to_TrueFalse.vi"("input_probability_u16"=w934) -> ("output_TF"=w932:bool)  [unwired: 10 in]
                          n631 = Not(x=w932) -> (.not. x?=w933:bool)
                        }
                        frame 3 {
                          w935 = TRUE
                          # "Audio and LED"
                        }
                      }
                      n632 = local read "sp_RightSpout"() -> (w921:u16)
                      n633 = call "myRIO_BRig_RT_dataMTrig_Solenoid_N__R.vi"() -> ("output_Solenoid_N__R"=w928:i32)  [unwired: 11 in]
                      n634 = call "myRIO_BRig_RT_dataMTrig_CueLed_N.vi"() -> ("output_CueLed_N"=w926:i32)  [unwired: 11 in]
                      n635 = call "myRIO_BRig_RT_dataMTrig_Audio_N__L.vi"() -> ("output_Audio_N__L"=w913:i32)  [unwired: 11 in]
                      n636 = call "myRIO_BRig_RT_dataMTrig_Audio_N__R.vi"() -> ("output_Audio_N__R"=w911:i32)  [unwired: 11 in]
                      n637 = Boolean To (0,1)(Boolean=w925) -> (0, 1=w924:i16)
                      n638 = To Unsigned Word Integer(number=w924) -> (unsigned 16bit integer=w923:u16)
                      n639 = Not Equal?(x=u16 1, y=w921) -> (x != y?=w920:bool)
                      n640 = Not Equal To 0?(x=w921) -> (x != 0?=w919:bool)
                      n641 = And(x=w920, y=w918) -> (x .and. y?=w916:bool)
                      n642 = And(x=w919, y=w918) -> (x .and. y?=w914:bool)
                      n643 = Boolean To (0,1)(Boolean=w916) -> (0, 1=w917:i16)
                      n644 = Boolean To (0,1)(Boolean=w914) -> (0, 1=w915:i16)
                      n645 = To Unsigned Word Integer(number=w917) -> (unsigned 16bit integer=w912:u16)
                      n646 = To Unsigned Word Integer(number=w915) -> (unsigned 16bit integer=w910:u16)
                      n647 = Replace Array Subset(array=w909, new element #1=u16 1 ("new element/subarray"), index #1=w928, new element #2=w923, index #2=w926, new element #3=w912, index #3=w913, new element #4=w910, index #4=w911) -> (w929:u16[])
                    }
                    frame False {
                      n648 = call "myRIO_BRig_RT_dataMTrig_Solenoid_N__R.vi"() -> ("output_Solenoid_N__R"=w938:i32)  [unwired: 11 in]
                      n649 = Index Array(array=w936, index=w938) -> (element=w937:u16)
                      n650 = Increment(x=w937) -> (x+1=w939:u16)
                      n651 = Replace Array Subset(array=w936, new element=w939, index=w938) -> (w940:u16[])
                    }
                  }
                  n652 = local write "MTrig_Solenoid_trig__R"(FALSE) -> ()
                }
                frame 3 {
                  w945 = FALSE
                  n653 = case shown="True" w944 {
                    tunnel: [w961 w975] -> w942
                    tunnel: w943 -> [w952 _]
                    tunnel: w941 -> [w951 w971]
                    frame True {
                      w947 = u16 1 ("new element/subarray")
                      n654 = case shown="2" w952 {
                        tunnel: [TRUE _ w965 w967] -> w950
                        tunnel: [_ TRUE w964 w967] -> w958
                        frame 0, Default {
                          # "Audio"
                        }
                        frame 1 {
                          # "LED"
                        }
                        frame 2 {
                          # "Audio or LED"
                          n655 = local read "Cue1Param_AudioLed_Probability_Switch"() -> (w966:u16)
                          n656 = call "myRIO__convert__Probability_to_TrueFalse.vi"("input_probability_u16"=w966) -> ("output_TF"=w964:bool)  [unwired: 10 in]
                          n657 = Not(x=w964) -> (.not. x?=w965:bool)
                        }
                        frame 3 {
                          w967 = TRUE
                          # "Audio and LED"
                        }
                      }
                      n658 = call "myRIO_BRig_RT_dataMTrig_Solenoid_N__R.vi"() -> ("output_Solenoid_N__R"=w948:i32)  [unwired: 11 in]
                      n659 = call "myRIO_BRig_RT_dataMTrig_Solenoid_N__L.vi"() -> ("output_Solenoid_N__L"=w960:i32)  [unwired: 11 in]
                      n660 = call "myRIO_BRig_RT_dataMTrig_CueLed_N.vi"() -> ("output_CueLed_N"=w959:i32)  [unwired: 11 in]
                      n661 = call "myRIO_BRig_RT_dataMTrig_Audio_N__L.vi"() -> ("output_Audio_N__L"=w954:i32)  [unwired: 11 in]
                      n662 = call "myRIO_BRig_RT_dataMTrig_Audio_N__R.vi"() -> ("output_Audio_N__R"=w953:i32)  [unwired: 11 in]
                      n663 = Boolean To (0,1)(Boolean=w958) -> (0, 1=w957:i16)
                      n664 = To Unsigned Word Integer(number=w957) -> (unsigned 16bit integer=w956:u16)
                      n665 = Boolean To (0,1)(Boolean=w950) -> (0, 1=w955:i16)
                      n666 = To Unsigned Word Integer(number=w955) -> (unsigned 16bit integer=w949:u16)
                      n667 = Replace Array Subset(array=w951, new element #1=w947, index #1=w948, new element #2=w947, index #2=w960, new element #3=w956, index #3=w959, new element #4=w949, index #4=w954, new element #5=w949, index #5=w953) -> (w961:u16[])
                    }
                    frame False {
                      n668 = call "myRIO_BRig_RT_dataMTrig_Solenoid_N__L.vi"() -> ("output_Solenoid_N__L"=w974:i32)  [unwired: 11 in]
                      n669 = call "myRIO_BRig_RT_dataMTrig_Solenoid_N__R.vi"() -> ("output_Solenoid_N__R"=w970:i32)  [unwired: 11 in]
                      n670 = Index Array(array=w971, index #1=w974, index #2=w970) -> (element #1=w972:u16, element #2=w969:u16)
                      n671 = Increment(x=w972) -> (x+1=w973:u16)
                      n672 = Increment(x=w969) -> (x+1=w968:u16)
                      n673 = Replace Array Subset(array=w971, new element #1=w973, index #1=w974, new element #2=w968, index #2=w970) -> (w975:u16[])
                    }
                  }
                  n674 = local write "MTrig_Solenoid_trig__L"(w945) -> ()
                  n675 = local write "MTrig_Solenoid_trig__R"(w945) -> ()
                }
              }
              n676 = local read "get_countPerMS"() -> (w843:bool)
              n677 = Select(t=myRIO_BRig_RT__Case_NonExp_stateList."Cue_pre", s=w846, f=myRIO_BRig_RT__Case_NonExp_stateList."DispenseWater_pre" ("Enum")) -> (s? t:f=w844:T1)
              n678 = Select(t=myRIO_BRig_RT__Case_NonExp_stateList."Get_FPGA_count_per_ms" ("Enum"), s=w843, f=myRIO_BRig_RT__Case_NonExp_stateList."Idle_6" ("Enum")) -> (s? t:f=w841:T1)
              n679 = Select(t=w844, s=w848, f=w841) -> (s? t:f=w849:T1)
            }
            frame "Idle_6" {
              # "There are a number of tasks we need to perform\nwhile idling. To preserve our timing loop, we\nbreak up the IDLE state into smaller states"
              # "use dataMTrig as it is one of the last to transfer"
              n680 = call "myRIO_BRig_RT_comm_webdav_uploadReceived_check_v2,0.vi"("input_dataName"="dataMTrig") -> ("output_Iexist"=w980:bool)  [unwired: 9 in, 1 out]
              n681 = Select(t=myRIO_BRig_RT__Case_NonExp_stateList."UploadSettings_pre" ("Enum"), s=w980, f=myRIO_BRig_RT__Case_NonExp_stateList."Idle") -> (s? t:f=w978:T1)
            }
            frame "Cue_pre" {
              w988 = u16 0 ("new element/subarray")
              # "Audio cue or LED cue?"
              # "Audio, LED, or \"Audio or LED\""
              # "Right Audio?"
              # "Left Audio?"
              # "Left or Right?"
              # "Cue Audio?\n(T=Audio, F=LED)"
              # "Ncycle"
              # "count"
              # "Audio_R"
              # "Ncycle"
              # "count"
              # "Audio_L"
              n682 = local read "Cue1Param_CueType_Switch"() -> (w1009:u16)
              n683 = case shown="3" w1009 {
                tunnel: [TRUE _ w1029 w1031] -> w984
                tunnel: [_ TRUE w1028 w1031] -> w982
                frame 0, Default {
                  # "Audio"
                }
                frame 1 {
                  # "LED"
                }
                frame 2 {
                  # "Audio or LED"
                  n684 = local read "Cue1Param_AudioLed_Probability_Switch"() -> (w1030:u16)
                  n685 = call "myRIO__convert__Probability_to_TrueFalse.vi"("input_probability_u16"=w1030) -> ("output_TF"=w1028:bool)  [unwired: 10 in]
                  n686 = Not(x=w1028) -> (.not. x?=w1029:bool)
                }
                frame 3 {
                  w1031 = TRUE
                }
              }
              n687 = call "myRIO_BRig_RT_dataMTrig_Solenoid_N__L.vi"() -> ("output_Solenoid_N__L"=w1019:i32)  [unwired: 11 in]
              n688 = call "myRIO_BRig_RT_dataMTrig_Solenoid_N__R.vi"() -> ("output_Solenoid_N__R"=w1018:i32)  [unwired: 11 in]
              n689 = Index Array(array=w1015, index #1=w1019, index #2=w1018) -> (element #1=w1017:u16, element #2=w1016:u16)
              n690 = Not Equal To 0?(x=w1017) -> (x != 0?=w1008:bool)
              n691 = Not Equal To 0?(x=w1016) -> (x != 0?=w1007:bool)
              n692 = And(x=w984, y=w1008) -> (x .and. y?=w1002:bool)
              n693 = And(x=w984, y=w1007) -> (x .and. y?=w1000:bool)
              n694 = local read "sp_RightSpout"() -> (w1001:u16)
              n695 = local read "sp_LeftSpout"() -> (w1003:u16)
              n696 = Boolean To (0,1)(Boolean=w982) -> (0, 1=w986:i16)
              n697 = To Unsigned Word Integer(number=w986) -> (unsigned 16bit integer=w985:u16)
              n698 = case shown="0, Default" w1003 {
                tunnel: [w1023 _ w1025] -> w999
                tunnel: [_ w1024 w1025] -> w997
                tunnel: w1002 -> [w1023 w1024 w1025]
                frame 0, Default {
                }
                frame 1 {
                }
                frame 2 {
                }
              }
              n699 = case shown="0, Default" w1001 {
                tunnel: [w1020 _ w1022] -> w998
                tunnel: [_ w1021 w1022] -> w996
                tunnel: w1000 -> [w1020 w1021 w1022]
                frame 0, Default {
                }
                frame 1 {
                }
                frame 2 {
                }
              }
              n700 = call "myRIO_BRig_RT_dataMTrig_Audio_c__L.vi"() -> ("output_Audio_c__L"=w1013:i32)  [unwired: 11 in]
              n701 = call "myRIO_BRig_RT_dataMTrig_Audio_N__L.vi"() -> ("output_Audio_N__L"=w1012:i32)  [unwired: 11 in]
              n702 = call "myRIO_BRig_RT_dataMTrig_Audio_c__R.vi"() -> ("output_Audio_c__R"=w1011:i32)  [unwired: 11 in]
              n703 = call "myRIO_BRig_RT_dataMTrig_Audio_N__R.vi"() -> ("output_Audio_N__R"=w1010:i32)  [unwired: 11 in]
              n704 = call "myRIO_BRig_RT_dataMTrig_CueLed_c.vi"() -> ("output_CueLed_c"=w989:i32)  [unwired: 11 in]
              n705 = call "myRIO_BRig_RT_dataMTrig_CueLed_N.vi"() -> ("output_CueLed_N"=w987:i32)  [unwired: 11 in]
              n706 = Or(x=w999, y=w998) -> (x .or. y?=w995:bool)
              n707 = Boolean To (0,1)(Boolean=w995) -> (0, 1=w993:i16)
              n708 = To Unsigned Word Integer(number=w993) -> (unsigned 16bit integer=w992:u16)
              n709 = Or(x=w997, y=w996) -> (x .or. y?=w994:bool)
              n710 = Boolean To (0,1)(Boolean=w994) -> (0, 1=w991:i16)
              n711 = To Unsigned Word Integer(number=w991) -> (unsigned 16bit integer=w990:u16)
              n712 = Replace Array Subset(array=w1015, new element #1=w988, index #1=w1013, new element #2=w992, index #2=w1012, new element #3=w988, index #3=w1011, new element #4=w990, index #4=w1010, new element #5=w988, index #5=w989, new element #6=w985, index #6=w987) -> (w1014:u16[])
              n713 = Initialize Array(u16 0 ("element"), 1 ("dimension size")) -> (w1006:u16[])
            }
            frame "Cue" {
              # "warmupType\n0 = Cue with reward (not possible to be in this state with value==0)\n1 = Cue then reward\n2 = Cue then reward (no lick)"
              # "Audio cue"
              # "lick did not occur or warmupType==1"
              # "lick occurred?"
              # "Ncycle"
              # "Audio_R"
              # "Ncycle"
              # "Audio_L"
              n714 = local read "warmupType"() -> (w1041:u8)
              n715 = Greater?(x=w1047, y=w1046) -> (0:w1050:bool)
              n716 = Greater?(x=w1049, y=w1048) -> (0:w1045:bool)
              n717 = Or(x=w1045, y=w1050) -> (x .or. y?=w1039:bool)
              n718 = Equal?(x=w1041, y=u8 1) -> (x = y?=w1035:bool)
              n719 = Not(x=w1039) -> (.not. x?=w1038:bool)
              n720 = call "myRIO_BRig_RT_dataMTrig_Audio_N__L.vi"() -> ("output_Audio_N__L"=w1052:i32)  [unwired: 11 in]
              n721 = call "myRIO_BRig_RT_dataMTrig_Audio_N__R.vi"() -> ("output_Audio_N__R"=w1051:i32)  [unwired: 11 in]
              n722 = call "myRIO_BRig_RT_dataMTrig_CueLed_N.vi"() -> ("output_CueLed_N"=w1032:i32)  [unwired: 11 in]
              n723 = Or(x=w1038, y=w1035) -> (x .or. y?=w1036:bool)
              n724 = case shown="True" w1036 {
                tunnel: w1052 -> [w1058 w1079]
                tunnel: w1051 -> [w1057 w1078]
                tunnel: w1044 -> [w1060 w1073]
                tunnel: [w1059 w1073] -> w1043
                tunnel: w1042 -> [_ w1071]
                tunnel: [myRIO_BRig_RT__Case_NonExp_stateList."Idle" ("t") w1070] -> w1037
                tunnel: w1035 -> [_ w1069]
                tunnel: w1034 -> [_ w1065]
                tunnel: w1033 -> [_ w1064]
                tunnel: w1032 -> [_ w1063]
                frame False {
                  w1053 = u16 0 ("new element/subarray")
                  # "lick occurred and warmupType==2"
                  n725 = call "myRIO_BRig_RT_dataMTrig_Solenoid_N__R.vi"() -> ("output_Solenoid_N__R"=w1054:i32)  [unwired: 11 in]
                  n726 = call "myRIO_BRig_RT_dataMTrig_Solenoid_N__L.vi"() -> ("output_Solenoid_N__L"=w1055:i32)  [unwired: 11 in]
                  n727 = Replace Array Subset(array=w1060, new element #1=w1053, index #1=w1058, new element #2=w1053, index #2=w1057, new element #3=w1053, index #3=w1055, new element #4=w1053, index #4=w1054) -> (w1059:u16[])
                }
                frame True {
                  n728 = Not(x=w1069) -> (.not. x?=w1068:bool)
                  n729 = Index Array(array=w1073, index #1=w1079, index #2=w1078, index #3=w1063) -> (element #1=w1077:u16, element #2=w1076:u16, element #3=w1062:u16)
                  n730 = Equal To 0?(x=w1077) -> (x = 0?=w1075:bool)
                  n731 = Equal To 0?(x=w1076) -> (x = 0?=w1074:bool)
                  n732 = Equal To 0?(x=w1062) -> (x = 0?=w1061:bool)
                  n733 = Compound Arithmetic op=AND(w1075, w1074, w1061) -> (w1067:bool)
                  n734 = And(x=w1067, y=w1068) -> (x .and. y?=w1066:bool)
                  n735 = case shown="True" w1066 {
                    tunnel: w1065 -> [_ w1087]
                    tunnel: w1064 -> [_ w1082]
                    frame False {
                    }
                    frame True {
                      n736 = local read "count_warmup_R"() -> (w1080:u16)
                      n737 = local read "count_warmup_L"() -> (w1085:u16)
                      n738 = Increment(x=w1080) -> (x+1=w1083:u16)
                      n739 = Increment(x=w1085) -> (x+1=w1086:u16)
                      n740 = Select(t=w1083, s=w1082, f=w1080) -> (s? t:f=w1081:u16)
                      n741 = Select(t=w1086, s=w1087, f=w1085) -> (s? t:f=w1084:u16)
                      n742 = local write "count_warmup_R"(w1081) -> ()
                      n743 = local write "count_warmup_L"(w1084) -> ()
                    }
                  }
                  n744 = Select(t=myRIO_BRig_RT__Case_NonExp_stateList."DispenseWater_pre", s=w1067, f=w1071) -> (s? t:f=w1070:T1)
                }
              }
            }
            frame "RewardCalibration_pre" {
              (unwired) FALSE
              w1088 = FALSE
              w1099 = u8 0
              w1115 = u8 0
              # "Are we starting a RewardCalibration?\nOr are we stopping a RewardCalibration?\nOr is a RewardCalibration over?"
              # "RewCalib\nOnOff"
              # "N"
              # "Solenoid R"
              # "RewCalib\nOnOff"
              # "N"
              # "Solenoid L"
              n745 = local read "RewCalib_Trig_L"() -> (w1122:bool)
              n746 = local read "RewCalib_Trig_R"() -> (w1091:bool)
              n747 = call "myRIO_BRig_RT_dataMTrig_Solenoid_N__R.vi"() -> ("output_Solenoid_N__R"=w1093:i32)  [unwired: 11 in]
              n748 = call "myRIO_BRig_RT_dataMTrig_Solenoid_RewCalib_OnOff__R.vi"() -> ("output_Solenoid_RewCalib_OnOff__R"=w1090:i32)  [unwired: 11 in]
              n749 = call "myRIO_BRig_RT_dataMTrig_Solenoid_N__L.vi"() -> ("output_Solenoid_N__L"=w1108:i32)  [unwired: 11 in]
              n750 = call "myRIO_BRig_RT_dataMTrig_Solenoid_RewCalib_OnOff__L.vi"() -> ("output_Solenoid_RewCalib_OnOff__L"=w1109:i32)  [unwired: 11 in]
              n751 = Index Array(array=w1092, index #1=w1093, index #2=w1090) -> (element #1=w1103:u16, element #2=w1098:u16)
              n752 = Index Array(array=w1092, index #1=w1108, index #2=w1109) -> (element #1=w1119:u16, element #2=w1114:u16)
              n753 = Equal To 0?(x=w1103) -> (x = 0?=w1104:bool)
              n754 = Not Equal To 0?(x=w1098) -> (x != 0?=w1101:bool)
              n755 = Equal To 0?(x=w1119) -> (x = 0?=w1120:bool)
              n756 = Not Equal To 0?(x=w1114) -> (x != 0?=w1117:bool)
              n757 = local write "MTrig_Solenoid_trig__L"(w1088) -> ()
              n758 = local write "MTrig_Solenoid_trig__R"(w1088) -> ()
              n759 = Select(t=u8 1, s=w1091, f=w1099) -> (s? t:f=w1095:u8)
              n760 = Select(t=u8 1, s=w1122, f=w1115) -> (s? t:f=w1111:u8)
              n761 = Select(t=u8 2, s=w1104, f=w1099) -> (s? t:f=w1096:u8)
              n762 = Select(t=u8 4, s=w1101, f=w1099) -> (s? t:f=w1097:u8)
              n763 = Select(t=u8 2, s=w1120, f=w1115) -> (s? t:f=w1112:u8)
              n764 = Select(t=u8 4, s=w1117, f=w1115) -> (s? t:f=w1113:u8)
              n765 = Compound Arithmetic op=ADD(w1095, w1096, w1097) -> (w1094:u8)
              n766 = Compound Arithmetic op=ADD(w1111, w1112, w1113) -> (w1110:u8)
              n767 = case shown="7" w1110 {
                tunnel: w1092 -> [w1152 w1157 w1159 w1164 w1169 w1171 w1174 w1179]
                tunnel: [w1152 w1158 w1159 w1165 w1170 w1171 w1175 w1180] -> w1107
                tunnel: w1109 -> [_ w1155 _ w1162 w1167 _ w1173 w1178]
                tunnel: w1108 -> [_ w1156 _ w1163 w1168 _ _ _]
                frame 0, Default {
                }
                frame 1 {
                  n768 = Replace Array Subset(array=w1157, new element #1=u16 100 ("new element/subarray"), index #1=w1156, new element #2=u16 1 ("new element/subarray"), index #2=w1155) -> (w1158:u16[])
                }
                frame 2 {
                }
                frame 3 {
                  n769 = Replace Array Subset(array=w1164, new element #1=u16 100 ("new element/subarray"), index #1=w1163, new element #2=u16 1 ("new element/subarray"), index #2=w1162) -> (w1165:u16[])
                }
                frame 4 {
                  w1166 = u16 0 ("new element/subarray")
                  n770 = Replace Array Subset(array=w1169, new element #1=w1166, index #1=w1168, new element #2=w1166, index #2=w1167) -> (w1170:u16[])
                }
                frame 5 {
                }
                frame 6 {
                  n771 = Replace Array Subset(array=w1174, new element=u16 0 ("new element/subarray"), index=w1173) -> (w1175:u16[])
                }
                frame 7 {
                  n772 = local write "RewCalib_Trig_L"(FALSE ("RewCalib_Trig_L")) -> ()
                  n773 = Replace Array Subset(array=w1179, new element=u16 0 ("new element/subarray"), index=w1178) -> (w1180:u16[])
                }
              }
              n774 = case shown="7" w1094 {
                tunnel: w1107 -> [w1123 w1128 w1130 w1135 w1140 w1142 w1145 w1150]
                tunnel: [w1123 w1129 w1130 w1136 w1141 w1142 w1146 w1151] -> w1106
                tunnel: w1090 -> [_ w1126 _ w1133 w1138 _ w1144 w1149]
                tunnel: w1093 -> [_ w1127 _ w1134 w1139 _ _ _]
                frame 0, Default {
                }
                frame 1 {
                  n775 = Replace Array Subset(array=w1128, new element #1=u16 100 ("new element/subarray"), index #1=w1127, new element #2=u16 1 ("new element/subarray"), index #2=w1126) -> (w1129:u16[])
                }
                frame 2 {
                }
                frame 3 {
                  n776 = Replace Array Subset(array=w1135, new element #1=u16 100 ("new element/subarray"), index #1=w1134, new element #2=u16 1 ("new element/subarray"), index #2=w1133) -> (w1136:u16[])
                }
                frame 4 {
                  w1137 = u16 0 ("new element/subarray")
                  n777 = Replace Array Subset(array=w1140, new element #1=w1137, index #1=w1139, new element #2=w1137, index #2=w1138) -> (w1141:u16[])
                }
                frame 5 {
                }
                frame 6 {
                  n778 = Replace Array Subset(array=w1145, new element=u16 0 ("new element/subarray"), index=w1144) -> (w1146:u16[])
                }
                frame 7 {
                  n779 = local write "RewCalib_Trig_R"(FALSE ("RewCalib_Trig_L")) -> ()
                  n780 = Replace Array Subset(array=w1150, new element=u16 0 ("new element/subarray"), index=w1149) -> (w1151:u16[])
                }
              }
            }
            frame "DispenseWater_pre" {
              w1186 = u16 0 ("t")
              w1229 = u16 0 ("new element/subarray")
              # "just trust me on this one"
              # "RewCalib\nOnOff"
              # "RewCalib\nOnOff"
              # "nCycle"
              # "Solenoid__R"
              # "Tdelay"
              # "delay"
              # "nCycle"
              # "Solenoid__L"
              # "Tdelay"
              # "delay"
              # "Solenoid__R"
              # "count"
              # "Solenoid_Tcycle_R"
              # "Solenoid_Tcycle_L"
              # "Solenoid__L"
              # "count"
              n781 = call "myRIO_BRig_RT_dataMTrig_Solenoid_RewCalib_OnOff__L.vi"() -> ("output_Solenoid_RewCalib_OnOff__L"=w1193:i32)  [unwired: 11 in]
              n782 = call "myRIO_BRig_RT_dataMTrig_Solenoid_N__L.vi"() -> ("output_Solenoid_N__L"=w1184:i32)  [unwired: 11 in]
              n783 = call "myRIO_BRig_RT_dataMTrig_Solenoid_delay__L.vi"() -> ("output_Solenoid_delay__L"=w1227:i32)  [unwired: 11 in]
              n784 = call "myRIO_BRig_RT_dataMTrig_Solenoid_Tdelay__L.vi"() -> ("output_Solenoid_Tdelay__L"=w1226:i32)  [unwired: 11 in]
              n785 = call "myRIO_BRig_RT_dataMTrig_Solenoid_N__R.vi"() -> ("output_Solenoid_N__R"=w1182:i32)  [unwired: 11 in]
              n786 = call "myRIO_BRig_RT_dataMTrig_Solenoid_delay__R.vi"() -> ("output_Solenoid_delay__R"=w1216:i32)  [unwired: 11 in]
              n787 = call "myRIO_BRig_RT_dataMTrig_Solenoid_Tdelay__R.vi"() -> ("output_Solenoid_Tdelay__R"=w1215:i32)  [unwired: 11 in]
              n788 = call "myRIO_BRig_RT_dataMTrig_Solenoid_RewCalib_OnOff__R.vi"() -> ("output_Solenoid_RewCalib_OnOff__R"=w1189:i32)  [unwired: 11 in]
              n789 = Index Array(array=w1228, index #1=w1184, index #2=w1227, index #3=w1226, index #4=w1182, index #5=w1216, index #6=w1215, index #7=w1193, index #8=w1189) -> (element #1=w1185:u16, element #2=w1225:u16, element #3=w1220:u16, element #4=w1188:u16, element #5=w1210:u16, element #6=w1209:u16, element #7=w1194:u16, element #8=w1191:u16)
              n790 = Equal To 0?(x=w1225) -> (x = 0?=w1224:bool)
              n791 = Equal To 0?(x=w1210) -> (x = 0?=w1214:bool)
              n792 = local read "RewCalib_Trig_L"() -> (w1205:bool)
              n793 = local read "RewCalib_Trig_R"() -> (w1200:bool)
              n794 = Not Equal To 0?(x=w1185) -> (x != 0?=w1223:bool)
              n795 = Not Equal To 0?(x=w1188) -> (x != 0?=w1213:bool)
              n796 = local read "MTrig_Solenoid_Tcycle__L"() -> (w1222:u16)
              n797 = local read "MTrig_Solenoid_Tcycle__R"() -> (w1208:u16)
              n798 = Not Equal To 0?(x=w1194) -> (x != 0?=w1204:bool)
              n799 = Not Equal To 0?(x=w1191) -> (x != 0?=w1202:bool)
              n800 = Not(x=w1205) -> (.not. x?=w1203:bool)
              n801 = Not(x=w1200) -> (.not. x?=w1201:bool)
              n802 = And(x=w1204, y=w1203) -> (x .and. y?=w1199:bool)
              n803 = And(x=w1202, y=w1201) -> (x .and. y?=w1198:bool)
              n804 = call "myRIO_BRig_RT_dataMTrig_Solenoid_c__L.vi"() -> ("output_Solenoid_c__L"=w1231:i32)  [unwired: 11 in]
              n805 = call "myRIO_BRig_RT_dataMTrig_Solenoid_c__R.vi"() -> ("output_Solenoid_c__R"=w1230:i32)  [unwired: 11 in]
              n806 = Select(t=w1222, s=w1223, f=u16 0) -> (s? t:f=w1219:u16)
              n807 = Or(x=w1199, y=w1198) -> (x .or. y?=w1187:bool)
              n808 = Select(t=w1208, s=w1213, f=u16 0) -> (s? t:f=w1211:u16)
              n809 = Select(t=w1219, s=w1224, f=w1220) -> (s? t:f=w1217:u16)
              n810 = Select(t=w1211, s=w1214, f=w1209) -> (s? t:f=w1206:u16)
              n811 = call "myRIO_BRig_RT_dataMTrig_Solenoid_Tcycle__L.vi"() -> ("output_Solenoid_Tcycle__L"=w1218:i32)  [unwired: 11 in]
              n812 = call "myRIO_BRig_RT_dataMTrig_Solenoid_Tcycle__R.vi"() -> ("output_Solenoid_Tcycle__R"=w1207:i32)  [unwired: 11 in]
              n813 = Select(t=w1186, s=w1187, f=w1185) -> (s? t:f=w1183:u16)
              n814 = Select(t=w1186, s=w1187, f=w1188) -> (s? t:f=w1181:u16)
              n815 = Select(t=myRIO_BRig_RT__Case_NonExp_stateList."Idle" ("Enum"), s=w1187, f=myRIO_BRig_RT__Case_NonExp_stateList."DispenseWater" ("Enum")) -> (s? t:f=w1195:T1)
              n816 = Select(t=w1186, s=w1187, f=w1194) -> (s? t:f=w1192:u16)
              n817 = Select(t=w1186, s=w1187, f=w1191) -> (s? t:f=w1190:u16)
              n818 = Replace Array Subset(array=w1228, new element #1=w1229, index #1=w1231, new element #2=w1229, index #2=w1230, new element #3=w1217, index #3=w1218, new element #4=w1206, index #4=w1207, new element #5=w1192, index #5=w1193, new element #6=w1190, index #6=w1189, new element #7=w1183, index #7=w1184, new element #8=w1181, index #8=w1182) -> (w1232:u16[])
            }
            frame "DispenseWater" {
              # "D"
              # "C"
              # "B"
              # "A"
              # "(A) Add COUNT and INCREMENT\n(B) Is (A) smaller than Tcycle?\n(C) Are we dispensing water or in the delay phase?\n(D) If (A) is smaller than Tcycle   AND   if we are dispensing water\n      then send TRUE to solenoid"
              # "delay"
              # "Tcycle"
              # "Solenoid__R"
              # "count"
              # "delay"
              # "Tcycle"
              # "Solenoid__L"
              # "count"
              n819 = To Unsigned Word Integer(number=w1259) -> (unsigned 16bit integer=w1241:u16)
              n820 = call "myRIO_BRig_RT_dataMTrig_Solenoid_delay__R.vi"() -> ("output_Solenoid_delay__R"=w1245:i32)  [unwired: 11 in]
              n821 = call "myRIO_BRig_RT_dataMTrig_Solenoid_c__R.vi"() -> ("output_Solenoid_c__R"=w1244:i32)  [unwired: 11 in]
              n822 = call "myRIO_BRig_RT_dataMTrig_Solenoid_Tcycle__R.vi"() -> ("output_Solenoid_Tcycle__R"=w1246:i32)  [unwired: 11 in]
              n823 = call "myRIO_BRig_RT_dataMTrig_Solenoid_delay__L.vi"() -> ("output_Solenoid_delay__L"=w1261:i32)  [unwired: 11 in]
              n824 = call "myRIO_BRig_RT_dataMTrig_Solenoid_c__L.vi"() -> ("output_Solenoid_c__L"=w1253:i32)  [unwired: 11 in]
              n825 = call "myRIO_BRig_RT_dataMTrig_Solenoid_Tcycle__L.vi"() -> ("output_Solenoid_Tcycle__L"=w1262:i32)  [unwired: 11 in]
              n826 = Index Array(array=w1255, index #1=w1253, index #2=w1262, index #3=w1261, index #4=w1244, index #5=w1246, index #6=w1245) -> (element #1=w1260:u16, element #2=w1250:u16, element #3=w1258:u16, element #4=w1240:u16, element #5=w1237:u16, element #6=w1236:u16)
              n827 = Add(x=w1260, y=w1241) -> (x+y=w1251:u16)
              n828 = Add(x=w1240, y=w1241) -> (x+y=w1242:u16)
              n829 = Less?(x=w1251, y=w1250) -> (x < y?=w1234:bool)
              n830 = Equal To 0?(x=w1258) -> (x = 0?=w1257:bool)
              n831 = Less?(x=w1242, y=w1237) -> (x < y?=w1235:bool)
              n832 = Equal To 0?(x=w1236) -> (x = 0?=w1243:bool)
              n833 = And(x=w1234, y=w1257) -> (x .and. y?=w1256:bool)
              n834 = Or(x=w1234, y=w1235) -> (x .or. y?=w1233:bool)
              n835 = And(x=w1235, y=w1243) -> (x .and. y?=w1238:bool)
              n836 = Select(t=w1251, s=w1234, f=w1250) -> (s? t:f=w1252:u16)
              n837 = Select(t=w1242, s=w1235, f=w1237) -> (s? t:f=w1239:u16)
              n838 = Replace Array Subset(array=w1255, new element #1=w1252, index #1=w1253, new element #2=w1239, index #2=w1244) -> (w1254:u16[])
              n839 = Select(t=w1249, s=w1233, f=myRIO_BRig_RT__Case_NonExp_stateList."DispenseWater_post" ("Enum")) -> (s? t:f=w1247:T1)
            }
            frame "DispenseWater_post" {
              # "nCycle"
              # "delay"
              # "Solenoid__R"
              # "nCycle"
              # "delay"
              # "Solenoid__L"
              n840 = call "myRIO_BRig_RT_dataMTrig_Solenoid_N__L.vi"() -> ("output_Solenoid_N__L"=w1279:i32)  [unwired: 11 in]
              n841 = call "myRIO_BRig_RT_dataMTrig_Solenoid_delay__L.vi"() -> ("output_Solenoid_delay__L"=w1278:i32)  [unwired: 11 in]
              n842 = call "myRIO_BRig_RT_dataMTrig_Solenoid_N__R.vi"() -> ("output_Solenoid_N__R"=w1275:i32)  [unwired: 11 in]
              n843 = call "myRIO_BRig_RT_dataMTrig_Solenoid_delay__R.vi"() -> ("output_Solenoid_delay__R"=w1274:i32)  [unwired: 11 in]
              n844 = Index Array(array=w1281, index #1=w1279, index #2=w1278, index #3=w1275, index #4=w1274) -> (element #1=w1283:u16, element #2=w1282:u16, element #3=w1266:u16, element #4=w1268:u16)
              n845 = Not Equal To 0?(x=w1283) -> (x != 0?=w1284:bool)
              n846 = Not Equal To 0?(x=w1266) -> (x != 0?=w1267:bool)
              n847 = case shown="True" w1267 {
                selector: w1267 -> [_ w1288]
                tunnel: w1266 -> [w1286 w1294]
                tunnel: w1268 -> [_ w1295]
                tunnel: [w1286 w1292] -> w1265
                tunnel: [u16 0 w1291] -> w1264
                tunnel: [_ w1288] -> w1263
                frame False {
                }
                frame True {
                  n848 = Equal To 0?(x=w1295) -> (x = 0?=w1287:bool)
                  n849 = Decrement(x=w1294) -> (x-1=w1293:u16)
                  n850 = Select(t=w1293, s=w1287, f=w1294) -> (s? t:f=w1292:u16)
                  n851 = Select(t=u16 1, s=w1287, f=u16 0) -> (s? t:f=w1291:u16)
                }
              }
              n852 = case shown="True" w1284 {
                selector: w1284 -> [_ w1299]
                tunnel: w1283 -> [w1297 w1305]
                tunnel: w1282 -> [_ w1306]
                tunnel: [w1297 w1303] -> w1277
                tunnel: [u16 0 w1302] -> w1276
                tunnel: [_ w1299] -> w1273
                frame False {
                }
                frame True {
                  n853 = Equal To 0?(x=w1306) -> (x = 0?=w1298:bool)
                  n854 = Decrement(x=w1305) -> (x-1=w1304:u16)
                  n855 = Select(t=w1304, s=w1298, f=w1305) -> (s? t:f=w1303:u16)
                  n856 = Select(t=u16 1, s=w1298, f=u16 0) -> (s? t:f=w1302:u16)
                }
              }
              n857 = Or(x=w1273, y=w1263) -> (x .or. y?=w1272:bool)
              n858 = Replace Array Subset(array=w1281, new element #1=w1277, index #1=w1279, new element #2=w1276, index #2=w1278, new element #3=w1265, index #3=w1275, new element #4=w1264, index #4=w1274) -> (w1280:u16[])
              n859 = Select(t=myRIO_BRig_RT__Case_NonExp_stateList."DispenseWater_pre" ("Enum"), s=w1272, f=myRIO_BRig_RT__Case_NonExp_stateList."Idle" ("Enum")) -> (s? t:f=w1269:T1)
            }
            frame "TestConnection" {
              n860 = local read "Host Password"() -> (w1312:string)
              n861 = local read "Host UserName"() -> (w1313:string)
              n862 = call "myRIO_BRig_RT_comm_webdav_testConnect.vi"("input_password"=w1312, "input_username"=w1313) -> ("output_Iconnected"=w1310:bool)  [unwired: 9 in]
              n863 = Select(t="Connection accepted!" ("message"), s=w1310, f="Error!") -> (s? t:f=w1308:string)
              n864 = One Button Dialog(message=w1308) -> ()  [unwired: 1 in, 1 out]
            }
            frame "SendData" {
              n865 = local read "Data Set Prefix"() -> (w1315:string)
              n866 = local read "Host Password"() -> (w1316:string)
              n867 = local read "Host UserName"() -> (w1317:string)
              n868 = call "myRIO_BRig_RT_comm_webdav_sendData_all.vi"("Host Filename Prefix"=w1315, "Host Password"=w1316, "Host UserName"=w1317) -> ()  [unwired: 9 in]
            }
            frame "Get_FPGA_count_per_ms" {
              # "Used to automatically determine how many FPGA cycles in 1 ms"
              n869 = case shown="False" w1330 {
                selector: w1330 -> [w1332 _]
                tunnel: w1328 -> [_ w1345]
                tunnel: [w1336 w1345] -> w1327
                tunnel: w1326 -> [w1335 w1343]
                tunnel: w1325 -> [w1334 w1342]
                tunnel: [w1333 w1340] -> w1320
                tunnel: [w1332 w1339] -> w1324
                frame False {
                  n870 = Get Date/Time In Seconds() -> (seconds since 1Jan1904=w1337:timestamp)
                  n871 = xnode "Read/Write Control"("FPGA VI Reference In"=w1335, "error in"=w1334, "timeTrial_trig"=TRUE ("timeTrial")) -> ("error out"=w1333:errorcluster)  [unwired: 1 out]
                  n872 = To Double Precision Float(number=w1337) -> (double precision float=w1336:dbl)
                  n873 = local write "get_countPerMS"(w1332) -> ()
                }
                frame True {
                  w1341 = 1.0
                  n874 = Get Date/Time In Seconds() -> (seconds since 1Jan1904=w1346:timestamp)
                  n875 = To Double Precision Float(number=w1346) -> (double precision float=w1347:dbl)
                  n876 = Subtract(x=w1347, y=w1345) -> (x-y=w1344:dbl)
                  n877 = Less Or Equal?(x=w1341, y=w1344) -> (x <= y?=w1339:bool)
                  n878 = case shown="True" w1339 {
                    tunnel: w1343 -> [_ w1360]
                    tunnel: w1342 -> [w1348 w1359]
                    tunnel: w1341 -> [_ w1350]
                    tunnel: [w1348 w1349] -> w1340
                    frame False {
                    }
                    frame True {
                      n879 = xnode "Read/Write Control"("FPGA VI Reference In"=w1360, "error in"=w1359) -> ("FPGA VI Reference Out"=w1357:refnum<k20>, "error out"=w1356:errorcluster, "timeTrial_count"=w1351:u32)
                      n880 = Multiply(x=w1350, y=1000.0) -> (x*y=w1354:dbl)
                      n881 = To Double Precision Float(number=w1351) -> (double precision float=w1353:dbl)
                      n882 = Divide(x=w1353, y=w1354) -> (x/y=w1355:dbl)
                      n883 = local write "FPGA_count2ms"(w1355) -> ()
                      n884 = xnode "Read/Write Control"("FPGA VI Reference In"=w1357, "error in"=w1356, "timeTrial_trig"=FALSE ("timeTrial")) -> ("error out"=w1349:errorcluster)  [unwired: 1 out]
                    }
                  }
                }
              }
              n885 = Select(t=myRIO_BRig_RT__Case_NonExp_stateList."Idle" ("Enum"), s=w1324, f=w1322) -> (s? t:f=w1321:T1)
              n886 = local write "error out"(w1320) -> ()
            }
            frame "End" {
            }
          }
          n887 = local read "MTrig_Audio_trig__R"() -> (w91:bool)
          n888 = local read "MTrig_Audio_trig__L"() -> (w92:bool)
          n889 = local read "MTrig_Laser_trig"() -> (w90:bool)
          n890 = local read "MTrig_CueLed"() -> (w83:bool)
          n891 = Compound Arithmetic op=OR(w92, w91, w90, w83) -> (w89:bool)
          n892 = local read "START"() -> (w115:bool)
          n893 = local read "STOP_abort"() -> (w114:bool)
          n894 = case shown="True" w89 {
            frame False {
            }
            frame True {
              w131 = FALSE
              n895 = local write "MTrig_Audio_trig__R"(w131) -> ()
              n896 = local write "MTrig_Audio_trig__L"(w131) -> ()
              n897 = local write "MTrig_Laser_trig"(w131) -> ()
              n898 = local write "MTrig_CueLed"(w131) -> ()
            }
          }
          n899 = call "myRIO_BRig_RT_dataMTrig_main__NoExp.vi"("input_dataMTrig"=w118, "input_Audio_trig_L"=w92, "input_Audio_trig_R"=w91, "input_Laser_trig"=w90, "input_CueLed"=w83) -> ("output_dataMTrig"=w117:u16[], "output_Audio_L"=w109:bool, "output_Audio_R"=w110:bool, "output_Laser"=w88:bool, "output_CueLed"=w82:bool)  [unwired: 10 in]
          n900 = Or(x=w115, y=w114) -> (x .or. y?=w113:bool)
          n901 = Select(t=myRIO_BRig_RT__Case_NonExp_stateList."End" ("Enum"), s=w113, f=w112) -> (s? t:f=w111:T1)
          n902 = Not(x="MTrig_Laser_Switch") -> (.not. x?=w85:bool)
          n903 = And(x=w88, y=w85) -> (x .and. y?=w86:bool)
          n904 = And(x=w88, y="MTrig_Laser_Switch") -> (x .and. y?=w87:bool)
          n905 = xnode "Read/Write Control"("FPGA VI Reference In"=w98, "error in"=w97, "A1_SR"=w119, "A3_SL"=w120, "audioTrigger_L"=w109, "audioTrigger_R"=w110, "LC_Laser_l1"=w86, "LC_Laser_l2"=w87, "CueLed_Event"=w82) -> ("FPGA VI Reference Out"=w125:refnum<k20>, "error out"=w124:errorcluster)
          n906 = node-c288() -> ()  [unwired: 1 in, 1 out]
          "cState_NonExp" <- w123
        }
        n907 = node-c288(w70) -> ()  [unwired: 1 out]
        n908 = flat-sequence {
          tunnel: w63 -> [w81]
          tunnel: [w81] -> w62
          tunnel: w61 -> [w80]
          tunnel: [w80] -> w60
          frame #0 {
            w79 = FALSE
            n909 = local write "STOP_endBlock"(w79) -> ()
            n910 = local write "STOP_endTrial"(w79) -> ()
          }
        }
      }
      frame True {
        w1373 = u16 0
        w1390 = u16 0 ("idxDataBlock")
        w1392 = u16 100 ("new element/subarray")
        w1393 = u16 100 ("new element/subarray")
        w1413 = T6 refnum items=["Session NI_WebDAV"] ("output_hSession")
        w1422 = FALSE
        # "dummyState counter"
        # "audio__L\naudio__R"
        # "Audio params"
        # "nRewards"
        # "idxDataBlock"
        # "Solenoid_Tdelay_R"
        # "Solenoid_Tdelay_L"
        # "RewCalib_N__R"
        # "RewCalib_N__L"
        # "Save dataLick to file\nSend file to Host\nSave dataMTrig\nSend file to Host\nDisconnect"
        # "dataTrial"
        # "dataTrial"
        # "Solenoid_Tcycle_R"
        # "Solenoid_Tcycle_L"
        # "Laser_Tcycle"
        # "Audio_Tcycle_R"
        # "Audio_Tcycle_L"
        # "dataLick"
        # "dataLC"
        # "dataLC"
        # "dataBlock"
        # "dataBlock"
        # "dataMTrig"
        # "dataMTrig"
        # "dataExp"
        # "dataCurrent"
        # "dataExp"
        # "dataCurrent"
        # "spout"
        # "state"
        n911 = call "myRIO_BRig_RT_dataMTrig_Solenoid_Tcycle__L.vi"() -> ("output_Solenoid_Tcycle__L"=w1419:i32)  [unwired: 11 in]
        n912 = call "myRIO_BRig_RT_dataMTrig_Solenoid_Tcycle__R.vi"() -> ("output_Solenoid_Tcycle__R"=w1418:i32)  [unwired: 11 in]
        n913 = call "myRIO_BRig_RT_dataMTrig_Audio_Tcycle__L.vi"() -> ("output_Audio_Tcycle__L"=w1417:i32)  [unwired: 11 in]
        n914 = call "myRIO_BRig_RT_dataMTrig_Audio_Tcycle__R.vi"() -> ("output_Audio_Tcycle__R"=w1416:i32)  [unwired: 11 in]
        n915 = call "myRIO_BRig_RT_dataMTrig_Laser_Tcycle.vi"() -> ("output_Laser_Tcycle"=w1415:i32)  [unwired: 11 in]
        n916 = local read "Tcycle_Reward_min_L"() -> (w1394:u16)
        n917 = local read "Tcycle_Reward_min_R"() -> (w1395:u16)
        n918 = local read "MTrig_Solenoid_Tcycle__L"() -> (w1398:u16)
        n919 = local read "MTrig_Solenoid_Tcycle__R"() -> (w1397:u16)
        n920 = local read "MTrig_Laser_Tcycle"() -> (w1396:u16)
        n921 = call "myRIO_BRig_RT_dataMTrig_Solenoid_RewCalib_nCycle__L.vi"() -> ("output_Solenoid_RewCalib_nCycle__L"=w1401:i32)  [unwired: 11 in]
        n922 = call "myRIO_BRig_RT_dataMTrig_Solenoid_Tdelay__L.vi"() -> ("output_Solenoid_Tdelay__L"=w1403:i32)  [unwired: 11 in]
        n923 = call "myRIO_BRig_RT_dataMTrig_Solenoid_RewCalib_nCycle__R.vi"() -> ("output_Solenoid_RewCalib_nCycle__R"=w1402:i32)  [unwired: 11 in]
        n924 = call "myRIO_BRig_RT_dataMTrig_Solenoid_Tdelay__R.vi"() -> ("output_Solenoid_Tdelay__R"=w1404:i32)  [unwired: 11 in]
        n925 = case shown="False" w1383 {
          selector: w1383 -> [_ w1444]
          tunnel: w1382 -> [w1441 w1446]
          tunnel: [w1442 w1446] -> w1378
          tunnel: w1381 -> [_ w1445]
          tunnel: [w1443 w1445] -> w1379
          tunnel: [w1440 w1444] -> w1377
          frame False {
            n926 = call "myRIO__TCP_connect_forWriting.vi"("input_error"=w1441) -> ("output_error"=w1442:errorcluster, "output_connected"=w1440:bool, "output_hTCP"=w1443:refnum<k5>)  [unwired: 8 in]
          }
          frame True {
          }
        }
        n927 = call "myRIO_BRig_RT_dataLick_init.vi"() -> ("output_dataLick"=w1424:u16[][])  [unwired: 11 in]
        n928 = call "myRIO_BRig_RT_dataCurrent_init.vi"() -> ("output_dataCurrent"=w1431:u16[])  [unwired: 11 in]
        n929 = call "myRIO_BRig_RT_dataExp_init.vi"() -> ("output_dataExp"=w1430:u16[])  [unwired: 11 in]
        n930 = call "myRIO_BRig_RT_dataMTrig_init.vi"() -> ("output_dataMTrig"=w1421:u16[])  [unwired: 5 in]
        n931 = call "myRIO_BRig_RT_dataLC_init.vi"() -> ("output_dataLC"=w1428:u16[])  [unwired: 11 in]
        n932 = call "myRIO_BRig_RT_dataBlock_init.vi"() -> ("output_dataBlock"=w1429:u16[][])  [unwired: 11 in]
        n933 = call "myRIO_BRig_RT_dataTrial_init.vi"() -> ("output_dataTrial"=w1414:u16[][])  [unwired: 11 in]
        n934 = local write "I_connect_TCP"(w1377) -> ()
        n935 = Replace Array Subset(array=w1421, new element #1=w1393, index #1=w1401, new element #2=w1393, index #2=w1402, new element #3=w1392, index #3=w1403, new element #4=w1392, index #4=w1404, new element #5=w1398, index #5=w1419, new element #6=w1397, index #6=w1418, new element #7=w1394, index #7=w1417, new element #8=w1395, index #8=w1416, new element #9=w1396, index #9=w1415) -> (w1420:u16[])
        n936 = call "myRIO_BRig_RT_dataAnalog_init.vi"() -> ("output_dataAnalog"=w1388:u16[][])  [unwired: 11 in]
        n937 = call "myRIO_BRig_RT_TCP__start_exp.vi"("input_hTCP"=w1379, "input_I_connected_TCP"=w1377, "input_error"=w1378) -> ("output_hTCP"=w1376:refnum<k5>, "output_error"=w1375:errorcluster)  [unwired: 11 in]
        n938 = Get Date/Time In Seconds() -> (seconds since 1Jan1904=w1400:timestamp)
        n939 = call "myRIO_BRig_RT_arrTrig_init.vi"() -> ("output_arrTrig"=w1372:bool[])  [unwired: 11 in]
        n940 = To Double Precision Float(number=w1400) -> (double precision float=w1399:dbl)
        n941 = node-c288() -> (w1439:T3)  [unwired: 4 in]
        n942 = timed-loop {
          timing: w1439 -> [_]
          timing-out: [_] -> w1438
          shift-right: [w1573] -> _
          shift-left: myRIO_BRig_RT__Case_Exp_stateList."Start1" ("Enum") -> [w1497]
          shift-right: [w1531] -> _
          shift-left: enum16{"Left", "Right"}."Left" -> [w1613]
          tunnel: w1371 -> [w1611]
          tunnel: w1370 -> [w1503]
          shift-right: [w1606] -> _
          shift-left: w1436 -> [w1610]
          shift-right: [w1605] -> _
          shift-left: w1435 -> [w1609]
          tunnel: [w1589] -> w1433
          tunnel: [w1590] -> w1434
          shift-right: [w1591] -> w1405
          shift-left: w1431 -> [w1492]
          shift-right: [w1604] -> _
          shift-left: w1430 -> [w1564]
          shift-right: [w1585] -> w1409
          shift-left: w1420 -> [w1586]
          shift-right: [w1602] -> _
          shift-left: w1429 -> [w1603]
          shift-right: [w1600] -> _
          shift-left: w1428 -> [w1601]
          shift-right: [w1592] -> w1411
          shift-left: w1424 -> [w1593]
          shift-right: [w1562] -> _
          shift-left: w1422 -> [w1587]
          shift-right: [w1563] -> _
          shift-left: w1422 -> [w1588]
          shift-right: [w1571] -> _
          shift-left: w1414 -> [w1572]
          shift-right: [w1570] -> w1407
          shift-left: w1413 -> [w1568]
          shift-right: [w1569] -> w1408
          shift-left: FALSE ("output_Iconnected") -> [w1567]
          tunnel: "Data Set Prefix" -> [w1566]
          tunnel: [w1566] -> w1406
          tunnel: w1399 -> [w1565]
          shift-right: [w1560] -> _
          shift-left: 0 ("idxDataBlock") -> [w1561]
          shift-right: [w1557] -> _
          shift-left: w1390 -> [w1559]
          shift-right: [w1556] -> _
          shift-left: w1390 -> [w1558]
          shift-right: [w1550] -> w1386
          shift-left: 0 -> [w1536]
          shift-right: [w1532] -> _
          shift-left: w1373 -> [w1545]
          shift-right: [w1533] -> _
          shift-left: w1373 -> [w1542]
          shift-right: [w1541] -> _
          shift-left: w1373 -> [w1548]
          shift-right: [w1551] -> w1387
          shift-left: w1388 -> [w1552]
          tunnel: w1376 -> [w1540]
          tunnel: [w1539] -> w1385
          tunnel: w1377 -> [w1537]
          tunnel: [w1537] -> w1384
          tunnel: w1375 -> [w1538]
          tunnel: [w1500] -> w1380
          shift-right: [w1529] -> _
          shift-left: u16 0 -> [w1530]
          shift-right: [w1527] -> _
          shift-left: w1373 -> [w1528]
          shift-right: [w1524] -> _
          shift-left: w1372 -> [w1525]
          shift-right: [w1495] -> _
          shift-left: FALSE -> [w1498]
          stop <- w1599 stop-if-true
          # "arrTrig"
          # "arrTrig"
          # "LC_Laser_l2"
          # "LC_Event_l2"
          # "LC_Laser_l1"
          # "LC_Event_l1"
          # "CueLed"
          # "LC_Laser_l2"
          # "LC_Event_l2"
          # "LC_Laser_l1"
          # "LC_Event_l1"
          # "solenoid__R"
          # "solenoid__L"
          # "spout"
          # "iState"
          # "dataAnalog"
          # "index"
          # "iEvent"
          # "iBlock"
          # "iTrial"
          # "Laser"
          # "Audio R"
          # "Audio L"
          # "Solenoid R"
          # "Solenoid L"
          # "manual triggering"
          # "dataTrial"
          # "dataBlock"
          # "nRewards"
          # "dataExp"
          # "dataCurrent"
          # "audio__L\naudio__R"
          # "time stamp"
          # "nRewards"
          # "idxDataBlock"
          # "idxDataBlock"
          # "audio__L\naudio__R"
          # "dataLC"
          # "solenoid__R"
          # "solenoid__L"
          # "Did a lick occur?"
          # "Update lick counter"
          # "spout"
          # "spout"
          # "state"
          # "state"
          n943 = node-c288() -> ()  [unwired: 1 in, 1 out]
          n944 = flat-sequence {
            tunnel: w1503 -> [w1614]
            tunnel: [w1614] -> _
            tunnel: [w1615] -> w1499
            tunnel: [w1614] -> w1502
            frame #0 {
              n945 = Get Date/Time In Seconds() -> (seconds since 1Jan1904=w1615:timestamp)
            }
          }
          n946 = xnode "Read/Write Control"("FPGA VI Reference In"=w1611, "error in"=w1502) -> ("FPGA VI Reference Out"=w1555:refnum<k20>, "error out"=w1554:errorcluster, "A2_LickL"=w1606:u32, "A4_LickR"=w1605:u32)
          "A2" <- w1606
          "A4" <- w1605
          n947 = Greater?(x=w1606, y=w1610) -> (0:w1608:bool)
          n948 = Greater?(x=w1605, y=w1609) -> (0:w1607:bool)
          n949 = call "myRIO_BRig_RT_dataCurrent_IallReward_L.vi"() -> ("output_IallReward_L"=w1493:i32)  [unwired: 11 in]
          n950 = call "myRIO_BRig_RT_dataCurrent_IallReward_R.vi"() -> ("output_IallReward_R"=w1494:i32)  [unwired: 11 in]
          n951 = Or(x=w1608, y=w1607) -> (x .or. y?=w1612:bool)
          n952 = local read "MTrig_Solenoid_trig__L"() -> (w1583:bool)
          n953 = local read "MTrig_Solenoid_trig__R"() -> (w1582:bool)
          n954 = local read "MTrig_Audio_trig__L"() -> (w1581:bool)
          n955 = local read "MTrig_Audio_trig__R"() -> (w1580:bool)
          n956 = local read "MTrig_Laser_trig"() -> (w1579:bool)
          n957 = Index Array(array=w1492, index #1=w1493, index #2=w1494) -> (element #1=w1490:u16, element #2=w1491:u16)
          n958 = Not Equal To 0?(x=w1490) -> (x != 0?=→"allReward_L":bool)
          n959 = Not Equal To 0?(x=w1491) -> (x != 0?=→"allReward_R":bool)
          n960 = case shown="\"Selection\"" w1497 {
            selector: w1497 -> [_ _ _ _ _ _ _ _ _ _ _ _ _ _ _ _ _ _ _ _ _ _ _ _ _ w2582 _ w2625 _ _ _ _ _ w2722 _ w2782 _ _ _ _ _ w2885 _ w2937 _ w2992 _ w3032 _ _ w3090 _ _ _ _ _ w3237 _ _ _ _ _ _ _ _ _ _ _ _ w3470 w3499]
            tunnel: [myRIO_BRig_RT__Case_Exp_stateList."Start2" ("Enum") myRIO_BRig_RT__Case_Exp_stateList."Start3" ("Enum") myRIO_BRig_RT__Case_Exp_stateList."saveSettings1" ("Enum") myRIO_BRig_RT__Case_Exp_stateList."saveSettings2" ("Enum") myRIO_BRig_RT__Case_Exp_stateList."saveSettings3" ("Enum") myRIO_BRig_RT__Case_Exp_stateList."saveSettings4" ("Enum") myRIO_BRig_RT__Case_Exp_stateList."saveSettings_LC_ENL_l1" ("Enum") myRIO_BRig_RT__Case_Exp_stateList."saveSettings_LC_ENL_l2" ("Enum") myRIO_BRig_RT__Case_Exp_stateList."saveSettings_LC_Cue_l1" ("Enum") myRIO_BRig_RT__Case_Exp_stateList."saveSettings_LC_Cue_l2" ("Enum") myRIO_BRig_RT__Case_Exp_stateList."saveSettings6_LC_l1_Other" ("Enum") myRIO_BRig_RT__Case_Exp_stateList."SaveSettings6_LC_l2_Other" ("Enum") myRIO_BRig_RT__Case_Exp_stateList."setSettings_Audio" ("Enum") myRIO_BRig_RT__Case_Exp_stateList."setSettings_Laser" ("Enum") myRIO_BRig_RT__Case_Exp_stateList."commConnect" ("Enum") w2339 myRIO_BRig_RT__Case_Exp_stateList."initTrial" ("Enum") w2393 myRIO_BRig_RT__Case_Exp_stateList."initTrial3" ("Enum") myRIO_BRig_RT__Case_Exp_stateList."initTrial_LC_ENL1" ("Enum") myRIO_BRig_RT__Case_Exp_stateList."ENL1_pre" ("Enum") myRIO_BRig_RT__Case_Exp_stateList."initTrial_LC_Cue1" ("Enum") myRIO_BRig_RT__Case_Exp_stateList."initTrial_LC_Sel" ("Enum") myRIO_BRig_RT__Case_Exp_stateList."initTrial4" ("Enum") w2557 w2579 myRIO_BRig_RT__Case_Exp_stateList."ENL1Penalty" ("Enum") w2626 myRIO_BRig_RT__Case_Exp_stateList."endExp" ("Enum") myRIO_BRig_RT__Case_Exp_stateList."endExp" ("Enum") myRIO_BRig_RT__Case_Exp_stateList."endExp" ("Enum") myRIO_BRig_RT__Case_Exp_stateList."endExp" ("Enum") w2699 w2716 myRIO_BRig_RT__Case_Exp_stateList."Cue1Penalty" ("Enum") w2780 myRIO_BRig_RT__Case_Exp_stateList."endExp" ("Enum") myRIO_BRig_RT__Case_Exp_stateList."endExp" ("Enum") myRIO_BRig_RT__Case_Exp_stateList."endExp" ("Enum") myRIO_BRig_RT__Case_Exp_stateList."endExp" ("Enum") w2858 w2884 myRIO_BRig_RT__Case_Exp_stateList."SelectReward" ("Enum") w2938 myRIO_BRig_RT__Case_Exp_stateList."SelectRewardPost" ("Enum") w2993 myRIO_BRig_RT__Case_Exp_stateList."SelectWrong" ("Enum") w3028 myRIO_BRig_RT__Case_Exp_stateList."endTrial1" ("Enum") myRIO_BRig_RT__Case_Exp_stateList."SelectTimeout" ("Enum") w3092 myRIO_BRig_RT__Case_Exp_stateList."endTrial1" ("Enum") myRIO_BRig_RT__Case_Exp_stateList."endTrial2" ("Enum") myRIO_BRig_RT__Case_Exp_stateList."endTrial3" ("Enum") w3162 w3220 w3237 myRIO_BRig_RT__Case_Exp_stateList."initBlock" ("Enum") w3260 myRIO_BRig_RT__Case_Exp_stateList."commUpload_dataExp" ("Enum") myRIO_BRig_RT__Case_Exp_stateList."endBlock" ("Enum") myRIO_BRig_RT__Case_Exp_stateList."commUpload_dataLC" ("Enum") myRIO_BRig_RT__Case_Exp_stateList."commUpload_dataTrial" ("Enum") myRIO_BRig_RT__Case_Exp_stateList."commUpload_dataCurrent" ("Enum") myRIO_BRig_RT__Case_Exp_stateList."saveData_dataCurrent" ("Enum") myRIO_BRig_RT__Case_Exp_stateList."saveData_dataExp" ("Enum") myRIO_BRig_RT__Case_Exp_stateList."saveData_dataLC" ("Enum") myRIO_BRig_RT__Case_Exp_stateList."saveData_dataTrial" ("Enum") myRIO_BRig_RT__Case_Exp_stateList."commUpload_pre" ("Enum") w3469 w3498] -> w1573
            tunnel: [w1644 w1659 w1677 w1740 w1798 w1860 w1919 w1979 w2039 w2099 w2159 w2198 w2238 w2267 w2330 w2338 w2363 w2380 w2410 w2452 w2480 w2501 w2520 w2543 w2567 w2591 w2612 w2630 w2642 w2660 w2675 w2690 w2698 w2738 w2762 w2779 w2796 w2813 w2828 w2843 w2867 w2899 w2920 w2935 w2948 w2990 w3010 w3038 w3055 w3071 w3098 w3117 w3129 w3145 w3182 w3197 w3236 w3249 w3263 w3289 w3306 w3323 w3340 w3357 w3381 w3397 w3420 w3436 w3456 w3486 w3515] -> w1531
            tunnel: w1613 -> [w1644 w1659 w1677 w1740 w1798 w1860 w1919 w1979 w2039 w2099 w2159 w2198 w2238 w2267 w2330 w2340 w2363 w2380 w2410 w2452 w2480 w2501 w2520 w2543 w2567 w2591 w2612 w2630 w2642 w2660 w2675 w2690 w2698 w2738 w2762 w2779 w2796 w2813 w2828 w2843 w2867 w2899 w2920 w2935 w2948 w2990 w3010 w3038 w3055 w3071 w3098 w3117 w3129 w3145 w3182 w3197 w3236 w3249 w3263 w3289 w3306 w3323 w3340 w3357 w3381 w3397 w3420 w3436 w3456 w3486 w3515]
            tunnel: w1612 -> [w1647 w1662 w1674 w1743 w1801 w1863 w1922 w1982 w2042 w2102 w2162 w2201 w2241 w2270 w2333 w2355 w2370 w2394 w2429 w2463 w2490 w2509 w2529 w2552 w2558 w2578 w2615 w2633 w2648 w2663 w2678 w2693 w2702 w2721 w2768 w2786 w2801 w2816 w2831 w2846 w2866 w2898 w2925 w2944 w2975 w2998 w3021 w3041 w3054 w3083 w3103 w3114 w3133 w3144 w3189 w3219 w3240 w3246 w3268 w3292 w3309 w3326 w3343 w3360 w3384 w3400 w3423 w3439 w3459 w3489 w3518]
            tunnel: w1608 -> [w1646 w1661 w1675 w1742 w1800 w1862 w1921 w1981 w2041 w2101 w2161 w2200 w2240 w2269 w2332 w2354 w2369 w2395 w2428 w2464 w2491 w2510 w2530 w2553 w2571 w2593 w2614 w2632 w2647 w2662 w2677 w2692 w2712 w2739 w2767 w2785 w2800 w2815 w2830 w2845 w2848 w2874 w2924 w2943 w2974 w2997 w3020 w3040 w3053 w3082 w3102 w3115 w3134 w3143 w3188 w3218 w3239 w3247 w3269 w3291 w3308 w3325 w3342 w3359 w3383 w3399 w3422 w3438 w3458 w3488 w3517]
            tunnel: w1607 -> [w1645 w1660 w1676 w1741 w1799 w1861 w1920 w1980 w2040 w2100 w2160 w2199 w2239 w2268 w2331 w2353 w2368 w2396 w2427 w2465 w2492 w2511 w2531 w2554 w2570 w2592 w2613 w2631 w2646 w2661 w2676 w2691 w2711 w2740 w2766 w2784 w2799 w2814 w2829 w2844 w2847 w2873 w2923 w2942 w2973 w2996 w3019 w3039 w3052 w3081 w3101 w3116 w3135 w3142 w3187 w3217 w3238 w3248 w3270 w3290 w3307 w3324 w3341 w3358 w3382 w3398 w3421 w3437 w3457 w3487 w3516]
            tunnel: [w1647 w1662 w1674 w1743 w1801 w1863 w1922 w1982 w2042 w2102 w2162 w2201 w2241 w2270 w2333 w2355 w2370 w2394 w2429 w2463 w2490 w2509 w2529 w2552 w2558 w2578 w2615 w2633 w2648 w2663 w2678 w2693 w2702 w2721 w2768 w2786 w2801 w2816 w2831 w2846 w2866 w2898 w2925 w2944 w2975 w2998 w3021 w3041 w3054 w3083 w3103 w3114 w3133 w3144 w3189 w3219 w3240 w3246 w3268 w3292 w3309 w3326 w3343 w3360 w3384 w3400 w3423 w3439 w3459 w3489 w3518] -> w1596
            tunnel: [w1646 w1661 w1675 w1742 w1800 w1862 w1921 w1981 w2041 w2101 w2161 w2200 w2240 w2269 w2332 w2354 w2369 w2395 w2428 w2464 w2491 w2510 w2530 w2553 w2571 w2593 w2614 w2632 w2647 w2662 w2677 w2692 w2712 w2739 w2767 w2785 w2800 w2815 w2830 w2845 w2848 w2874 w2924 w2943 w2974 w2997 w3020 w3040 w3053 w3082 w3102 w3115 w3134 w3143 w3188 w3218 w3239 w3247 w3269 w3291 w3308 w3325 w3342 w3359 w3383 w3399 w3422 w3438 w3458 w3488 w3517] -> w1595
            tunnel: [w1645 w1660 w1676 w1741 w1799 w1861 w1920 w1980 w2040 w2100 w2160 w2199 w2239 w2268 w2331 w2353 w2368 w2396 w2427 w2465 w2492 w2511 w2531 w2554 w2570 w2592 w2613 w2631 w2646 w2661 w2676 w2691 w2711 w2740 w2766 w2784 w2799 w2814 w2829 w2844 w2847 w2873 w2923 w2942 w2973 w2996 w3019 w3039 w3052 w3081 w3101 w3116 w3135 w3142 w3187 w3217 w3238 w3248 w3270 w3290 w3307 w3324 w3341 w3358 w3382 w3398 w3421 w3437 w3457 w3487 w3516] -> w1594
            tunnel: w1492 -> [w1643 w1658 w1673 w1707 w1783 w1802 w1864 w1978 w2038 w2098 w2158 w2197 w2237 w2265 w2284 w2346 w2362 w2392 w2399 w2441 w2479 w2500 w2519 w2542 w2559 w2581 w2606 w2629 w2643 w2659 w2674 w2689 w2701 w2723 w2761 w2783 w2797 w2812 w2827 w2842 w2860 w2887 w2900 w2940 w2950 w2995 w3011 w3037 w3051 w3072 w3100 w3113 w3126 w3147 w3164 w3195 w3235 w3250 w3271 w3286 w3303 w3320 w3337 w3348 w3374 w3389 w3409 w3433 w3449 w3468 w3497]
            tunnel: w1564 -> [w1642 w1657 w1672 w1738 w1796 w1857 w1916 w1976 w2036 w2096 w2156 w2195 w2235 w2258 w2276 w2343 w2367 w2391 w2397 w2436 w2482 w2493 w2523 w2546 w2569 w2590 w2605 w2627 w2645 w2658 w2673 w2688 w2697 w2737 w2759 w2778 w2798 w2811 w2826 w2841 w2850 w2875 w2921 w2927 w2967 w2991 w3012 w3035 w3050 w3074 w3097 w3112 w3132 w3136 w3163 w3210 w3234 w3251 w3272 w3285 w3302 w3319 w3336 w3349 w3378 w3394 w3405 w3432 w3453 w3483 w3512]
            tunnel: [w1643 w1658 w1673 w1707 w1783 w1802 w1864 w1978 w2038 w2098 w2158 w2197 w2237 w2265 w2283 w2345 w2362 w2385 w2398 w2440 w2479 w2499 w2518 w2541 w2556 w2580 w2607 w2628 w2643 w2659 w2674 w2689 w2700 w2717 w2760 w2781 w2797 w2812 w2827 w2842 w2859 w2886 w2922 w2939 w2968 w2994 w3013 w3036 w3051 w3075 w3099 w3113 w3125 w3146 w3164 w3193 w3235 w3250 w3271 w3286 w3303 w3320 w3337 w3348 w3374 w3389 w3409 w3433 w3449 w3468 w3497] -> w1505
            tunnel: [w1642 w1657 w1672 w1737 w1795 w1852 w1915 w1976 w2036 w2096 w2156 w2195 w2235 w2258 w2275 w2344 w2367 w2390 w2397 w2436 w2482 w2493 w2523 w2546 w2569 w2590 w2605 w2627 w2645 w2658 w2673 w2688 w2697 w2737 w2759 w2778 w2798 w2811 w2826 w2841 w2850 w2875 w2921 w2927 w2967 w2991 w3012 w3035 w3050 w3074 w3097 w3112 w3132 w3136 w3163 w3210 w3234 w3251 w3272 w3285 w3302 w3319 w3336 w3349 w3378 w3394 w3408 w3432 w3453 w3483 w3512] -> w1604
            tunnel: [_ _ _ _ _ _ _ _ _ _ _ _ _ _ _ _ _ _ _ _ _ _ _ _ _ _ _ _ _ _ _ _ _ _ _ _ _ _ _ _ _ _ _ w2933 _ _ _ _ _ _ _ _ _ _ _ _ _ _ _ _ _ _ _ _ _ _ _ _ _ _ _] -> w1522
            tunnel: [_ _ _ _ _ _ _ _ _ _ _ _ _ _ _ _ _ _ _ _ _ _ _ _ _ _ _ _ _ _ _ _ _ _ _ _ _ _ _ _ _ _ _ w2934 _ _ _ _ _ _ _ _ _ _ _ _ _ _ _ _ _ _ _ _ _ _ _ _ _ _ _] -> w1576
            tunnel: w1603 -> [w1640 w1655 w1670 w1709 w1785 w1858 w1917 w1977 w2037 w2097 w2157 w2196 w2236 w2263 w2327 w2335 w2364 w2375 w2420 w2461 w2488 w2496 w2515 w2538 w2568 w2589 w2602 w2623 w2644 w2656 w2671 w2686 w2710 w2736 w2758 w2776 w2794 w2809 w2824 w2839 w2872 w2896 w2918 w2941 w2952 w2988 w3009 w3033 w3048 w3073 w3096 w3110 w3128 w3151 w3185 w3206 w3232 w3253 w3274 w3283 w3300 w3317 w3334 w3354 w3368 w3391 w3415 w3430 w3451 w3481 w3510]
            tunnel: [w1640 w1655 w1670 w1709 w1785 w1858 w1917 w1977 w2037 w2097 w2157 w2196 w2236 w2263 w2327 w2334 w2361 w2375 w2420 w2461 w2488 w2496 w2515 w2538 w2568 w2589 w2602 w2623 w2644 w2656 w2671 w2686 w2710 w2736 w2758 w2776 w2794 w2809 w2824 w2839 w2872 w2896 w2918 w2941 w2951 w2988 w3009 w3033 w3048 w3073 w3096 w3110 w3127 w3151 w3185 w3206 w3232 w3253 w3274 w3283 w3300 w3317 w3334 w3354 w3368 w3391 w3415 w3430 w3451 w3481 w3510] -> w1602
            tunnel: w1601 -> [w1641 w1656 w1671 w1708 w1784 w1859 w1918 w1974 w2034 w2094 w2154 w2193 w2233 w2264 w2328 w2356 w2366 w2389 w2409 w2462 w2489 w2502 w2521 w2544 w2566 w2577 w2603 w2624 w2641 w2657 w2672 w2687 w2709 w2725 w2757 w2777 w2795 w2810 w2825 w2840 w2871 w2897 w2919 w2936 w2965 w2989 w3008 w3034 w3049 w3070 w3095 w3111 w3131 w3150 w3186 w3209 w3233 w3252 w3273 w3284 w3301 w3318 w3335 w3355 w3377 w3393 w3417 w3428 w3452 w3482 w3511]
            tunnel: [w1641 w1656 w1671 w1708 w1784 w1859 w1918 w1975 w2035 w2095 w2155 w2194 w2234 w2264 w2328 w2356 w2366 w2389 w2409 w2462 w2489 w2502 w2521 w2544 w2566 w2577 w2603 w2624 w2641 w2657 w2672 w2687 w2709 w2725 w2757 w2777 w2795 w2810 w2825 w2840 w2871 w2897 w2919 w2936 w2965 w2989 w3008 w3034 w3049 w3070 w3095 w3111 w3131 w3150 w3186 w3209 w3233 w3252 w3273 w3284 w3301 w3318 w3335 w3355 w3377 w3393 w3417 w3428 w3452 w3482 w3511] -> w1600
            tunnel: [_ _ _ _ _ _ _ _ _ _ _ _ _ _ _ _ _ _ _ _ _ _ _ _ _ _ _ _ _ _ _ _ _ _ _ _ _ _ _ _ _ _ _ _ _ _ _ _ _ _ _ _ _ _ _ _ TRUE _ _ _ _ _ _ _ _ _ _ _ _ _ _] -> w1597
            tunnel: w1588 -> [_ _ _ _ _ _ _ _ _ _ _ _ _ _ _ _ _ _ _ _ _ _ _ _ _ _ _ _ _ _ _ _ _ w2735 _ _ _ _ _ _ _ _ _ _ _ _ _ _ _ _ _ _ _ _ _ _ _ _ _ _ _ _ _ _ _ _ _ _ _ _ _]
            tunnel: w1587 -> [_ _ _ _ _ _ _ _ _ _ _ _ _ _ _ _ _ _ _ _ _ _ _ _ _ _ _ _ _ _ _ _ _ w2734 _ _ _ _ _ _ _ _ _ _ _ _ _ _ _ _ _ _ _ _ _ _ _ _ _ _ _ _ _ _ _ _ _ _ _ _ _]
            tunnel: [_ _ _ _ _ _ _ _ _ _ _ _ _ _ _ _ _ _ _ _ _ _ _ _ _ _ _ _ _ _ _ _ w2696 w2735 _ _ _ _ _ _ _ _ _ _ _ _ _ _ _ _ _ _ _ _ _ _ _ _ _ _ _ _ _ _ _ _ _ _ _ _ _] -> w1563
            tunnel: [_ _ _ _ _ _ _ _ _ _ _ _ _ _ _ _ _ _ _ _ _ _ _ _ _ _ _ _ _ _ _ _ w2695 w2734 _ _ _ _ _ _ _ _ _ _ _ _ _ _ _ _ _ _ _ _ _ _ _ _ _ _ _ _ _ _ _ _ _ _ _ _ _] -> w1562
            tunnel: w1572 -> [w1638 w1653 w1668 w1699 w1781 w1847 w1914 w1961 w2026 w2081 w2141 w2168 w2218 w2257 w2326 w2352 w2365 w2388 w2412 w2454 w2478 w2498 w2517 w2540 w2565 w2588 w2600 w2622 w2639 w2654 w2669 w2684 w2708 w2733 w2755 w2775 w2792 w2807 w2822 w2837 w2870 w2895 w2908 w2926 w2963 w2987 w3004 w3027 w3047 w3066 w3089 w3109 w3124 w3149 w3178 w3205 w3230 w3254 w3275 w3282 w3299 w3316 w3333 w3353 w3376 w3392 w3416 w3431 w3446 w3480 w3509]
            tunnel: [w1638 w1653 w1668 w1699 w1781 w1847 w1914 w1961 w2026 w2081 w2141 w2168 w2218 w2257 w2326 w2352 w2365 w2388 w2411 w2453 w2471 w2497 w2516 w2539 w2565 w2588 w2600 w2622 w2639 w2654 w2669 w2684 w2708 w2733 w2755 w2775 w2792 w2807 w2822 w2837 w2870 w2895 w2908 w2926 w2963 w2987 w3004 w3027 w3047 w3066 w3089 w3109 w3124 w3148 w3178 w3205 w3230 w3254 w3275 w3282 w3299 w3316 w3333 w3353 w3376 w3392 w3416 w3431 w3446 w3480 w3509] -> w1571
            tunnel: [w1637 w1652 w1667 w1698 w1780 w1846 w1913 w1960 w2025 w2080 w2140 w2167 w2217 w2256 w2325 w2351 w2372 w2387 w2422 w2460 w2487 w2508 w2528 w2551 w2564 w2587 w2599 w2621 w2638 w2653 w2668 w2683 w2707 w2732 w2754 w2774 w2791 w2806 w2821 w2836 w2869 w2894 w2907 w2932 w2962 w2986 w3003 w3026 w3046 w3065 w3088 w3108 w3123 w3141 w3184 w3204 w3228 w3255 w3265 w3281 w3298 w3315 w3332 w3352 w3380 w3396 w3419 w3435 w3455 w3485 w3514] -> w1570
            tunnel: [w1636 w1651 w1666 w1697 w1779 w1845 w1912 w1959 w2024 w2079 w2139 w2166 w2216 w2255 w2324 w2350 w2371 w2386 w2421 w2459 w2486 w2507 w2527 w2550 w2563 w2586 w2598 w2620 w2637 w2652 w2667 w2682 w2706 w2731 w2753 w2773 w2790 w2805 w2820 w2835 w2868 w2893 w2906 w2931 w2961 w2985 w3002 w3025 w3045 w3064 w3087 w3107 w3122 w3140 w3183 w3203 w3229 w3241 w3262 w3287 w3304 w3321 w3338 w3356 w3379 w3395 w3418 w3434 w3454 w3484 w3513] -> w1569
            tunnel: w1568 -> [w1637 w1652 w1667 w1698 w1780 w1846 w1913 w1960 w2025 w2080 w2140 w2167 w2217 w2256 w2325 w2351 w2372 w2387 w2422 w2460 w2487 w2508 w2528 w2551 w2564 w2587 w2599 w2621 w2638 w2653 w2668 w2683 w2707 w2732 w2754 w2774 w2791 w2806 w2821 w2836 w2869 w2894 w2907 w2932 w2962 w2986 w3003 w3026 w3046 w3065 w3088 w3108 w3123 w3141 w3184 w3204 w3228 _ w3265 w3281 w3298 w3315 w3332 w3352 w3380 w3396 w3419 w3435 w3455 w3485 w3514]
            tunnel: w1567 -> [w1636 w1651 w1666 w1697 w1779 w1845 w1912 w1959 w2024 w2079 w2139 w2166 w2216 w2255 w2324 w2350 w2371 w2386 w2421 w2459 w2486 w2507 w2527 w2550 w2563 w2586 w2598 w2620 w2637 w2652 w2667 w2682 w2706 w2731 w2753 w2773 w2790 w2805 w2820 w2835 w2868 w2893 w2906 w2931 w2961 w2985 w3002 w3025 w3045 w3064 w3087 w3107 w3122 w3140 w3183 w3203 w3229 _ w3262 w3287 w3304 w3321 w3338 w3356 w3379 w3395 w3418 w3434 w3454 w3484 w3513]
            tunnel: w1566 -> [_ _ _ _ _ _ _ _ _ _ _ _ _ _ _ _ _ _ _ _ _ _ _ _ _ _ _ _ _ _ _ _ _ _ _ _ _ _ _ _ _ _ _ _ _ _ _ _ _ _ _ _ _ _ _ _ _ _ _ w3279 w3296 w3313 w3330 w3350 _ _ _ _ _ _ _]
            tunnel: w1565 -> [_ _ _ _ _ _ _ _ _ _ _ _ _ _ _ _ _ _ _ _ _ _ _ _ _ _ _ _ _ _ _ _ _ _ _ _ _ _ _ _ _ _ _ _ _ _ _ _ _ _ _ _ _ _ _ _ _ _ _ _ _ _ _ _ _ _ w3410 _ _ _ _]
            tunnel: [w1635 w1650 w1665 w1696 w1778 w1844 w1911 w1958 w2023 w2078 w2138 w2165 w2215 w2254 w2323 w2341 w2359 w2384 w2423 w2458 w2485 w2506 w2526 w2549 w2562 w2585 w2597 w2619 w2636 w2651 w2666 w2681 w2705 w2730 w2752 w2772 w2789 w2804 w2819 w2834 w2865 w2892 w2905 w2930 w2946 w2984 w3001 w3024 w3044 w3063 w3086 w3106 w3121 w3139 w3181 w3190 w3227 w3244 w3264 w3278 w3295 w3312 w3329 w3347 w3363 w3388 w3404 w3427 w3444 w3479 w3508] -> w1560
            tunnel: w1561 -> [w1635 w1650 w1665 w1696 w1778 w1844 w1911 w1958 w2023 w2078 w2138 w2165 w2215 w2254 w2323 _ _ w2384 w2423 w2458 w2485 w2506 w2526 w2549 w2562 w2585 w2597 w2619 w2636 w2651 w2666 w2681 w2705 w2730 w2752 w2772 w2789 w2804 w2819 w2834 w2865 w2892 w2905 w2930 w2946 w2984 w3001 w3024 w3044 w3063 w3086 w3106 w3121 w3139 w3181 w3191 w3227 w3244 w3264 w3278 w3295 w3312 w3329 w3347 w3363 w3388 w3404 w3427 w3444 w3479 w3508]
            tunnel: w1559 -> [w1634 w1649 w1664 w1695 w1777 w1843 w1910 w1957 w2022 w2077 w2137 w2164 w2214 w2253 w2322 w2349 w2358 w2383 w2419 w2457 w2484 w2505 w2525 w2548 w2561 w2584 w2596 w2618 w2635 w2650 w2665 w2680 w2704 w2729 w2751 w2771 w2788 w2803 w2818 w2833 w2864 w2891 w2904 w2929 w2960 w2983 w3000 w3023 w3043 w3062 w3085 w3105 w3120 w3138 w3180 w3202 w3226 w3243 w3267 w3277 w3294 w3311 w3328 w3346 w3362 w3387 w3403 w3426 w3443 w3478 w3507]
            tunnel: w1558 -> [w1633 w1648 w1663 w1694 w1776 w1842 w1909 w1956 w2021 w2076 w2136 w2163 w2213 w2252 w2321 w2348 w2357 w2382 w2418 w2456 w2483 w2504 w2524 w2547 w2560 w2583 w2595 w2617 w2634 w2649 w2664 w2679 w2703 w2728 w2750 w2770 w2787 w2802 w2817 w2832 w2863 w2890 w2903 w2928 w2957 w2982 w2999 w3022 w3042 w3061 w3084 w3104 w3119 w3137 w3179 w3201 w3225 w3242 w3266 w3276 w3293 w3310 w3327 w3345 w3361 w3386 w3402 w3425 w3442 w3477 w3506]
            tunnel: [w1634 w1649 w1664 w1695 w1777 w1843 w1910 w1957 w2022 w2077 w2137 w2164 w2214 w2253 w2322 w2349 w2358 w2383 w2419 w2457 w2484 w2505 w2525 w2548 w2561 w2584 w2596 w2618 w2635 w2650 w2665 w2680 w2704 w2729 w2751 w2771 w2788 w2803 w2818 w2833 w2864 w2891 w2904 w2929 w2959 w2983 w3000 w3023 w3043 w3062 w3085 w3105 w3120 w3138 w3180 w3202 w3226 w3243 w3267 w3277 w3294 w3311 w3328 w3346 w3362 w3387 w3403 w3426 w3443 w3478 w3507] -> w1557
            tunnel: [w1633 w1648 w1663 w1694 w1776 w1842 w1909 w1956 w2021 w2076 w2136 w2163 w2213 w2252 w2321 w2348 w2357 w2382 w2418 w2456 w2483 w2504 w2524 w2547 w2560 w2583 w2595 w2617 w2634 w2649 w2664 w2679 w2703 w2728 w2750 w2770 w2787 w2802 w2817 w2832 w2863 w2890 w2903 w2928 w2958 w2982 w2999 w3022 w3042 w3061 w3084 w3104 w3119 w3137 w3179 w3201 w3225 w3242 w3266 w3276 w3293 w3310 w3327 w3345 w3361 w3386 w3402 w3425 w3442 w3477 w3506] -> w1556
            tunnel: w1555 -> [w1632 _ _ _ _ _ _ _ _ _ _ _ _ w2249 w2318 _ _ w2379 w2426 w2448 w2469 _ _ w2534 _ _ _ _ _ _ _ _ _ w2727 _ _ _ _ _ _ w2861 w2889 _ _ _ _ _ _ _ w3060 _ _ _ _ w3160 _ w3223 _ _ _ _ _ _ _ _ _ _ _ _ _ _]
            tunnel: w1554 -> [w1631 _ _ _ _ _ _ _ _ _ _ _ _ w2248 w2319 _ _ w2378 w2425 w2447 w2468 _ _ w2533 _ _ _ _ _ _ _ _ _ w2726 _ _ _ _ _ _ w2862 w2888 _ _ _ _ _ _ _ w3059 _ _ _ _ w3159 _ w3222 _ _ _ _ _ _ _ _ _ _ _ _ _ _]
            tunnel: [_ _ _ _ _ _ _ _ _ _ _ _ _ _ _ _ _ _ _ _ _ _ _ _ _ w2575 _ _ _ _ _ _ _ w2713 _ _ _ _ _ _ w2854 w2880 _ _ _ _ _ _ _ _ _ _ _ _ _ _ _ _ _ _ _ _ _ _ _ _ _ _ _ _ _] -> w1513
            tunnel: [_ _ _ _ _ _ _ _ _ _ _ _ _ _ _ _ _ _ _ _ _ _ _ _ _ w2574 _ _ _ _ _ _ _ w2714 _ _ _ _ _ _ w2853 w2879 _ _ _ _ _ _ _ _ _ _ _ _ _ _ _ _ _ _ _ _ _ _ _ _ _ _ _ _ _] -> w1512
            tunnel: [_ _ _ _ _ _ _ _ _ _ _ _ _ _ _ _ _ _ _ _ _ _ TRUE ("Recording") _ _ _ _ _ _ _ _ _ _ _ _ _ _ _ _ _ _ _ _ _ _ _ _ _ _ _ _ _ _ _ _ _ _ _ _ _ _ _ _ _ _ _ _ _ _ _ _] -> w1549
            tunnel: [_ _ _ _ _ _ _ _ _ _ _ _ _ _ _ TRUE _ _ _ _ _ _ _ _ _ _ _ _ _ _ _ _ _ _ _ _ _ _ _ _ _ _ _ _ _ _ _ _ _ _ _ _ _ _ _ _ _ _ _ _ _ _ _ _ _ _ _ _ _ _ _] -> w1546
            tunnel: [_ _ _ _ _ _ _ _ _ _ _ _ _ _ _ _ _ TRUE _ _ _ _ _ _ _ _ _ _ _ _ _ _ _ _ _ _ _ _ _ _ _ _ _ _ _ _ _ _ _ _ _ _ _ _ _ _ _ _ _ _ _ _ _ _ _ _ _ _ _ _ _] -> w1544
            tunnel: [_ _ _ _ _ _ _ _ _ _ _ _ _ _ _ _ _ w2374 _ _ _ _ _ _ _ _ _ _ _ _ _ _ _ _ _ _ _ _ _ _ _ _ _ _ _ _ _ _ _ _ _ _ _ _ _ _ _ _ _ _ _ _ _ _ _ _ _ _ _ _ _] -> w1543
            tunnel: w1530 -> [_ _ _ _ _ _ _ _ _ _ _ _ _ _ _ _ _ _ _ _ _ _ _ _ _ _ _ _ _ _ _ _ _ _ _ _ _ _ _ _ _ _ _ _ _ _ _ _ _ _ _ _ _ _ _ _ _ _ _ _ _ _ _ _ _ _ _ _ _ w3475 w3504]
            tunnel: [_ _ _ _ _ _ _ _ _ _ _ _ _ _ _ _ _ _ _ _ _ _ _ _ _ _ _ _ _ _ _ _ _ _ _ _ _ _ _ _ _ _ _ _ _ _ _ _ _ _ _ _ _ _ _ _ _ _ _ _ _ _ _ _ _ _ _ _ _ w3473 w3502] -> w1529
            tunnel: w1525 -> [_ _ _ _ _ _ _ _ _ _ _ _ _ _ _ _ _ _ _ _ w2470 w2495 w2514 w2537 w2555 w2576 w2594 w2616 _ _ _ _ w2694 w2724 w2749 w2769 _ _ _ _ w2855 w2881 _ _ _ _ _ _ _ _ _ _ _ _ _ _ _ _ _ _ _ _ _ _ _ _ _ _ _ _ _]
            tunnel: [_ _ _ _ _ _ _ _ _ _ _ _ _ _ _ _ _ _ _ w2438 w2470 w2494 w2513 w2536 w2555 w2576 w2594 w2616 _ _ _ _ w2694 w2724 w2749 w2769 _ _ _ _ w2855 w2881 _ _ _ _ _ _ _ _ _ _ _ _ _ _ _ _ _ _ _ _ _ _ _ _ _ _ _ _ _] -> w1524
            tunnel: [_ _ _ _ _ _ _ _ _ _ _ _ _ _ _ _ _ _ _ _ _ _ _ _ _ w2573 _ _ _ _ _ _ _ w2718 _ _ _ _ _ _ w2852 w2878 _ _ _ _ _ _ _ _ _ _ _ _ _ _ _ _ _ _ _ _ _ _ _ _ _ _ _ _ _] -> w1517
            tunnel: [_ _ _ _ _ _ _ _ _ _ _ _ _ _ _ _ _ _ _ _ _ _ _ _ _ w2572 _ _ _ _ _ _ _ w2719 _ _ _ _ _ _ w2851 w2877 _ _ _ _ _ _ _ _ _ _ _ _ _ _ _ _ _ _ _ _ _ _ _ _ _ _ _ _ _] -> w1515
            tunnel: [_ _ _ _ _ _ _ _ _ _ _ _ _ _ _ _ _ _ _ _ _ _ _ _ _ _ _ _ _ _ _ _ _ w2720 _ _ _ _ _ _ _ _ _ _ _ _ _ _ _ _ _ _ _ _ _ _ _ _ _ _ _ _ _ _ _ _ _ _ _ _ _] -> w1521
            tunnel: [_ _ _ _ _ _ _ _ _ _ _ _ _ _ _ w2336 _ _ _ _ _ _ _ _ _ _ _ _ _ _ _ _ _ _ _ _ _ _ _ _ _ _ _ _ _ _ _ _ _ _ _ _ _ _ _ _ _ _ _ _ _ _ _ _ _ _ _ _ _ _ _] -> w1504
            frame "Start1", Default {
              w1630 = FALSE ("SelectionState")
              n961 = local read "CueLed_baseline"() -> (w1629:bool)
              n962 = local read "Laser2_baseline"() -> (w1628:bool)
              n963 = local read "Laser1_baseline"() -> (w1627:bool)
              n964 = xnode "Read/Write Control"("FPGA VI Reference In"=w1632, "error in"=w1631, "SelectionState"=w1630, "LR_reward_Laser_l1"=w1630, "LR_wrong_Laser_l1"=w1630, "LR_reward_Event_l1"=w1630, "LR_wrong_Event_l1"=w1630, "Left(F)_or_Right(T)"=w1630, "ignoreWrong"=w1630, "SelectionState"=w1630, "LR_reward_Laser_l2"=w1630, "LR_wrong_laser_l2"=w1630, "LR_reward_Event_l2"=w1630, "LR_wrong_Event_l2"=w1630, "LC_Event_l1"=w1630, "LC_Laser_l1"=w1630, "LC_Laser_l2"=w1630, "LC_Event_l2"=w1630, "CueLed_Event"=w1630, "I_allReward"=w1630, "CueLed_Baseline"=w1629, "L2Led_Baseline"=w1628, "L1Led_Baseline"=w1627) -> ()  [unwired: 2 out]
            }
            frame "Start2" {
            }
            frame "Start3" {
            }
            frame "saveSettings1" {
              n965 = call "myRIO_BRig_RT_dataExp_Tcycle_Reward_min_L.vi"() -> ("output_Tcycle_Reward_min_L"=w1683:i32)  [unwired: 11 in]
              n966 = local read "Tcycle_Reward_min_L"() -> (w1682:u16)
              n967 = call "myRIO_BRig_RT_dataExp_Audio_freq__L.vi"() -> ("output_Audio_freq__L"=w1715:i32)  [unwired: 11 in]
              n968 = call "myRIO_BRig_RT_dataExp_Audio_freq__R.vi"() -> ("output_Audio_freq__R"=w1714:i32)  [unwired: 11 in]
              n969 = call "myRIO_BRig_RT_dataExp_Audio_amp__L.vi"() -> ("output_Audio_amp__L"=w1713:i32)  [unwired: 11 in]
              n970 = call "myRIO_BRig_RT_dataExp_Audio_amp__R.vi"() -> ("output_Audio_amp__R"=w1711:i32)  [unwired: 11 in]
              n971 = call "myRIO_BRig_RT_dataExp_TPB_min__L.vi"() -> ("output_TPB_min__L"=w1723:i32)  [unwired: 11 in]
              n972 = call "myRIO_BRig_RT_dataExp_TPB_min__R.vi"() -> ("output_TPB_min__R"=w1721:i32)  [unwired: 11 in]
              n973 = call "myRIO_BRig_RT_dataExp_TPB_max__L.vi"() -> ("output_TPB_max__L"=w1719:i32)  [unwired: 11 in]
              n974 = call "myRIO_BRig_RT_dataExp_TPB_max__R.vi"() -> ("output_TPB_max__R"=w1717:i32)  [unwired: 11 in]
              n975 = call "myRIO_BRig_RT_dataExp_Cue1Param_AudioLed_Count_Switch.vi"() -> ("output_Cue1Param_AudioLed_Count_Switch"=w1689:i32)  [unwired: 11 in]
              n976 = call "myRIO_BRig_RT_dataExp_Cue1Param_AudioLed_Probability_Switch.vi"() -> ("output_Cue1Param_AudioLed_Probability_Switch"=w1687:i32)  [unwired: 11 in]
              n977 = call "myRIO_BRig_RT_dataExp_Cue1Param_CueType_Switch.vi"() -> ("output_Cue1Param_CueType_Switch"=w1685:i32)  [unwired: 11 in]
              n978 = call "myRIO_BRig_RT_dataExp_ItrialUntilReward.vi"() -> ("output_I_trialUntilReward"=w1736:i32)  [unwired: 11 in]
              n979 = call "myRIO_BRig_RT_dataExp_IblockUntilReward.vi"() -> ("output_I_blockUntilReward"=w1732:i32)  [unwired: 11 in]
              n980 = call "myRIO_BRig_RT_dataExp_CueCycles.vi"() -> ("output_CueCycles"=w1731:i32)  [unwired: 11 in]
              n981 = call "myRIO_BRig_RT_dataExp_ENL_min.vi"() -> ("output_ENL_min"=w1729:i32)  [unwired: 11 in]
              n982 = call "myRIO_BRig_RT_dataExp_ENL_max.vi"() -> ("output_ENL_max"=w1727:i32)  [unwired: 11 in]
              n983 = call "myRIO_BRig_RT_dataExp_ENL_penalty.vi"() -> ("output_ENL_penalty"=w1725:i32)  [unwired: 11 in]
              n984 = local read "Audio_Freq__L"() -> (w1693:u8)
              n985 = local read "Audio_Freq__R"() -> (w1691:u8)
              n986 = local read "Audio_Amp__L"() -> (w1712:u16)
              n987 = local read "TpB_Min_L"() -> (w1722:u16)
              n988 = local read "TpB_Min_R"() -> (w1720:u16)
              n989 = local read "TpB_Max_L"() -> (w1718:u16)
              n990 = local read "TpB_Max_R"() -> (w1716:u16)
              n991 = local read "Audio_Amp__R"() -> (w1710:u16)
              n992 = local read "TrialUntilReward"() -> (w1735:bool)
              n993 = local read "CueCycles"() -> (w1730:u16)
              n994 = local read "Tcycle_ENL_min"() -> (w1728:u16)
              n995 = local read "Tcycle_ENL_max"() -> (w1726:u16)
              n996 = local read "Tcycle_ENLPenalty"() -> (w1724:u16)
              n997 = local read "Cue1Param_AudioLed_Count_Switch"() -> (w1688:u16)
              n998 = local read "Cue1Param_AudioLed_Probability_Switch"() -> (w1686:u16)
              n999 = local read "Cue1Param_CueType_Switch"() -> (w1684:u16)
              n1000 = local read "Tcycle_Reward_max_L"() -> (w1680:u16)
              n1001 = call "myRIO_BRig_RT_dataExp_Tcycle_Reward_max_L.vi"() -> ("output_Tcycle_Reward_max_L"=w1681:i32)  [unwired: 11 in]
              n1002 = To Unsigned Word Integer(number=w1691) -> (unsigned 16bit integer=w1690:u16)
              n1003 = To Unsigned Word Integer(number=w1693) -> (unsigned 16bit integer=w1692:u16)
              n1004 = Boolean To (0,1)(Boolean=w1735) -> (0, 1=w1734:i16)
              n1005 = To Unsigned Word Integer(number=w1734) -> (unsigned 16bit integer=w1733:u16)
              n1006 = call "myRIO_BRig_RT_dataExp_Tcycle_Reward_step_L.vi"() -> ("output_Tcycle_Reward_step_L"=w1679:i32)  [unwired: 11 in]
              n1007 = local read "Tcycle_Reward_step_L"() -> (w1678:u16)
              n1008 = local read "BUR_min"() -> (w1704:u16)
              n1009 = local read "BUR_max"() -> (w1705:u16)
              n1010 = Not Equal To 0?(x=w1704) -> (x != 0?=w1703:bool)
              n1011 = Not Equal To 0?(x=w1705) -> (x != 0?=w1702:bool)
              n1012 = And(x=w1703, y=w1702) -> (x .and. y?=w1701:bool)
              n1013 = Boolean To (0,1)(Boolean=w1701) -> (0, 1=w1706:i16)
              n1014 = To Unsigned Word Integer(number=w1706) -> (unsigned 16bit integer=w1700:u16)
              n1015 = Replace Array Subset(array=w1738, new element #1=w1733, index #1=w1736, new element #2=w1700, index #2=w1732, new element #3=w1730, index #3=w1731, new element #4=w1728, index #4=w1729, new element #5=w1726, index #5=w1727, new element #6=w1724, index #6=w1725, new element #7=w1722, index #7=w1723, new element #8=w1720, index #8=w1721, new element #9=w1718, index #9=w1719, new element #10=w1716, index #10=w1717, new element #11=w1692, index #11=w1715, new element #12=w1690, index #12=w1714, new element #13=w1712, index #13=w1713, new element #14=w1710, index #14=w1711, new element #15=w1688, index #15=w1689, new element #16=w1686, index #16=w1687, new element #17=w1684, index #17=w1685, new element #18=w1682, index #18=w1683, new element #19=w1680, index #19=w1681, new element #20=w1678, index #20=w1679) -> (w1737:u16[])
            }
            frame "saveSettings2" {
              n1016 = call "myRIO_BRig_RT_dataExp_Tcycle_Reward_min_R.vi"() -> ("output_Tcycle_Reward_min_R"=w1757:i32)  [unwired: 11 in]
              n1017 = local read "Tcycle_Reward_min_R"() -> (w1756:u16)
              n1018 = call "myRIO_BRig_RT_dataExp_Tcycle_Cue1_Audio_min.vi"() -> ("output_Tcycle_Cue1_Audio_min"=w1788:i32)  [unwired: 11 in]
              n1019 = call "myRIO_BRig_RT_dataExp_Tcycle_Cue1_Audio_max.vi"() -> ("output_Tcycle_Cue1_Audio_max"=w1787:i32)  [unwired: 11 in]
              n1020 = call "myRIO_BRig_RT_dataExp_Tcycle_Cue1Penalty_Audio.vi"() -> ("output_Tcycle_Cue1Penalty_Audio"=w1786:i32)  [unwired: 11 in]
              n1021 = call "myRIO_BRig_RT_dataExp_Tcycle_RewardPost.vi"() -> ("output_Tcycle_RewardPost"=w1794:i32)  [unwired: 11 in]
              n1022 = call "myRIO_BRig_RT_dataExp_Tcycle_Wrong.vi"() -> ("output_Tcycle_Wrong"=w1792:i32)  [unwired: 11 in]
              n1023 = call "myRIO_BRig_RT_dataExp_Tcycle_Timeout.vi"() -> ("output_Tcycle_Timeout"=w1790:i32)  [unwired: 11 in]
              n1024 = call "myRIO_BRig_RT_dataExp_Tcycle_Cue1_LED_min.vi"() -> ("output_Tcycle_Cue1_LED_min"=w1763:i32)  [unwired: 11 in]
              n1025 = call "myRIO_BRig_RT_dataExp_Tcycle_Cue1_LED_max.vi"() -> ("output_Tcycle_Cue1_LED_max"=w1762:i32)  [unwired: 11 in]
              n1026 = call "myRIO_BRig_RT_dataExp_Tcycle_Cue1Penalty_LED.vi"() -> ("output_Tcycle_Cue1Penalty_LED"=w1761:i32)  [unwired: 11 in]
              n1027 = call "myRIO_BRig_RT_dataExp_SolenoidProbability_L.vi"() -> ("output_SolenoidProbability_L"=w1773:i32)  [unwired: 11 in]
              n1028 = call "myRIO_BRig_RT_dataExp_SolenoidProbability_R.vi"() -> ("output_SolenoidProbability_R"=w1772:i32)  [unwired: 11 in]
              n1029 = call "myRIO_BRig_RT_dataExp_Cue1Param_AudioLed_Count_NS.vi"() -> ("output_Cue1Param_AudioLed_Count_NS"=w1769:i32)  [unwired: 11 in]
              n1030 = call "myRIO_BRig_RT_dataExp_Cue1Param_AudioLed_Probability_NS.vi"() -> ("output_Cue1Param_AudioLed_Probability_NS"=w1767:i32)  [unwired: 11 in]
              n1031 = call "myRIO_BRig_RT_dataExp_Cue1Param_CueType_NS.vi"() -> ("output_Cue1Param_CueType_NS"=w1765:i32)  [unwired: 11 in]
              n1032 = call "myRIO_BRig_RT_dataExp_nBlock.vi"() -> ("output_nBlock"=w1744:i32)  [unwired: 11 in]
              n1033 = call "myRIO_BRig_RT_dataExp_nTrial.vi"() -> ("output_nTrial"=w1746:i32)  [unwired: 11 in]
              n1034 = call "myRIO_BRig_RT_dataExp_runTime_seconds.vi"() -> ("output_RunTime_minutes"=w1749:i32)  [unwired: 11 in]
              n1035 = call "myRIO_BRig_RT_dataExp_Tcycle_Selection.vi"() -> ("output_Tcycle_Selection"=w1751:i32)  [unwired: 11 in]
              n1036 = local read "Tcycle_CuePenalty_Audio"() -> (w1782:u16)
              n1037 = local read "Tcycle_Cue_Audio_max"() -> (w1774:u16)
              n1038 = local read "Tcycle_Cue_Audio_min"() -> (w1775:u16)
              n1039 = local read "Tcycle_RewardPost"() -> (w1793:u16)
              n1040 = local read "Tcycle_Wrong"() -> (w1791:u16)
              n1041 = local read "Tcycle_Timeout"() -> (w1789:u16)
              n1042 = local read "Tcycle_Selection"() -> (w1750:u16)
              n1043 = local read "Cue1Param_AudioLed_Count_NS"() -> (w1768:u16)
              n1044 = local read "Cue1Param_AudioLed_Probability_NS"() -> (w1766:u16)
              n1045 = local read "Cue1Param_CueType_NS"() -> (w1764:u16)
              n1046 = local read "Tcycle_CuePenalty_LED"() -> (w1758:u16)
              n1047 = local read "SolenoidProbability_R"() -> (w1770:u16)
              n1048 = local read "SolenoidProbability_L"() -> (w1771:u16)
              n1049 = local read "Tcycle_Cue_LED_min"() -> (w1760:u16)
              n1050 = local read "Tcycle_Cue_LED_max"() -> (w1759:u16)
              n1051 = local read "Tcycle_Reward_max_R"() -> (w1754:u16)
              n1052 = call "myRIO_BRig_RT_dataExp_Tcycle_Reward_max_R.vi"() -> ("output_Tcycle_Reward_max_R"=w1755:i32)  [unwired: 11 in]
              n1053 = call "myRIO_BRig_RT_dataExp_Tcycle_Reward_step_R.vi"() -> ("output_Tcycle_Reward_step_R"=w1753:i32)  [unwired: 11 in]
              n1054 = local read "Tcycle_Reward_step_R"() -> (w1752:u16)
              n1055 = Replace Array Subset(array=w1796, new element #1=u16 0, index #1=w1744, new element #2=u16 0, index #2=w1746, new element #3=u16 0, index #3=w1749, new element #4=w1750, index #4=w1751, new element #5=w1793, index #5=w1794, new element #6=w1791, index #6=w1792, new element #7=w1789, index #7=w1790, new element #8=w1775, index #8=w1788, new element #9=w1774, index #9=w1787, new element #10=w1782, index #10=w1786, new element #11=w1771, index #11=w1773, new element #12=w1770, index #12=w1772, new element #13=w1768, index #13=w1769, new element #14=w1766, index #14=w1767, new element #15=w1764, index #15=w1765, new element #16=w1760, index #16=w1763, new element #17=w1759, index #17=w1762, new element #18=w1758, index #18=w1761, new element #19=w1756, index #19=w1757, new element #20=w1754, index #20=w1755, new element #21=w1752, index #21=w1753) -> (w1795:u16[])
            }
            frame "saveSettings3" {
              w1808 = 100.0 ("y")
              n1056 = call "myRIO_BRig_RT_dataExp_laser1_Freq.vi"() -> ("output_laser1_Freq"=w1841:i32)  [unwired: 11 in]
              n1057 = call "myRIO_BRig_RT_dataExp_laser1_Tpeak.vi"() -> ("output_laser1_Tpeak"=w1836:i32)  [unwired: 11 in]
              n1058 = call "myRIO_BRig_RT_dataExp_laser1_Tshutter.vi"() -> ("output_laser1_Tshutter"=w1831:i32)  [unwired: 11 in]
              n1059 = call "myRIO_BRig_RT_dataExp_FPGA_f_count2ms.vi"() -> ("output_FPGA_f_count2ms"=w1826:i32)  [unwired: 11 in]
              n1060 = call "myRIO_BRig_RT_dataExp_laser1_Power_min.vi"() -> ("output_laser1_Power_min"=w1821:i32)  [unwired: 11 in]
              n1061 = call "myRIO_BRig_RT_dataExp_laser1_Power_max.vi"() -> ("output_laser1_Power_max"=w1814:i32)  [unwired: 11 in]
              n1062 = call "myRIO_BRig_RT_dataExp_laser1_Power_step.vi"() -> ("output_laser1_Power_step"=w1813:i32)  [unwired: 11 in]
              n1063 = call "myRIO_BRig_RT_dataExp_laser1_duration.vi"() -> ("output_laser1_duration"=w1816:i32)  [unwired: 11 in]
              n1064 = local read "Laser_Tshutter_l1"() -> (w1828:dbl)
              n1065 = local read "Laser_Tpeak_l1"() -> (w1833:dbl)
              n1066 = local read "Laser_power_max_l1"() -> (w1807:dbl)
              n1067 = local read "Laser_power_step_l1"() -> (w1806:dbl)
              n1068 = local read "Laser_power_min_l1"() -> (w1818:dbl)
              n1069 = local read "Laser_Freq_l1"() -> (w1840:dbl)
              n1070 = call "myRIO_BRig_RT_dataExp_BUR_min.vi"() -> ("output_BUR_min"=w1856:i32)  [unwired: 11 in]
              n1071 = call "myRIO_BRig_RT_dataExp_BUR_max.vi"() -> ("output_BUR_max"=w1854:i32)  [unwired: 11 in]
              n1072 = call "myRIO_BRig_RT_dataExp_Audio_sp__L.vi"() -> ("output_Audio_sp__L"=w1851:i32)  [unwired: 11 in]
              n1073 = call "myRIO_BRig_RT_dataExp_Audio_sp__R.vi"() -> ("output_Audio_sp__R"=w1850:i32)  [unwired: 11 in]
              n1074 = local read "FPGA_count2ms"() -> (w1823:dbl)
              n1075 = local read "sp_LeftSpout"() -> (w1849:u16)
              n1076 = local read "BUR_max"() -> (w1853:u16)
              n1077 = local read "sp_RightSpout"() -> (w1848:u16)
              n1078 = local read "BUR_min"() -> (w1855:u16)
              n1079 = Multiply(x=w1840, y=w1808) -> (x*y=w1839:dbl)
              n1080 = Multiply(x=w1833, y=w1808) -> (x*y=w1835:dbl)
              n1081 = Multiply(x=w1828, y=w1808) -> (x*y=w1830:dbl)
              n1082 = Multiply(x=w1823, y=w1808) -> (x*y=w1825:dbl)
              n1083 = Multiply(x=w1818, y=w1808) -> (x*y=w1820:dbl)
              n1084 = Multiply(x=w1807, y=w1808) -> (x*y=w1812:dbl)
              n1085 = Multiply(x=w1806, y=w1808) -> (x*y=w1810:dbl)
              n1086 = Round To Nearest(number=w1839) -> (nearest integer value=w1838:dbl)
              n1087 = Round To Nearest(number=w1835) -> (nearest integer value=w1834:dbl)
              n1088 = Round To Nearest(number=w1830) -> (nearest integer value=w1829:dbl)
              n1089 = Round To Nearest(number=w1825) -> (nearest integer value=w1824:dbl)
              n1090 = Round To Nearest(number=w1820) -> (nearest integer value=w1819:dbl)
              n1091 = Round To Nearest(number=w1812) -> (nearest integer value=w1811:dbl)
              n1092 = Round To Nearest(number=w1810) -> (nearest integer value=w1809:dbl)
              n1093 = To Unsigned Word Integer(number=w1838) -> (unsigned 16bit integer=w1837:u16)
              n1094 = To Unsigned Word Integer(number=w1834) -> (unsigned 16bit integer=w1832:u16)
              n1095 = To Unsigned Word Integer(number=w1829) -> (unsigned 16bit integer=w1827:u16)
              n1096 = To Unsigned Word Integer(number=w1824) -> (unsigned 16bit integer=w1822:u16)
              n1097 = To Unsigned Word Integer(number=w1819) -> (unsigned 16bit integer=w1817:u16)
              n1098 = To Unsigned Word Integer(number=w1811) -> (unsigned 16bit integer=w1805:u16)
              n1099 = To Unsigned Word Integer(number=w1809) -> (unsigned 16bit integer=w1804:u16)
              n1100 = local read "Laser_duration_l1"() -> (w1815:u16)
              n1101 = Replace Array Subset(array=w1857, new element #1=w1855, index #1=w1856, new element #2=w1853, index #2=w1854, new element #3=w1849, index #3=w1851, new element #4=w1848, index #4=w1850, new element #5=w1837, index #5=w1841, new element #6=w1832, index #6=w1836, new element #7=w1827, index #7=w1831, new element #8=w1822, index #8=w1826, new element #9=w1817, index #9=w1821, new element #10=w1805, index #10=w1814, new element #11=w1804, index #11=w1813, new element #12=w1815, index #12=w1816) -> (w1852:u16[])
            }
            frame "saveSettings4" {
              w1877 = 100.0 ("y")
              n1102 = call "myRIO_BRig_RT_dataExp_laser2_Freq.vi"() -> ("output_laser2_Freq"=w1866:i32)  [unwired: 11 in]
              n1103 = call "myRIO_BRig_RT_dataExp_laser2_Tpeak.vi"() -> ("output_laser2_Tpeak"=w1868:i32)  [unwired: 11 in]
              n1104 = call "myRIO_BRig_RT_dataExp_laser2_Tshutter.vi"() -> ("output_laser2_Tshutter"=w1870:i32)  [unwired: 11 in]
              n1105 = call "myRIO_BRig_RT_dataExp_laser2_Power_min.vi"() -> ("output_laser2_Power_min"=w1885:i32)  [unwired: 11 in]
              n1106 = call "myRIO_BRig_RT_dataExp_laser2_Power_max.vi"() -> ("output_laser2_Power_max"=w1884:i32)  [unwired: 11 in]
              n1107 = call "myRIO_BRig_RT_dataExp_laser2_Power_step.vi"() -> ("output_laser2_Power_step"=w1883:i32)  [unwired: 11 in]
              n1108 = call "myRIO_BRig_RT_dataExp_laser2_duration.vi"() -> ("output_laser2_duration"=w1882:i32)  [unwired: 11 in]
              n1109 = call "myRIO_BRig_RT_dataExp_CueLed_Freq.vi"() -> ("output_CueLed_Freq"=w1874:i32)  [unwired: 11 in]
              n1110 = call "myRIO_BRig_RT_dataExp_CueLed_Tpeak.vi"() -> ("output_CueLed_Tpeak"=w1873:i32)  [unwired: 11 in]
              n1111 = local read "Laser_Tshutter_l2"() -> (w1900:dbl)
              n1112 = local read "Laser_Tpeak_l2"() -> (w1903:dbl)
              n1113 = local read "Laser_power_max_l2"() -> (w1890:dbl)
              n1114 = local read "Laser_power_step_l2"() -> (w1889:dbl)
              n1115 = local read "Laser_power_min_l2"() -> (w1897:dbl)
              n1116 = local read "Laser_Freq_l2"() -> (w1908:dbl)
              n1117 = local read "CueLed_Tpeak"() -> (w1875:dbl)
              n1118 = local read "CueLed_Freq"() -> (w1876:dbl)
              n1119 = Multiply(x=w1908, y=w1877) -> (x*y=w1907:dbl)
              n1120 = Multiply(x=w1903, y=w1877) -> (x*y=w1905:dbl)
              n1121 = Multiply(x=w1900, y=w1877) -> (x*y=w1902:dbl)
              n1122 = Multiply(x=w1897, y=w1877) -> (x*y=w1899:dbl)
              n1123 = Multiply(x=w1890, y=w1877) -> (x*y=w1894:dbl)
              n1124 = Multiply(x=w1889, y=w1877) -> (x*y=w1892:dbl)
              n1125 = Multiply(x=w1876, y=w1877) -> (x*y=w1878:dbl)
              n1126 = Multiply(x=w1875, y=w1877) -> (x*y=w1879:dbl)
              n1127 = Round To Nearest(number=w1907) -> (nearest integer value=w1906:dbl)
              n1128 = Round To Nearest(number=w1905) -> (nearest integer value=w1904:dbl)
              n1129 = Round To Nearest(number=w1902) -> (nearest integer value=w1901:dbl)
              n1130 = Round To Nearest(number=w1899) -> (nearest integer value=w1898:dbl)
              n1131 = Round To Nearest(number=w1894) -> (nearest integer value=w1893:dbl)
              n1132 = Round To Nearest(number=w1892) -> (nearest integer value=w1891:dbl)
              n1133 = Round To Nearest(number=w1878) -> (nearest integer value=w1881:dbl)
              n1134 = Round To Nearest(number=w1879) -> (nearest integer value=w1880:dbl)
              n1135 = To Unsigned Word Integer(number=w1906) -> (unsigned 16bit integer=w1865:u16)
              n1136 = To Unsigned Word Integer(number=w1904) -> (unsigned 16bit integer=w1867:u16)
              n1137 = To Unsigned Word Integer(number=w1901) -> (unsigned 16bit integer=w1869:u16)
              n1138 = To Unsigned Word Integer(number=w1898) -> (unsigned 16bit integer=w1896:u16)
              n1139 = To Unsigned Word Integer(number=w1893) -> (unsigned 16bit integer=w1888:u16)
              n1140 = To Unsigned Word Integer(number=w1891) -> (unsigned 16bit integer=w1887:u16)
              n1141 = To Unsigned Word Integer(number=w1881) -> (unsigned 16bit integer=w1872:u16)
              n1142 = To Unsigned Word Integer(number=w1880) -> (unsigned 16bit integer=w1871:u16)
              n1143 = local read "Laser_duration_l2"() -> (w1895:u16)
              n1144 = Replace Array Subset(array=w1916, new element #1=w1865, index #1=w1866, new element #2=w1867, index #2=w1868, new element #3=w1869, index #3=w1870, new element #4=w1896, index #4=w1885, new element #5=w1888, index #5=w1884, new element #6=w1887, index #6=w1883, new element #7=w1895, index #7=w1882, new element #8=w1872, index #8=w1874, new element #9=w1871, index #9=w1873) -> (w1915:u16[])
            }
            frame "saveSettings_LC_ENL_l1" {
              # "Selection First"
              # "Count"
              # "Tdelay"
              # "Probability"
              # "OnOff"
              # "Block"
              # "delayOpt"
              # "Count"
              # "Tdelay"
              # "Probability"
              # "OnOff"
              # "Block"
              # "ENL1 All"
              # "delayOpt"
              # "Count"
              # "Tdelay"
              # "Probability"
              # "OnOff"
              # "Block"
              # "ENL1 First"
              n1145 = local read "LC_ENL1_delayOpt_Switch_l1"() -> (w1954:bool)
              n1146 = call "myRIO_BRig_RT_dataLC_ENL1_Block_NS_l1.vi"() -> ("output_ENL1_All_Block"=w1951:i32)  [unwired: 11 in]
              n1147 = call "myRIO_BRig_RT_dataLC_ENL1_OnOff_NS_l1.vi"() -> ("output_ENL1_OnOff_NS_l1"=w1941:i32)  [unwired: 11 in]
              n1148 = call "myRIO_BRig_RT_dataLC_ENL1_Probability_NS_l1.vi"() -> ("output_ENL1_Probability_NS_l1"=w1940:i32)  [unwired: 11 in]
              n1149 = call "myRIO_BRig_RT_dataLC_ENL1_Tdelay_NS_l1.vi"() -> ("output_ENL1_Tdelay_NS_l1"=w1939:i32)  [unwired: 11 in]
              n1150 = call "myRIO_BRig_RT_dataLC_ENL1_Count_NS_l1.vi"() -> ("output_ENL1_Count_NS_l1"=w1938:i32)  [unwired: 11 in]
              n1151 = call "myRIO_BRig_RT_dataLC_ENL1_delayOpt_NS_l1.vi"() -> ("output_ENL1_delayOpt_NS_l1"=w1937:i32)  [unwired: 11 in]
              n1152 = call "myRIO_BRig_RT_dataLC_ENL1_Block_Switch_l1.vi"() -> ("output_ENL1_Block_Switch_l1"=w1973:i32)  [unwired: 11 in]
              n1153 = call "myRIO_BRig_RT_dataLC_ENL1_OnOff_Switch_l1.vi"() -> ("output_ENL1_OnOff_Switch_l1"=w1971:i32)  [unwired: 11 in]
              n1154 = call "myRIO_BRig_RT_dataLC_ENL1_Probability_Switch_l1.vi"() -> ("output_ENL1_Probability_Switch_l1"=w1967:i32)  [unwired: 11 in]
              n1155 = call "myRIO_BRig_RT_dataLC_ENL1_Tdelay_Switch_l1.vi"() -> ("output_ENL1_Tdelay_Switch_l1"=w1965:i32)  [unwired: 11 in]
              n1156 = call "myRIO_BRig_RT_dataLC_ENL1_Count_Switch_l1.vi"() -> ("output_ENL1_Count_Switch_l1"=w1963:i32)  [unwired: 11 in]
              n1157 = call "myRIO_BRig_RT_dataLC_ENL1_delayOpt_Switch_l1.vi"() -> ("output_ENL1_delayOpt_Switch_l1"=w1953:i32)  [unwired: 11 in]
              n1158 = local read "LC_ENL1_Count_Switch_l1"() -> (w1962:u16)
              n1159 = local read "LC_ENL1_Probability_Switch_l1"() -> (w1966:u16)
              n1160 = local read "LC_ENL1_Block_Switch_l1"() -> (w1972:u16)
              n1161 = local read "LC_ENL1_Tdelay_Switch_l1"() -> (w1964:u16)
              n1162 = local read "LC_ENL1_OnOff_Switch_l1"() -> (w1970:bool)
              n1163 = call "myRIO_BRig_RT_dataLC_Selection_Block_Switch_l1.vi"() -> ("output_Selection_Block_Switch_l1"=w1935:i32)  [unwired: 11 in]
              n1164 = call "myRIO_BRig_RT_dataLC_Selection_OnOff_Switch_l1.vi"() -> ("output_Selection_OnOff_Switch_l1"=w1934:i32)  [unwired: 11 in]
              n1165 = call "myRIO_BRig_RT_dataLC_Selection_Probability_Switch_l1.vi"() -> ("output_Selection_Probability_Switch_l1"=w1933:i32)  [unwired: 11 in]
              n1166 = call "myRIO_BRig_RT_dataLC_Selection_Tdelay_Switch_l1.vi"() -> ("output_Selection_Tdelay_Switch_l1"=w1932:i32)  [unwired: 11 in]
              n1167 = call "myRIO_BRig_RT_dataLC_Selection_Count_Switch_l1.vi"() -> ("output_Selection_Count_Switch_l1"=w1931:i32)  [unwired: 11 in]
              n1168 = local read "LC_ENL1_OnOff_NS_l1"() -> (w1947:bool)
              n1169 = local read "LC_ENL1_Probability_NS_l1"() -> (w1945:u16)
              n1170 = local read "LC_ENL1_delayOpt_NS_l1"() -> (w1943:bool)
              n1171 = local read "LC_Sel_Probability_Switch_l1"() -> (w1926:u16)
              n1172 = local read "LC_ENL1_Tdelay_NS_l1"() -> (w1936:u16)
              n1173 = local read "LC_ENL1_Block_NS_l1"() -> (w1948:u16)
              n1174 = local read "LC_ENL1_Count_NS_l1"() -> (w1944:u16)
              n1175 = local read "LC_Sel_Tdelay_Switch_l1"() -> (w1925:u16)
              n1176 = local read "LC_Sel_OnOff_Switch_l1"() -> (w1929:bool)
              n1177 = local read "LC_Sel_Count_Switch_l1"() -> (w1924:u16)
              n1178 = local read "LC_Sel_Block_Switch_l1"() -> (w1928:u16)
              n1179 = Boolean To (0,1)(Boolean=w1954) -> (0, 1=w1955:i16)
              n1180 = Boolean To (0,1)(Boolean=w1970) -> (0, 1=w1969:i16)
              n1181 = Boolean To (0,1)(Boolean=w1947) -> (0, 1=w1950:i16)
              n1182 = To Unsigned Word Integer(number=w1955) -> (unsigned 16bit integer=w1952:u16)
              n1183 = To Unsigned Word Integer(number=w1969) -> (unsigned 16bit integer=w1968:u16)
              n1184 = Boolean To (0,1)(Boolean=w1943) -> (0, 1=w1949:i16)
              n1185 = To Unsigned Word Integer(number=w1950) -> (unsigned 16bit integer=w1946:u16)
              n1186 = Boolean To (0,1)(Boolean=w1929) -> (0, 1=w1930:i16)
              n1187 = To Unsigned Word Integer(number=w1949) -> (unsigned 16bit integer=w1942:u16)
              n1188 = To Unsigned Word Integer(number=w1930) -> (unsigned 16bit integer=w1927:u16)
              n1189 = Replace Array Subset(array=w1974, new element #1=w1972, index #1=w1973, new element #2=w1968, index #2=w1971, new element #3=w1966, index #3=w1967, new element #4=w1964, index #4=w1965, new element #5=w1962, index #5=w1963, new element #6=w1952, index #6=w1953, new element #7=w1948, index #7=w1951, new element #8=w1946, index #8=w1941, new element #9=w1945, index #9=w1940, new element #10=w1936, index #10=w1939, new element #11=w1944, index #11=w1938, new element #12=w1942, index #12=w1937, new element #13=w1928, index #13=w1935, new element #14=w1927, index #14=w1934, new element #15=w1926, index #15=w1933, new element #16=w1925, index #16=w1932, new element #17=w1924, index #17=w1931) -> (w1975:u16[])
            }
            frame "saveSettings_LC_ENL_l2" {
              # "Selection First"
              # "Count"
              # "Tdelay"
              # "Probability"
              # "OnOff"
              # "Block"
              # "delayOpt"
              # "Count"
              # "Tdelay"
              # "Probability"
              # "OnOff"
              # "Block"
              # "ENL1 All"
              # "delayOpt"
              # "Count"
              # "Tdelay"
              # "Probability"
              # "OnOff"
              # "Block"
              # "ENL1 First"
              n1190 = call "myRIO_BRig_RT_dataLC_ENL1_Block_Switch_l2.vi"() -> ("output_ENL1_Block_Switch_l2"=w1994:i32)  [unwired: 11 in]
              n1191 = call "myRIO_BRig_RT_dataLC_ENL1_OnOff_Switch_l2.vi"() -> ("output_ENL1_OnOff_Switch_l2"=w1995:i32)  [unwired: 11 in]
              n1192 = call "myRIO_BRig_RT_dataLC_ENL1_Probability_Switch_l2.vi"() -> ("output_ENL1_Probability_Switch_l2"=w1996:i32)  [unwired: 11 in]
              n1193 = call "myRIO_BRig_RT_dataLC_ENL1_Tdelay_Switch_l2.vi"() -> ("output_ENL1_Tdelay_Switch_l2"=w1997:i32)  [unwired: 11 in]
              n1194 = call "myRIO_BRig_RT_dataLC_ENL1_Count_Switch_l2.vi"() -> ("output_ENL1_Count_Switch_l2"=w1998:i32)  [unwired: 11 in]
              n1195 = call "myRIO_BRig_RT_dataLC_ENL1_delayOpt_Switch_l2.vi"() -> ("output_ENL1_delayOpt_Switch_l2"=w1999:i32)  [unwired: 11 in]
              n1196 = local read "LC_ENL1_delayOpt_Switch_l2"() -> (w2019:bool)
              n1197 = call "myRIO_BRig_RT_dataLC_ENL1_Block_NS_l2.vi"() -> ("output_ENL1_Block_NS_l2"=w1988:i32)  [unwired: 11 in]
              n1198 = call "myRIO_BRig_RT_dataLC_ENL1_OnOff_NS_l2.vi"() -> ("output_ENL1_OnOff_NS_l2"=w1989:i32)  [unwired: 11 in]
              n1199 = call "myRIO_BRig_RT_dataLC_ENL1_Probability_NS_l2.vi"() -> ("output_ENL1_Probability_NS_l2"=w1990:i32)  [unwired: 11 in]
              n1200 = call "myRIO_BRig_RT_dataLC_ENL1_Tdelay_NS_l2.vi"() -> ("output_ENL1_Tdelay_NS_l2"=w1991:i32)  [unwired: 11 in]
              n1201 = call "myRIO_BRig_RT_dataLC_ENL1_Count_NS_l2.vi"() -> ("output_ENL1_Count_NS_l2"=w1992:i32)  [unwired: 11 in]
              n1202 = call "myRIO_BRig_RT_dataLC_ENL1_delayOpt_NS_l2.vi"() -> ("output_ENL1_delayOpt_NS_l2"=w1993:i32)  [unwired: 11 in]
              n1203 = local read "LC_ENL1_Count_Switch_l2"() -> (w2027:u16)
              n1204 = local read "LC_ENL1_Probability_Switch_l2"() -> (w2029:u16)
              n1205 = local read "LC_ENL1_Block_Switch_l2"() -> (w2033:u16)
              n1206 = local read "LC_ENL1_Tdelay_Switch_l2"() -> (w2028:u16)
              n1207 = local read "LC_ENL1_OnOff_Switch_l2"() -> (w2032:bool)
              n1208 = call "myRIO_BRig_RT_dataLC_Selection_Block_Switch_l2.vi"() -> ("output_Selection_Block_Switch_l2"=w1987:i32)  [unwired: 11 in]
              n1209 = call "myRIO_BRig_RT_dataLC_Selection_OnOff_Switch_l2.vi"() -> ("output_Selection_OnOff_Switch_l2"=w1986:i32)  [unwired: 11 in]
              n1210 = call "myRIO_BRig_RT_dataLC_Selection_Probability_Switch_l2.vi"() -> ("output_Selection_Probability_Switch_l1"=w1985:i32)  [unwired: 11 in]
              n1211 = call "myRIO_BRig_RT_dataLC_Selection_Tdelay_Switch_l2.vi"() -> ("output_Selection_Tdelay_Switch_l2"=w1984:i32)  [unwired: 11 in]
              n1212 = call "myRIO_BRig_RT_dataLC_Selection_Count_Switch_l2.vi"() -> ("output_Selection_Count_Switch_l2"=w1983:i32)  [unwired: 11 in]
              n1213 = local read "LC_ENL1_OnOff_NS_l2"() -> (w2014:bool)
              n1214 = local read "LC_ENL1_Probability_NS_l2"() -> (w2012:u16)
              n1215 = local read "LC_ENL1_delayOpt_NS_l2"() -> (w2010:bool)
              n1216 = local read "LC_Sel_Probability_Switch_l2"() -> (w2003:u16)
              n1217 = local read "LC_ENL1_Tdelay_NS_l2"() -> (w2008:u16)
              n1218 = local read "LC_ENL1_Block_NS_l2"() -> (w2015:u16)
              n1219 = local read "LC_ENL1_Count_NS_l2"() -> (w2011:u16)
              n1220 = local read "LC_Sel_Tdelay_Switch_l2"() -> (w2002:u16)
              n1221 = local read "LC_Sel_OnOff_Switch_l2"() -> (w2006:bool)
              n1222 = local read "LC_Sel_Count_Switch_l2"() -> (w2001:u16)
              n1223 = local read "LC_Sel_Block_Switch_l2"() -> (w2005:u16)
              n1224 = Boolean To (0,1)(Boolean=w2019) -> (0, 1=w2020:i16)
              n1225 = Boolean To (0,1)(Boolean=w2032) -> (0, 1=w2031:i16)
              n1226 = Boolean To (0,1)(Boolean=w2014) -> (0, 1=w2017:i16)
              n1227 = To Unsigned Word Integer(number=w2020) -> (unsigned 16bit integer=w2018:u16)
              n1228 = To Unsigned Word Integer(number=w2031) -> (unsigned 16bit integer=w2030:u16)
              n1229 = Boolean To (0,1)(Boolean=w2010) -> (0, 1=w2016:i16)
              n1230 = To Unsigned Word Integer(number=w2017) -> (unsigned 16bit integer=w2013:u16)
              n1231 = Boolean To (0,1)(Boolean=w2006) -> (0, 1=w2007:i16)
              n1232 = To Unsigned Word Integer(number=w2016) -> (unsigned 16bit integer=w2009:u16)
              n1233 = To Unsigned Word Integer(number=w2007) -> (unsigned 16bit integer=w2004:u16)
              n1234 = Replace Array Subset(array=w2034, new element #1=w2033, index #1=w1994, new element #2=w2030, index #2=w1995, new element #3=w2029, index #3=w1996, new element #4=w2028, index #4=w1997, new element #5=w2027, index #5=w1998, new element #6=w2018, index #6=w1999, new element #7=w2015, index #7=w1988, new element #8=w2013, index #8=w1989, new element #9=w2012, index #9=w1990, new element #10=w2008, index #10=w1991, new element #11=w2011, index #11=w1992, new element #12=w2009, index #12=w1993, new element #13=w2005, index #13=w1987, new element #14=w2004, index #14=w1986, new element #15=w2003, index #15=w1985, new element #16=w2002, index #16=w1984, new element #17=w2001, index #17=w1983) -> (w2035:u16[])
            }
            frame "saveSettings_LC_Cue_l1" {
              # "Selection All"
              # "Count"
              # "Tdelay"
              # "Probability"
              # "OnOff"
              # "Block"
              # "delayOpt"
              # "Count"
              # "Tdelay"
              # "Probability"
              # "OnOff"
              # "Block"
              # "Cue1 All"
              # "delayOpt"
              # "Count"
              # "Tdelay"
              # "Probability"
              # "OnOff"
              # "Block"
              # "Cue1 First"
              n1235 = call "myRIO_BRig_RT_dataLC_Cue1_delayOpt_Switch_l1.vi"() -> ("output_Cue1_delayOpt_Switch_l1"=w2074:i32)  [unwired: 11 in]
              n1236 = call "myRIO_BRig_RT_dataLC_Cue1_Block_Switch_l1.vi"() -> ("output_Cue1_Block_Switch_l1"=w2093:i32)  [unwired: 11 in]
              n1237 = call "myRIO_BRig_RT_dataLC_Cue1_OnOff_Switch_l1.vi"() -> ("output_Cue1_OnOff_Switch_l1"=w2091:i32)  [unwired: 11 in]
              n1238 = call "myRIO_BRig_RT_dataLC_Cue1_Probability_Switch_l1.vi"() -> ("output_Cue1_Probability_Switch_l1"=w2087:i32)  [unwired: 11 in]
              n1239 = call "myRIO_BRig_RT_dataLC_Cue1_Tdelay_Switch_l1.vi"() -> ("output_Cue1_Tdelay_Switch_l1"=w2085:i32)  [unwired: 11 in]
              n1240 = call "myRIO_BRig_RT_dataLC_Cue1_Count_Switch_l1.vi"() -> ("output_Cue1_Count_Switch_l1"=w2083:i32)  [unwired: 11 in]
              n1241 = local read "LC_Cue1_delayOpt_Switch_l1"() -> (w2073:bool)
              n1242 = call "myRIO_BRig_RT_dataLC_Cue1_Block_NS_l1.vi"() -> ("output_Cue1_Block_NS_l1"=w2071:i32)  [unwired: 11 in]
              n1243 = call "myRIO_BRig_RT_dataLC_Cue1_OnOff_NS_l1.vi"() -> ("output_Cue1_OnOff_NS_l1"=w2070:i32)  [unwired: 11 in]
              n1244 = call "myRIO_BRig_RT_dataLC_Cue1_Probability_NS_l1.vi"() -> ("output_Cue1_l1_All_Probability"=w2069:i32)  [unwired: 11 in]
              n1245 = call "myRIO_BRig_RT_dataLC_Cue1_Tdelay_NS_l1.vi"() -> ("output_Cue1_Tdelay_NS_l1"=w2068:i32)  [unwired: 11 in]
              n1246 = call "myRIO_BRig_RT_dataLC_Cue1_Count_NS_l1.vi"() -> ("output_Cue1_Count_NS_l1"=w2067:i32)  [unwired: 11 in]
              n1247 = call "myRIO_BRig_RT_dataLC_Cue1_delayOpt_NS_l1.vi"() -> ("output_Cue1_delayOpt_NS_l1"=w2066:i32)  [unwired: 11 in]
              n1248 = local read "LC_Cue1_Count_Switch_l1"() -> (w2082:u16)
              n1249 = local read "LC_Cue1_Probability_Switch_l1"() -> (w2086:u16)
              n1250 = local read "LC_Cue1_Block_Switch_l1"() -> (w2092:u16)
              n1251 = local read "LC_Cue1_Tdelay_Switch_l1"() -> (w2084:u16)
              n1252 = local read "LC_Cue1_OnOff_Switch_l1"() -> (w2090:bool)
              n1253 = local read "LC_Cue1_OnOff_NS_l1"() -> (w2062:bool)
              n1254 = call "myRIO_BRig_RT_dataLC_Selection_Block_NS_l1.vi"() -> ("output_Selection_Block_NS_l1"=w2055:i32)  [unwired: 11 in]
              n1255 = call "myRIO_BRig_RT_dataLC_Selection_OnOff_NS_l1.vi"() -> ("output_Selection_OnOff_NS_l1"=w2054:i32)  [unwired: 11 in]
              n1256 = call "myRIO_BRig_RT_dataLC_Selection_Probability_NS_l1.vi"() -> ("output_Selection_Probability_NS_l1"=w2053:i32)  [unwired: 11 in]
              n1257 = call "myRIO_BRig_RT_dataLC_Selection_Tdelay_NS_l1.vi"() -> ("output_Selection_Tdelay_NS_l1"=w2052:i32)  [unwired: 11 in]
              n1258 = call "myRIO_BRig_RT_dataLC_Selection_Count_NS_l1.vi"() -> ("output_Selection_Count_NS_l1"=w2045:i32)  [unwired: 11 in]
              n1259 = local read "LC_Cue1_delayOpt_NS_l1"() -> (w2063:bool)
              n1260 = local read "LC_Cue1_Probability_NS_l1"() -> (w2059:u16)
              n1261 = local read "LC_Cue1_Tdelay_NS_l1"() -> (w2058:u16)
              n1262 = local read "LC_Cue1_Count_NS_l1"() -> (w2057:u16)
              n1263 = local read "LC_Cue1_Block_NS_l1"() -> (w2061:u16)
              n1264 = local read "LC_Sel_Probability_NS_l1"() -> (w2047:u16)
              n1265 = local read "LC_Sel_Tdelay_NS_l1"() -> (w2046:u16)
              n1266 = local read "LC_Sel_OnOff_NS_l1"() -> (w2049:bool)
              n1267 = local read "LC_Sel_Count_NS_l1"() -> (w2044:u16)
              n1268 = local read "LC_Sel_Block_NS_l1"() -> (w2051:u16)
              n1269 = Boolean To (0,1)(Boolean=w2073) -> (0, 1=w2075:i16)
              n1270 = Boolean To (0,1)(Boolean=w2090) -> (0, 1=w2089:i16)
              n1271 = Boolean To (0,1)(Boolean=w2062) -> (0, 1=w2065:i16)
              n1272 = To Unsigned Word Integer(number=w2075) -> (unsigned 16bit integer=w2072:u16)
              n1273 = To Unsigned Word Integer(number=w2089) -> (unsigned 16bit integer=w2088:u16)
              n1274 = To Unsigned Word Integer(number=w2065) -> (unsigned 16bit integer=w2060:u16)
              n1275 = Boolean To (0,1)(Boolean=w2063) -> (0, 1=w2064:i16)
              n1276 = Boolean To (0,1)(Boolean=w2049) -> (0, 1=w2050:i16)
              n1277 = To Unsigned Word Integer(number=w2064) -> (unsigned 16bit integer=w2056:u16)
              n1278 = To Unsigned Word Integer(number=w2050) -> (unsigned 16bit integer=w2048:u16)
              n1279 = Replace Array Subset(array=w2094, new element #1=w2092, index #1=w2093, new element #2=w2088, index #2=w2091, new element #3=w2086, index #3=w2087, new element #4=w2084, index #4=w2085, new element #5=w2082, index #5=w2083, new element #6=w2072, index #6=w2074, new element #7=w2061, index #7=w2071, new element #8=w2060, index #8=w2070, new element #9=w2059, index #9=w2069, new element #10=w2058, index #10=w2068, new element #11=w2057, index #11=w2067, new element #12=w2056, index #12=w2066, new element #13=w2051, index #13=w2055, new element #14=w2048, index #14=w2054, new element #15=w2047, index #15=w2053, new element #16=w2046, index #16=w2052, new element #17=w2044, index #17=w2045) -> (w2095:u16[])
            }
            frame "saveSettings_LC_Cue_l2" {
              # "Selection All"
              # "Count"
              # "Tdelay"
              # "Probability"
              # "OnOff"
              # "Block"
              # "delayOpt"
              # "Count"
              # "Tdelay"
              # "Probability"
              # "OnOff"
              # "Block"
              # "Cue1 All"
              # "delayOpt"
              # "Count"
              # "Tdelay"
              # "Probability"
              # "OnOff"
              # "Block"
              # "Cue1 First"
              n1280 = call "myRIO_BRig_RT_dataLC_Cue1_delayOpt_Switch_l2.vi"() -> ("output_Cue1_delayOpt_Switch_l2"=w2134:i32)  [unwired: 11 in]
              n1281 = call "myRIO_BRig_RT_dataLC_Cue1_Block_Switch_l2.vi"() -> ("output_Cue1_Block_Switch_l2"=w2153:i32)  [unwired: 11 in]
              n1282 = call "myRIO_BRig_RT_dataLC_Cue1_OnOff_Switch_l2.vi"() -> ("output_Cue1_OnOff_Switch_l2"=w2151:i32)  [unwired: 11 in]
              n1283 = call "myRIO_BRig_RT_dataLC_Cue1_Probability_Switch_l2.vi"() -> ("output_Cue1_l2_First_Probability"=w2147:i32)  [unwired: 11 in]
              n1284 = call "myRIO_BRig_RT_dataLC_Cue1_Tdelay_Switch_l2.vi"() -> ("output_Cue1_Tdelay_Switch_l2"=w2145:i32)  [unwired: 11 in]
              n1285 = call "myRIO_BRig_RT_dataLC_Cue1_Count_Switch_l2.vi"() -> ("output_Cue1_Count_Switch_l2"=w2143:i32)  [unwired: 11 in]
              n1286 = local read "LC_Cue1_delayOpt_Switch_l2"() -> (w2133:bool)
              n1287 = call "myRIO_BRig_RT_dataLC_Cue1_Block_NS_l2.vi"() -> ("output_Cue1_Block_NS_l2"=w2131:i32)  [unwired: 11 in]
              n1288 = call "myRIO_BRig_RT_dataLC_Cue1_OnOff_NS_l2.vi"() -> ("output_Cue1_OnOff_NS_l2"=w2130:i32)  [unwired: 11 in]
              n1289 = call "myRIO_BRig_RT_dataLC_Cue1_Probability_NS_l2.vi"() -> ("output_Cue1_l2_All_Probability"=w2129:i32)  [unwired: 11 in]
              n1290 = call "myRIO_BRig_RT_dataLC_Cue1_Tdelay_NS_l2.vi"() -> ("output_Cue1_Tdelay_NS_l2"=w2128:i32)  [unwired: 11 in]
              n1291 = call "myRIO_BRig_RT_dataLC_Cue1_Count_NS_l2.vi"() -> ("output_Cue1_Count_NS_l2"=w2127:i32)  [unwired: 11 in]
              n1292 = call "myRIO_BRig_RT_dataLC_Cue1_delayOpt_NS_l2.vi"() -> ("output_Cue1_delayOpt_NS_l2"=w2126:i32)  [unwired: 11 in]
              n1293 = local read "LC_Cue1_Count_Switch_l2"() -> (w2142:u16)
              n1294 = local read "LC_Cue1_Probability_Switch_l2"() -> (w2146:u16)
              n1295 = local read "LC_Cue1_Block_Switch_l2"() -> (w2152:u16)
              n1296 = local read "LC_Cue1_Tdelay_Switch_l2"() -> (w2144:u16)
              n1297 = local read "LC_Cue1_OnOff_Switch_l2"() -> (w2150:bool)
              n1298 = local read "LC_Cue1_OnOff_NS_l2"() -> (w2122:bool)
              n1299 = call "myRIO_BRig_RT_dataLC_Selection_Block_NS_l2.vi"() -> ("output_Selection_Block_NS_l2"=w2107:i32)  [unwired: 11 in]
              n1300 = call "myRIO_BRig_RT_dataLC_Selection_OnOff_NS_l2.vi"() -> ("output_Selection_OnOff_NS_l2"=w2106:i32)  [unwired: 11 in]
              n1301 = call "myRIO_BRig_RT_dataLC_Selection_Probability_NS_l2.vi"() -> ("output_Selection_Probability_NS_l2"=w2105:i32)  [unwired: 11 in]
              n1302 = call "myRIO_BRig_RT_dataLC_Selection_Tdelay_NS_l2.vi"() -> ("output_Selection_Tdelay_NS_l2"=w2104:i32)  [unwired: 11 in]
              n1303 = call "myRIO_BRig_RT_dataLC_Selection_Count_NS_l2.vi"() -> ("output_Selection_Count_NS_l2"=w2103:i32)  [unwired: 11 in]
              n1304 = local read "LC_Cue1_delayOpt_NS_l2"() -> (w2123:bool)
              n1305 = local read "LC_Cue1_Probability_NS_l2"() -> (w2119:u16)
              n1306 = local read "LC_Cue1_Tdelay_NS_l2"() -> (w2118:u16)
              n1307 = local read "LC_Cue1_Count_NS_l2"() -> (w2117:u16)
              n1308 = local read "LC_Cue1_Block_NS_l2"() -> (w2121:u16)
              n1309 = local read "LC_Sel_Probability_NS_l2"() -> (w2111:u16)
              n1310 = local read "LC_Sel_Tdelay_NS_l2"() -> (w2110:u16)
              n1311 = local read "LC_Sel_OnOff_NS_l2"() -> (w2113:bool)
              n1312 = local read "LC_Sel_Count_NS_l2"() -> (w2109:u16)
              n1313 = local read "LC_Sel_Block_NS_l2"() -> (w2115:u16)
              n1314 = Boolean To (0,1)(Boolean=w2133) -> (0, 1=w2135:i16)
              n1315 = Boolean To (0,1)(Boolean=w2150) -> (0, 1=w2149:i16)
              n1316 = Boolean To (0,1)(Boolean=w2122) -> (0, 1=w2125:i16)
              n1317 = To Unsigned Word Integer(number=w2135) -> (unsigned 16bit integer=w2132:u16)
              n1318 = To Unsigned Word Integer(number=w2149) -> (unsigned 16bit integer=w2148:u16)
              n1319 = To Unsigned Word Integer(number=w2125) -> (unsigned 16bit integer=w2120:u16)
              n1320 = Boolean To (0,1)(Boolean=w2123) -> (0, 1=w2124:i16)
              n1321 = Boolean To (0,1)(Boolean=w2113) -> (0, 1=w2114:i16)
              n1322 = To Unsigned Word Integer(number=w2124) -> (unsigned 16bit integer=w2116:u16)
              n1323 = To Unsigned Word Integer(number=w2114) -> (unsigned 16bit integer=w2112:u16)
              n1324 = Replace Array Subset(array=w2154, new element #1=w2152, index #1=w2153, new element #2=w2148, index #2=w2151, new element #3=w2146, index #3=w2147, new element #4=w2144, index #4=w2145, new element #5=w2142, index #5=w2143, new element #6=w2132, index #6=w2134, new element #7=w2121, index #7=w2131, new element #8=w2120, index #8=w2130, new element #9=w2119, index #9=w2129, new element #10=w2118, index #10=w2128, new element #11=w2117, index #11=w2127, new element #12=w2116, index #12=w2126, new element #13=w2115, index #13=w2107, new element #14=w2112, index #14=w2106, new element #15=w2111, index #15=w2105, new element #16=w2110, index #16=w2104, new element #17=w2109, index #17=w2103) -> (w2155:u16[])
            }
            frame "saveSettings6_LC_l1_Other" {
              # "Trial"
              # "Tdelay"
              # "Probability"
              # "OnOff"
              # "Block"
              # "Wrong"
              # "Trial"
              # "Tdelay"
              # "Probability"
              # "OnOff"
              # "Block"
              # "Reward"
              n1325 = call "myRIO_BRig_RT_dataLC_Wrong_Block_l1.vi"() -> ("output_Wrong_Block_l1"=w2180:i32)  [unwired: 11 in]
              n1326 = call "myRIO_BRig_RT_dataLC_Wrong_OnOff_l1.vi"() -> ("output_Wrong_OnOff_l1"=w2179:i32)  [unwired: 11 in]
              n1327 = call "myRIO_BRig_RT_dataLC_Wrong_Probability_l1.vi"() -> ("output_Wrong_Probability_l1"=w2178:i32)  [unwired: 11 in]
              n1328 = call "myRIO_BRig_RT_dataLC_Wrong_Tdelay_l1.vi"() -> ("output_Wrong_Tdelay_l1"=w2177:i32)  [unwired: 11 in]
              n1329 = call "myRIO_BRig_RT_dataLC_Wrong_Trial_l1.vi"() -> ("output_Wrong_Trial_l1"=w2176:i32)  [unwired: 11 in]
              n1330 = call "myRIO_BRig_RT_dataLC_Reward_Block_l1.vi"() -> ("output_Reward_Block_l1"=w2192:i32)  [unwired: 11 in]
              n1331 = call "myRIO_BRig_RT_dataLC_Reward_OnOff_l1.vi"() -> ("output_Reward_OnOff_l1"=w2190:i32)  [unwired: 11 in]
              n1332 = call "myRIO_BRig_RT_dataLC_Reward_Probability_l1.vi"() -> ("output_Reward_Probability_l1"=w2186:i32)  [unwired: 11 in]
              n1333 = call "myRIO_BRig_RT_dataLC_Reward_Tdelay_l1.vi"() -> ("output_Reward_Tdelay_l1"=w2184:i32)  [unwired: 11 in]
              n1334 = call "myRIO_BRig_RT_dataLC_Reward_Trial_l1.vi"() -> ("output_Reward_Trial_l1"=w2182:i32)  [unwired: 11 in]
              n1335 = local read "LC_Wrong_OnOff_l1"() -> (w2174:bool)
              n1336 = local read "LC_Wrong_Probability_l1"() -> (w2171:u16)
              n1337 = local read "LC_Wrong_Block_l1"() -> (w2173:u16)
              n1338 = local read "LC_Wrong_Tdelay_l1"() -> (w2170:u16)
              n1339 = local read "LC_Wrong_Trial_l1"() -> (w2169:u16)
              n1340 = local read "LC_Reward_Probability_l1"() -> (w2185:u16)
              n1341 = local read "LC_Reward_Block_l1"() -> (w2191:u16)
              n1342 = local read "LC_Reward_Tdelay_l1"() -> (w2183:u16)
              n1343 = local read "LC_Reward_OnOff_l1"() -> (w2189:bool)
              n1344 = local read "LC_Reward_Trial_l1"() -> (w2181:u16)
              n1345 = Boolean To (0,1)(Boolean=w2174) -> (0, 1=w2175:i16)
              n1346 = Boolean To (0,1)(Boolean=w2189) -> (0, 1=w2188:i16)
              n1347 = To Unsigned Word Integer(number=w2175) -> (unsigned 16bit integer=w2172:u16)
              n1348 = To Unsigned Word Integer(number=w2188) -> (unsigned 16bit integer=w2187:u16)
              n1349 = Replace Array Subset(array=w2193, new element #1=w2191, index #1=w2192, new element #2=w2187, index #2=w2190, new element #3=w2185, index #3=w2186, new element #4=w2183, index #4=w2184, new element #5=w2181, index #5=w2182, new element #6=w2173, index #6=w2180, new element #7=w2172, index #7=w2179, new element #8=w2171, index #8=w2178, new element #9=w2170, index #9=w2177, new element #10=w2169, index #10=w2176) -> (w2194:u16[])
            }
            frame "SaveSettings6_LC_l2_Other" {
              # "Trial"
              # "Tdelay"
              # "Probability"
              # "OnOff"
              # "Block"
              # "Wrong"
              # "Trial"
              # "Tdelay"
              # "Probability"
              # "OnOff"
              # "Block"
              # "Reward"
              n1350 = call "myRIO_BRig_RT_dataLC_Wrong_Block_l2.vi"() -> ("output_Wrong_Block_l2"=w2203:i32)  [unwired: 11 in]
              n1351 = call "myRIO_BRig_RT_dataLC_Wrong_OnOff_l2.vi"() -> ("output_Wrong_OnOff_l2"=w2204:i32)  [unwired: 11 in]
              n1352 = call "myRIO_BRig_RT_dataLC_Wrong_Probability_l2.vi"() -> ("output_Wrong_Probability_l2"=w2205:i32)  [unwired: 11 in]
              n1353 = call "myRIO_BRig_RT_dataLC_Wrong_Tdelay_l2.vi"() -> ("output_Wrong_Tdelay_l2"=w2206:i32)  [unwired: 11 in]
              n1354 = call "myRIO_BRig_RT_dataLC_Wrong_Trial_l2.vi"() -> ("output_Wrong_Trial_l2"=w2207:i32)  [unwired: 11 in]
              n1355 = call "myRIO_BRig_RT_dataLC_Reward_Block_l2.vi"() -> ("output_Reward_Block_l2"=w2208:i32)  [unwired: 11 in]
              n1356 = call "myRIO_BRig_RT_dataLC_Reward_OnOff_l2.vi"() -> ("output_Reward_OnOff_l2"=w2209:i32)  [unwired: 11 in]
              n1357 = call "myRIO_BRig_RT_dataLC_Reward_Probability_l2.vi"() -> ("output_Reward_Probability_l2"=w2210:i32)  [unwired: 11 in]
              n1358 = call "myRIO_BRig_RT_dataLC_Reward_Tdelay_l2.vi"() -> ("output_Reward_Tdelay_l2"=w2211:i32)  [unwired: 11 in]
              n1359 = call "myRIO_BRig_RT_dataLC_Reward_Trial_l2.vi"() -> ("output_Reward_Trial_l2"=w2212:i32)  [unwired: 11 in]
              n1360 = local read "LC_Wrong_OnOff_l2"() -> (w2224:bool)
              n1361 = local read "LC_Wrong_Probability_l2"() -> (w2221:u16)
              n1362 = local read "LC_Wrong_Block_l2"() -> (w2223:u16)
              n1363 = local read "LC_Wrong_Tdelay_l2"() -> (w2220:u16)
              n1364 = local read "LC_Wrong_Trial_l2"() -> (w2219:u16)
              n1365 = local read "LC_Reward_Probability_l2"() -> (w2228:u16)
              n1366 = local read "LC_Reward_Block_l2"() -> (w2232:u16)
              n1367 = local read "LC_Reward_Tdelay_l2"() -> (w2227:u16)
              n1368 = local read "LC_Reward_OnOff_l2"() -> (w2231:bool)
              n1369 = local read "LC_Reward_Trial_l2"() -> (w2226:u16)
              n1370 = Boolean To (0,1)(Boolean=w2224) -> (0, 1=w2225:i16)
              n1371 = Boolean To (0,1)(Boolean=w2231) -> (0, 1=w2230:i16)
              n1372 = To Unsigned Word Integer(number=w2225) -> (unsigned 16bit integer=w2222:u16)
              n1373 = To Unsigned Word Integer(number=w2230) -> (unsigned 16bit integer=w2229:u16)
              n1374 = Replace Array Subset(array=w2233, new element #1=w2232, index #1=w2208, new element #2=w2229, index #2=w2209, new element #3=w2228, index #3=w2210, new element #4=w2227, index #4=w2211, new element #5=w2226, index #5=w2212, new element #6=w2223, index #6=w2203, new element #7=w2222, index #7=w2204, new element #8=w2221, index #8=w2205, new element #9=w2220, index #9=w2206, new element #10=w2219, index #10=w2207) -> (w2234:u16[])
            }
            frame "setSettings_Audio" {
              # "amp_L"
              # "amp_R"
              # "freq_L"
              # "freq_R"
              n1375 = call "myRIO_BRig_RT_dataExp_Audio_amp__L.vi"() -> ("output_Audio_amp__L"=w2262:i32)  [unwired: 11 in]
              n1376 = call "myRIO_BRig_RT_dataExp_Audio_amp__R.vi"() -> ("output_Audio_amp__R"=w2261:i32)  [unwired: 11 in]
              n1377 = call "myRIO_BRig_RT_dataExp_Audio_freq__L.vi"() -> ("output_Audio_freq__L"=w2260:i32)  [unwired: 11 in]
              n1378 = call "myRIO_BRig_RT_dataExp_Audio_freq__R.vi"() -> ("output_Audio_freq__R"=w2259:i32)  [unwired: 11 in]
              n1379 = Index Array(array=w2258, index #1=w2262, index #2=w2261, index #3=w2260, index #4=w2259) -> (element #1=w2247:u16, element #2=w2246:u16, element #3=w2251:u16, element #4=w2250:u16)
              n1380 = To Unsigned Byte Integer(number=w2251) -> (unsigned 8bit integer=w2245:u8)
              n1381 = To Unsigned Byte Integer(number=w2250) -> (unsigned 8bit integer=w2244:u8)
              n1382 = xnode "Read/Write Control"("FPGA VI Reference In"=w2249, "error in"=w2248, "audioAmp_L"=w2247, "audioAmp_R"=w2246, "audioFreq_L_kHz"=w2245, "audioFreq_R_kHz"=w2244) -> ("error out"=w2243:errorcluster)  [unwired: 1 out]
              n1383 = local write "error out"(w2243) -> ()
            }
            frame "setSettings_Laser" {
              w2293 = u32 0 ("laser2_selRew_Ndelay")
              # "tDelay"
              # "Wrong l1"
              # "Reward l1"
              n1384 = call "myRIO_BRig_RT_dataExp_IallReward.vi"() -> ("output_I_allReward"=w2274:i32)  [unwired: 11 in]
              n1385 = local read "Laser_Tpeak_l1"() -> (w2304:dbl)
              n1386 = local read "Laser_Tshutter_l1"() -> (w2302:dbl)
              n1387 = local read "Laser_Freq_l1"() -> (w2303:dbl)
              n1388 = local read "Laser_duration_l1"() -> (w2278:u16)
              n1389 = local read "Laser_Tpeak_l2"() -> (w2300:dbl)
              n1390 = local read "Laser_Tshutter_l2"() -> (w2298:dbl)
              n1391 = local read "Laser_Freq_l2"() -> (w2299:dbl)
              n1392 = local read "Laser_duration_l2"() -> (w2277:u16)
              n1393 = local read "CueLed_Freq"() -> (w2287:dbl)
              n1394 = local read "CueLed_Tpeak"() -> (w2288:dbl)
              n1395 = local read "I_allReward"() -> (w2273:bool)
              n1396 = call "myRIO_BRig_RT_dataLC_Reward_Tdelay_l1.vi"() -> ("output_Reward_Tdelay_l1"=w2316:i32)  [unwired: 11 in]
              n1397 = call "myRIO_BRig_RT_dataLC_Wrong_Tdelay_l1.vi"() -> ("output_Wrong_Tdelay_l1"=w2317:i32)  [unwired: 11 in]
              n1398 = local read "FPGA_count2ms"() -> (w2289:dbl)
              n1399 = Index Array(array=w2284, index #1=w2316, index #2=w2317) -> (element #1=w2315:u16, element #2=w2314:u16)
              n1400 = To Double Precision Float(number=w2315) -> (double precision float=w2311:dbl)
              n1401 = To Double Precision Float(number=w2314) -> (double precision float=w2308:dbl)
              n1402 = Boolean To (0,1)(Boolean=w2273) -> (0, 1=w2272:i16)
              n1403 = To Unsigned Word Integer(number=w2272) -> (unsigned 16bit integer=w2271:u16)
              n1404 = Replace Array Subset(array=w2276, new element=w2271, index=w2274) -> (w2275:u16[])
              n1405 = To Unsigned Word Integer(number=w2289) -> (unsigned 16bit integer=w2305:u16)
              n1406 = call "myRIO_BRig_RT__calc_laser_FPGA_N.vi"("input_FPGA_ms2count"=w2289, "input_Tpeak"=w2304, "input_Freq"=w2303, "input_Tshutter"=w2302, "input_duration"=w2278) -> ("output_laser_Npeak"=w2292:u32, "output_laser_Nvalley"=w2291:u32, "output_laser_Nshutter"=w2290:u32, "output_laser_Nduration"=w2301:u32, "output_laser_Tduration"=w2282:u16)  [unwired: 6 in]
              n1407 = Multiply(x=w2289, y=w2311) -> (x*y=w2312:dbl)
              n1408 = Multiply(x=w2289, y=w2308) -> (x*y=w2309:dbl)
              n1409 = call "myRIO_BRig_RT__calc_laser_FPGA_N__CueLed.vi"("input_FPGA_ms2count"=w2289, "input_Tpeak"=w2288, "input_Freq"=w2287) -> ("output_laser_Npeak"=w2286:u32, "output_laser_Nvalley"=w2285:u32)  [unwired: 11 in]
              n1410 = call "myRIO_BRig_RT__calc_laser_FPGA_N.vi"("input_FPGA_ms2count"=w2289, "input_Tpeak"=w2300, "input_Freq"=w2299, "input_Tshutter"=w2298, "input_duration"=w2277) -> ("output_laser_Npeak"=w2297:u32, "output_laser_Nvalley"=w2296:u32, "output_laser_Nshutter"=w2295:u32, "output_laser_Nduration"=w2294:u32, "output_laser_Tduration"=w2281:u16)  [unwired: 6 in]
              n1411 = Round Toward +Infinity(x=w2312) -> (ceil(x): smallest int >= x=w2313:dbl)
              n1412 = Round Toward +Infinity(x=w2309) -> (ceil(x): smallest int >= x=w2310:dbl)
              n1413 = To Unsigned Long Integer(number=w2313) -> (unsigned 32bit integer=w2307:u32)
              n1414 = To Unsigned Long Integer(number=w2310) -> (unsigned 32bit integer=w2306:u32)
              n1415 = xnode "Read/Write Control"("FPGA VI Reference In"=w2318, "error in"=w2319, "I_allReward"=w2273, "LC_nPeak_l1"=w2292, "LC_nValley_l1"=w2291, "LC_nShutter_l1"=w2290, "LR_reward_nDelay_l1"=w2307, "LR_wrong_nDelay_l1"=w2306, "LR_reward_nTotal_l1"=w2301, "LR_wrong_nTotal_l1"=w2301, "k1__counter_per_ms"=w2305, "LC_nPeak_l2"=w2297, "LC_nValley_l2"=w2296, "LC_nShutter_l2"=w2295, "LR_reward_nDelay_l2"=w2293, "LR_wrong_nDelay_l2"=w2293, "LR_reward_nTotal_l2"=w2294, "LR_wrong_nTotal_l2"=w2294, "CueLed_nPeak"=w2286, "CueLed_nValley"=w2285) -> ("error out"=→"error out":errorcluster)  [unwired: 1 out]
              n1416 = call "myRIO_BRig_RT_dataCurrent_laser1_pulse_duration.vi"() -> ("output_laser1_pulse_duration"=w2280:i32)  [unwired: 11 in]
              n1417 = call "myRIO_BRig_RT_dataCurrent_laser2_pulse_duration.vi"() -> ("output_laser2_pulse_duration"=w2279:i32)  [unwired: 11 in]
              n1418 = Replace Array Subset(array=w2284, new element #1=w2282, index #1=w2280, new element #2=w2281, index #2=w2279) -> (w2283:u16[])
            }
            frame "initBlock" {
              n1419 = local write "nRewards_cur"(u16 0 ("nRewards_cur")) -> ()
              n1420 = call "myRIO_Brig_RT__Case_Exp_State_initBlock__v2.vi"("input_spout"=w2340, "input_dataCurrent"=w2346, "input_dataExp"=w2343, "input_dataBlock"=w2335) -> ("output_state"=w2339:T2, "output_spout"=w2338:enum16{"Left", "Right"}, "idxDataBlock"=w2341:i32, "output_dataCurrent"=w2345:u16[], "output_dataExp"=w2344:u16[], "output_TpB_target"=→"TpB_target":u16, "output_iBlock"=w2336:u16, "output_dataBlock"=w2334:u16[][])  [unwired: 4 in]
              "iBlock" <- w2336
              "cSpout" <- w2338
            }
            frame "initBlock2" {
              n1421 = call "myRIO_BRig_RT__Case_Exp_State_initBlock2.vi"("input_spout"=w2363, "input_dataBlock"=w2364, "input_dataCurrent"=w2362) -> ("idxDataBlock"=w2359:i32, "output_dataBlock"=w2361:u16[][])  [unwired: 7 in]
            }
            frame "initTrial" {
              n1422 = xnode "Read/Write Control"("FPGA VI Reference In"=w2379, "error in"=w2378, "SelectionState"=FALSE) -> ("error out"=w2377:errorcluster)  [unwired: 1 out]
              n1423 = call "myRIO_Brig_RT__Case_Exp_State_initTrial__v2.vi"("input_spout"=w2380, "input_dataBlock"=w2375, "input_dataExp"=w2391, "input_dataCurrent"=w2392) -> ("output_state"=w2393:T2, "output_dataExp"=w2390:u16[], "output_dataCurrent"=w2385:u16[], "output_iTrial"=w2374:u16, "output_SolenoidReward"=→"SolenoidReward":bool)  [unwired: 3 in]
              "iTrial" <- w2374
              n1424 = local write "error out"(w2377) -> ()
            }
            frame "initTrial2" {
              # "trialUntilReward"
              n1425 = call "myRIO_BRig_RT__Case_Exp_subState_LC__initTrial__v4.vi"("input_dataCurrent"=w2399, "input_dataExp"=w2397, "input_dataLC"=w2409, "input_spout"=w2410, "input_dataTrial"=w2412) -> ("output_dataTrial"=w2411:u16[][], "output_LR_Wrong_Laser_l2"=w2401:bool, "output_dataCurrent"=w2398:u16[], "output_LR_Reward_Laser_l2"=w2402:bool, "output_LR_Reward_Event_l1"=w2408:bool, "output_LR_Wrong_Event_l1"=w2407:bool, "output_LR_Reward_Laser_l1"=w2406:bool, "output_LR_Wrong_Laser_l1"=w2405:bool, "output_LR_Reward_Event_l2"=w2404:bool, "output_LR_Wrong_Event_l2"=w2403:bool)  [unwired: 5 in]
              n1426 = call "myRIO_BRig_RT_dataExp_ItrialUntilReward.vi"() -> ("output_I_trialUntilReward"=w2416:i32)  [unwired: 11 in]
              n1427 = Index Array(array=w2397, index=w2416) -> (element=w2415:u16)
              n1428 = Equal?(x=w2410, y=enum16{"Left", "Right"}."Right") -> (x = y?=w2414:bool)
              n1429 = Not Equal To 0?(x=w2415) -> (x != 0?=w2413:bool)
              n1430 = xnode "Read/Write Control"("FPGA VI Reference In"=w2426, "error in"=w2425, "Left(F)_or_Right(T)"=w2414, "ignoreWrong"=w2413, "LR_reward_Event_l1"=w2408, "LR_wrong_Event_l1"=w2407, "LR_reward_Laser_l1"=w2406, "LR_wrong_Laser_l1"=w2405, "LR_reward_Event_l2"=w2404, "LR_wrong_Event_l2"=w2403, "LR_reward_Laser_l2"=w2402, "LR_wrong_laser_l2"=w2401) -> ("error out"=w2400:errorcluster)  [unwired: 1 out]
              n1431 = local write "error out"(w2400) -> ()
            }
            frame "initTrial3" {
              # "Cue1_CueType"
              n1432 = call "myRIO_BRig_RT_dataExp_CueLed.vi"() -> ("output_CueLed"=w2435:i32)  [unwired: 11 in]
              n1433 = call "myRIO_BRig_RT_arrTrig_init.vi"() -> ("output_arrTrig"=w2439:bool[])  [unwired: 11 in]
              n1434 = Index Array(array=w2436, index=w2435) -> (element=w2434:u16)
              n1435 = call "myRIO_BRig_RT_arrTrig_Cue1_CueType_AudioLed.vi"() -> ("output_arrTrig_Cue1_CueType_AudioLed"=w2437:i32)  [unwired: 11 in]
              n1436 = Not Equal To 0?(x=w2434) -> (x != 0?=w2433:bool)
              n1437 = call "myRIO_BRig_RT__Case_Exp_State_initTrial_dataTrial.vi"("input_spout"=w2452, "input_dataCurrent"=w2441, "input_dataExp"=w2436, "input_dataTrial"=w2454) -> ("output_laserPower_l2"=w2442:u16, "output_dataCurrent"=w2440:u16[], "output_dataTrial"=w2453:u16[][], "output_laserPower_l1"=w2449:u16)  [unwired: 4 in]
              n1438 = To Double Precision Float(number=w2449) -> (double precision float=w2451:dbl)
              n1439 = To Double Precision Float(number=w2442) -> (double precision float=w2445:dbl)
              n1440 = Replace Array Subset(array=w2439, new element=w2433, index=w2437) -> (w2438:bool[])
              n1441 = Divide(x=w2451, y=100.0 ("x")) -> (x/y=w2446:dbl)
              "power_l1" <- w2446
              n1442 = Divide(x=w2445, y=100.0 ("x")) -> (x/y=w2443:dbl)
              "power_l2" <- w2443
              n1443 = call "myRIO__convert__Voltage_to_FPGAvalue.vi"("input_voltage"=w2446) -> ("output_PortA"=w2431:u16)  [unwired: 9 in, 1 out]
              n1444 = call "myRIO__convert__Voltage_to_FPGAvalue.vi"("input_voltage"=w2443) -> ("output_PortA"=w2430:u16)  [unwired: 9 in, 1 out]
              n1445 = xnode "Read/Write Control"("FPGA VI Reference In"=w2448, "error in"=w2447, "AnaOut_0"=w2431, "AnaOut_1"=w2430) -> ("error out"=w2432:errorcluster)  [unwired: 1 out]
              n1446 = local write "error out"(w2432) -> ()
            }
            frame "initTrial4" {
              n1447 = call "myRIO_BRig_RT_dataTrial_activeRecording.vi"() -> ("output_activeRecording"=w2474:i32)  [unwired: 11 in]
              n1448 = call "myRIO_BRig_RT_dataCurrent_idxDataTrial.vi"() -> ("output_idxDataTrial"=w2477:i32)  [unwired: 11 in]
              n1449 = Index Array(array=w2479, index=w2477) -> (element=w2476:u16)
              n1450 = xnode "Read/Write Control"("FPGA VI Reference In"=w2469, "error in"=w2468, "A6_Act"="Recording") -> ("error out"=w2466:errorcluster)  [unwired: 1 out]
              n1451 = Boolean To (0,1)(Boolean="Recording") -> (0, 1=w2473:i16)
              n1452 = To Long Integer(number=w2476) -> (32bit integer=w2475:i32)
              n1453 = To Unsigned Word Integer(number=w2473) -> (unsigned 16bit integer=w2472:u16)
              n1454 = local write "error out"(w2466) -> ()
              n1455 = Replace Array Subset(array=w2478, new element=w2472, index (row)=w2475, index (col)=w2474) -> (w2471:u16[][])
            }
            frame "initTrial_LC_ENL1" {
              n1456 = call "myRIO_BRig_RT__Case_Exp_State_initTrial_LC_ENL1__v4.vi"("input_dataTrial"=w2498, "input_spout"=w2501, "input_arrTrig"=w2495, "input_dataBlock"=w2496, "input_dataLC"=w2502, "input_dataCurrent"=w2500) -> ("output_arrTrig"=w2494:bool[], "output_dataTrial"=w2497:u16[][], "output_dataCurrent"=w2499:u16[])  [unwired: 3 in]
            }
            frame "initTrial_LC_Cue1" {
              n1457 = call "myRIO_BRig_RT__Case_Exp_State_initTrial_LC_Cue1__v4.vi"("input_dataTrial"=w2517, "input_spout"=w2520, "input_arrTrig"=w2514, "input_dataBlock"=w2515, "input_dataLC"=w2521, "input_dataCurrent"=w2519) -> ("output_arrTrig"=w2513:bool[], "output_dataTrial"=w2516:u16[][], "output_dataCurrent"=w2518:u16[])  [unwired: 3 in]
            }
            frame "initTrial_LC_Sel" {
              n1458 = xnode "Read/Write Control"("FPGA VI Reference In"=w2534, "error in"=w2533, "A6_Act"=FALSE) -> ("error out"=w2535:errorcluster)  [unwired: 1 out]
              n1459 = local write "error out"(w2535) -> ()
              n1460 = call "myRIO_BRig_RT__Case_Exp_State_initTrial_LC_Sel__v4.vi"("input_dataTrial"=w2540, "input_spout"=w2543, "input_arrTrig"=w2537, "input_dataBlock"=w2538, "input_dataLC"=w2544, "input_dataCurrent"=w2542) -> ("output_arrTrig"=w2536:bool[], "output_dataTrial"=w2539:u16[][], "output_dataCurrent"=w2541:u16[])  [unwired: 3 in]
            }
            frame "ENL1_pre" {
              n1461 = call "myRIO_BRig_RT__Case_Exp_State_Enl1Pre__v3.vi"("input_I_lick"=w2558, "input_arrTrig"=w2555, "input_dataCurrent"=w2559) -> ("output_dataCurrent"=w2556:u16[], "output_state"=w2557:T2)  [unwired: 3 in, 4 out]
            }
            frame "ENL1" {
              n1462 = call "myRIO_BRig_RT__Case_Exp_State_ENL1__v3.vi"("I_lick"=w2578, "input_arrTrig"=w2576, "input_state"=w2582, "input_dataCurrent"=w2581) -> ("output_l1_laserOn"=w2574:bool, "output_l1_laserEvent"=w2575:bool, "output_state"=w2579:T2, "output_dataCurrent"=w2580:u16[], "output_l2_laserEvent"=w2573:bool, "output_l2_laserOn"=w2572:bool)  [unwired: 2 in]
            }
            frame "ENL1Penalty_pre" {
              # "Tcycle"
              # "counter"
              n1463 = call "myRIO_BRig_RT_dataCurrent_Tcycle_generic.vi"() -> ("output_Tcycle_generic"=w2609:i32)  [unwired: 11 in]
              n1464 = call "myRIO_BRig_RT_dataCurrent_count_generic.vi"() -> ("output_count_generic"=w2611:i32)  [unwired: 11 in]
              n1465 = call "myRIO_BRig_RT_dataExp_ENL_penalty.vi"() -> ("output_ENL_penalty"=w2604:i32)  [unwired: 11 in]
              n1466 = Index Array(array=w2605, index=w2604) -> (element=w2608:u16)
              n1467 = Replace Array Subset(array=w2606, new element #1=u16 0 ("new element/subarray"), index #1=w2611, new element #2=w2608, index #2=w2609) -> (w2607:u16[])
            }
            frame "ENL1Penalty" {
              n1468 = call "myRIO_BRig_RT__Case_Exp_State_ENL1Penalty.vi"("input_state"=w2625, "input_dataCurrent"=w2629) -> ("output_state"=w2626:T2, "output_dataCurrent"=w2628:u16[])  [unwired: 8 in]
            }
            frame "ENL2_pre" {
            }
            frame "ENL2" {
            }
            frame "ENL2Penalty_pre" {
            }
            frame "ENL2Penalty" {
            }
            frame "Cue1_pre" {
              n1469 = call "myRIO_BRig_RT__Case_Exp_State_Cue1Pre__v3.vi"("input_dataCurrent"=w2701, "input_dataExp"=w2697, "input_arrTrig"=w2694, "input_spout"=w2698) -> ("output_audioR"=w2695:bool, "output_audioL"=w2696:bool, "output_state"=w2699:T2, "output_dataCurrent"=w2700:u16[])  [unwired: 7 in, 5 out]
            }
            frame "Cue1" {
              n1470 = call "myRIO_BRig_RT__Case_Exp_State_Cue1__v4.vi"("input_state"=w2722, "input_dataCurrent"=w2723, "I_lick"=w2721, "input_arrTrig"=w2724) -> ("output_SelectionState"=w2715:bool, "output_CueLed_Event"=w2720:bool, "output_state"=w2716:T2, "output_dataCurrent"=w2717:u16[], "output_l1_laserEvent"=w2713:bool, "output_l1_laserOn"=w2714:bool, "output_l2_laserEvent"=w2718:bool, "output_l2_laserOn"=w2719:bool)  [unwired: 8 in]
              n1471 = xnode "Read/Write Control"("FPGA VI Reference In"=w2727, "error in"=w2726, "SelectionState"=w2715) -> ()  [unwired: 2 out]
            }
            frame "Cue1Penalty_pre" {
              # "Tcycle"
              # "counter"
              n1472 = call "myRIO_BRig_RT_dataCurrent_Tcycle_generic.vi"() -> ("output_Tcycle_generic"=w2763:i32)  [unwired: 11 in]
              n1473 = call "myRIO_BRig_RT_dataCurrent_count_generic.vi"() -> ("output_count_generic"=w2765:i32)  [unwired: 11 in]
              n1474 = call "myRIO_BRig_RT_dataExp_CueLed.vi"() -> ("output_CueLed"=w2747:i32)  [unwired: 11 in]
              n1475 = call "myRIO_BRig_RT_dataExp_Tcycle_Cue1Penalty_Audio.vi"() -> ("output_Tcycle_Cue1Penalty_Audio"=w2748:i32)  [unwired: 11 in]
              n1476 = call "myRIO_BRig_RT_dataExp_Tcycle_Cue1Penalty_LED.vi"() -> ("output_Tcycle_Cue1Penalty_LED"=w2746:i32)  [unwired: 11 in]
              n1477 = Index Array(array=w2759, index #1=w2747, index #2=w2748, index #3=w2746) -> (element #1=w2745:u16, element #2=w2743:u16, element #3=w2742:u16)
              n1478 = Equal To 0?(x=w2745) -> (x = 0?=w2744:bool)
              n1479 = Select(t=w2743, s=w2744, f=w2742) -> (s? t:f=w2741:u16)
              n1480 = Replace Array Subset(array=w2761, new element #1=u16 0 ("new element/subarray"), index #1=w2765, new element #2=w2741, index #2=w2763) -> (w2760:u16[])
            }
            frame "Cue1Penalty" {
              n1481 = call "myRIO_BRig_RT__Case_Exp_State_Cue1Penalty.vi"("input_state"=w2782, "input_dataCurrent"=w2783) -> ("output_state"=w2780:T2, "output_dataCurrent"=w2781:u16[])  [unwired: 8 in]
            }
            frame "Cue2_pre" {
            }
            frame "Cue2" {
            }
            frame "Cue2Penalty_pre" {
            }
            frame "Cue2Penalty" {
            }
            frame "Selection_pre" {
              n1482 = xnode "Read/Write Control"("FPGA VI Reference In"=w2861, "error in"=w2862) -> ("error out"=w2849:errorcluster, "SelectReward"=w2856:bool, "SelectWrong"=w2857:bool)  [unwired: 1 out]
              n1483 = local write "error out"(w2849) -> ()
              n1484 = call "myRIO_BRig_RT__Case_Exp_State_SelectPre__v5.vi"("input_dataCurrent"=w2860, "input_SelectWrong"=w2857, "input_SelectReward"=w2856, "input_dataExp"=w2850, "input_LickL"=w2848, "input_LickR"=w2847, "input_arrTrig"=w2855) -> ("output_state"=w2858:T2, "output_dataCurrent"=w2859:u16[], "output_l1_laserEvent"=w2854:bool, "output_l1_laserOn"=w2853:bool, "output_l2_laserOn"=w2851:bool, "output_l2_laserEvent"=w2852:bool)  [unwired: 3 in]
            }
            frame "Selection" {
              n1485 = xnode "Read/Write Control"("FPGA VI Reference In"=w2889, "error in"=w2888) -> ("error out"=w2876:errorcluster, "SelectReward"=w2883:bool, "SelectWrong"=w2882:bool)  [unwired: 1 out]
              n1486 = local write "error out"(w2876) -> ()
              n1487 = call "myRIO_BRig_RT__Case_Exp_State_Selection__v5.vi"("input_dataCurrent"=w2887, "input_state"=w2885, "input_dataExp"=w2875, "input_LickL"=w2874, "input_FPGA_SelectReward"=w2883, "input_FPGA_SelectWrong"=w2882, "input_LickR"=w2873, "input_arrTrig"=w2881) -> ("output_state"=w2884:T2, "output_dataCurrent"=w2886:u16[], "output_LC_Event_l1"=w2880:bool, "output_LC_Laser_l2"=w2877:bool, "output_LC_Event_l2"=w2878:bool, "output_LC_Laser_l1"=w2879:bool)  [unwired: 2 in]
            }
            frame "SelectReward_pre" {
              # "iState"
              # "nRewTrials"
              # "Tcycle\nGeneric"
              # "counter"
              n1488 = call "myRIO_BRig_RT_dataCurrent_nRewTrials.vi"() -> ("output_nRewTrials"=w2913:i32)  [unwired: 11 in]
              n1489 = call "myRIO_BRig_RT_dataCurrent_Tcycle_reward.vi"() -> ("output_Tcycle_reward"=w2902:i32)  [unwired: 11 in]
              n1490 = Index Array(array=w2900, index #1=w2913, index #2=w2902) -> (element #1=w2912:u16, element #2=w2901:u16)
              n1491 = Increment(x=w2912) -> (x+1=w2911:u16)
              n1492 = call "myRIO_BRig_RT__Case_Exp_subState_LC__Reward.vi"("input_spout"=w2920, "input_dataCurrent"=w2900, "input_dataLC"=w2919) -> ()  [unwired: 6 in, 2 out]
              n1493 = call "myRIO_BRig_RT_dataCurrent_count_generic.vi"() -> ("output_count_generic"=w2915:i32)  [unwired: 11 in]
              n1494 = call "myRIO_BRig_RT_dataCurrent_Tcycle_generic.vi"() -> ("output_Tcycle_generic"=w2916:i32)  [unwired: 11 in]
              n1495 = call "myRIO_BRig_RT_dataCurrent_iState.vi"() -> ("output_iState"=w2910:i32)  [unwired: 11 in]
              n1496 = Replace Array Subset(array=w2900, new element #1=w2911, index #1=w2913, new element #2=u16 0 ("new element/subarray"), index #2=w2915, new element #3=w2901, index #3=w2916, new element #4=u16 1 ("new element/subarray"), index #4=w2910) -> (w2922:u16[])
            }
            frame "SelectReward" {
              n1497 = call "myRIO_BRig_RT__Case_Exp_State_Reward__v2.vi"("input_dataCurrent"=w2940, "input_state"=w2937, "input_spout"=w2935, "input_dataExp"=w2927, "input_dataTrial"=w2926) -> ("output_dataCurrent"=w2939:u16[], "output_state"=w2938:T2, "output__L"=w2933:bool, "output__R"=w2934:bool)  [unwired: 7 in]
            }
            frame "SelectRewardPost_pre" {
              # "nRewards"
              # "nRewTrials"
              # "Tcycle"
              # "counter"
              n1498 = call "myRIO_BRig_RT_dataBlock_nRewards__L.vi"() -> ("output_nRewards__L"=w2955:i32)  [unwired: 11 in]
              n1499 = call "myRIO_BRig_RT_dataBlock_nRewards__R.vi"() -> ("output_nRewards__R"=w2954:i32)  [unwired: 11 in]
              n1500 = call "myRIO_BRig_RT_dataCurrent_Tcycle_generic.vi"() -> ("output_Tcycle_generic"=w2970:i32)  [unwired: 11 in]
              n1501 = call "myRIO_BRig_RT_dataCurrent_count_generic.vi"() -> ("output_count_generic"=w2972:i32)  [unwired: 11 in]
              n1502 = case shown="\"Left\", Default" w2948 {
                tunnel: w2960 -> [w2977 w2981]
                tunnel: [w2976 w2981] -> w2959
                tunnel: [w2978 w2979] -> w2958
                tunnel: w2957 -> [w2978 w2980]
                frame "Left", Default {
                  n1503 = Increment(x=w2977) -> (x+1=w2976:u16)
                }
                frame "Right" {
                  n1504 = Increment(x=w2980) -> (x+1=w2979:u16)
                }
              }
              "nRewards_Left" <- w2959
              "nRewards_Right" <- w2958
              n1505 = Equal?(x=w2948, y=enum16{"Left", "Right"}."Left") -> (x = y?=w2947:bool)
              n1506 = Select(t=w2955, s=w2947, f=w2954) -> (s? t:f=w2953:i32)
              n1507 = call "myRIO_BRig_RT_dataExp_Tcycle_RewardPost.vi"() -> ("output_Tcycle_RewardPost"=w2966:i32)  [unwired: 11 in]
              n1508 = call "myRIO_BRig_RT_dataCurrent_nRewTrials.vi"() -> ("output_nRewTrials"=w2956:i32)  [unwired: 11 in]
              n1509 = Index Array(array=w2967, index=w2966) -> (element=w2969:u16)
              n1510 = Index Array(array=w2950, index=w2956) -> (element=w2945:u16)
              n1511 = Replace Array Subset(array=w2950, new element #1=u16 0 ("new element/subarray"), index #1=w2972, new element #2=w2969, index #2=w2970) -> (w2968:u16[])
              n1512 = Replace Array Subset(array=w2952, new element=w2945, index (row)=w2946, index (col)=w2953) -> (w2951:u16[][])
              n1513 = local write "nRewards_cur"(w2945) -> ()
            }
            frame "SelectRewardPost" {
              n1514 = call "myRIO_BRig_RT__Case_Exp_State_RewardPost.vi"("input_state"=w2992, "input_dataCurrent"=w2995) -> ("output_state"=w2993:T2, "output_dataCurrent"=w2994:u16[])  [unwired: 8 in]
            }
            frame "SelectWrong_pre" {
              # "iState"
              # "Tcycle"
              # "counter"
              n1515 = call "myRIO_BRig_RT_dataCurrent_Tcycle_generic.vi"() -> ("output_Tcycle_generic"=w3016:i32)  [unwired: 11 in]
              n1516 = call "myRIO_BRig_RT_dataCurrent_count_generic.vi"() -> ("output_count_generic"=w3018:i32)  [unwired: 11 in]
              n1517 = call "myRIO_BRig_RT_dataExp_Tcycle_Wrong.vi"() -> ("output_Tcycle_Wrong"=w3014:i32)  [unwired: 11 in]
              n1518 = call "myRIO_BRig_RT__Case_Exp_subState_LC__Wrong.vi"("input_spout"=w3010, "input_dataCurrent"=w3011, "input_dataLC"=w3008) -> ()  [unwired: 6 in, 2 out]
              n1519 = Index Array(array=w3012, index=w3014) -> (element=w3015:u16)
              n1520 = call "myRIO_BRig_RT_dataCurrent_iState.vi"() -> ("output_iState"=w3006:i32)  [unwired: 11 in]
              n1521 = Replace Array Subset(array=w3011, new element #1=u16 0 ("new element/subarray"), index #1=w3018, new element #2=w3015, index #2=w3016, new element #3=u16 2 ("new element/subarray"), index #3=w3006) -> (w3013:u16[])
            }
            frame "SelectWrong" {
              n1522 = call "myRIO_BRig_RT__Case_Exp_State_Wrong.vi"("input_state"=w3032, "input_dataCurrent"=w3037) -> ("output_state"=w3029:T2, "output_dataCurrent"=w3036:u16[])  [unwired: 8 in]
              n1523 = Not Equal?(x=w3032, y=w3029) -> (x != y?=w3031:bool)
              n1524 = Select(t=myRIO_BRig_RT__Case_Exp_stateList."SelectWrong_post" ("Enum"), s=w3031, f=w3029) -> (s? t:f=w3028:T2)
            }
            frame "SelectWrong_post" {
            }
            frame "SelectTimeout_pre" {
              # "iState"
              # "Tcycle"
              # "counter"
              n1525 = xnode "Read/Write Control"("FPGA VI Reference In"=w3060, "error in"=w3059, "SelectionState"=FALSE) -> ("error out"=w3057:errorcluster)  [unwired: 1 out]
              n1526 = call "myRIO_BRig_RT_dataCurrent_Tcycle_generic.vi"() -> ("output_Tcycle_generic"=w3078:i32)  [unwired: 11 in]
              n1527 = call "myRIO_BRig_RT_dataCurrent_count_generic.vi"() -> ("output_count_generic"=w3076:i32)  [unwired: 11 in]
              n1528 = call "myRIO_BRig_RT_dataExp_Tcycle_Timeout.vi"() -> ("output_Tcycle_Timeout"=w3080:i32)  [unwired: 11 in]
              n1529 = local write "error out"(w3057) -> ()
              n1530 = call "myRIO_BRig_RT__Case_Exp_subState_LC__Timeout.vi"("input_spout"=w3071, "input_dataCurrent"=w3072, "input_dataLC"=w3070) -> ()  [unwired: 6 in, 2 out]
              n1531 = Index Array(array=w3074, index=w3080) -> (element=w3079:u16)
              n1532 = call "myRIO_BRig_RT_dataCurrent_iState.vi"() -> ("output_iState"=w3068:i32)  [unwired: 11 in]
              n1533 = Replace Array Subset(array=w3072, new element #1=u16 0 ("new element/subarray"), index #1=w3076, new element #2=w3079, index #2=w3078, new element #3=u16 3 ("new element/subarray"), index #3=w3068) -> (w3075:u16[])
            }
            frame "SelectTimeout" {
              n1534 = call "myRIO_BRig_RT__Case_Exp_State_Timeout.vi"("input_dataLC"=w3095, "input_state"=w3090, "input_dataCurrent"=w3100) -> ("output_state"=w3091:T2, "output_dataCurrent"=w3099:u16[])  [unwired: 6 in, 1 out]
              n1535 = Not Equal?(x=w3090, y=w3091) -> (x != y?=w3094:bool)
              n1536 = Select(t=myRIO_BRig_RT__Case_Exp_stateList."SelectTimeout_post" ("Enum"), s=w3094, f=w3091) -> (s? t:f=w3092:T2)
            }
            frame "SelectTimeout_post" {
            }
            frame "endTrial1" {
              # "Update dataBlock"
              n1537 = call "myRIO_BRig_RT__Case_Exp_State_endTrial1.vi"("input_spout"=w3129, "input_dataBlock"=w3128, "input_dataCurrent"=w3126) -> ("output_dataBlock"=w3127:u16[][], "output_dataCurrent"=w3125:u16[])  [unwired: 7 in]
            }
            frame "endTrial2" {
              # "update dataTrial"
              n1538 = call "myRIO_BRig_RT__Case_Exp_State_endTrial2.vi"("input_dataExp"=w3136, "input_spout"=w3145, "input_dataTrial"=w3149, "input_dataCurrent"=w3147) -> ("output_dataTrial"=w3148:u16[][], "output_dataCurrent"=w3146:u16[])  [unwired: 6 in]
            }
            frame "endTrial3" {
              # "nRewTrials"
              # "iTrial"
              # "I_blockUntilReward"
              # "TPB"
              # "end block?"
              n1539 = local read "STOP_endTrial"() -> (w3170:bool)
              n1540 = local read "STOP_abort"() -> (w3169:bool)
              n1541 = xnode "Read/Write Control"("FPGA VI Reference In"=w3160, "error in"=w3159, "SelectionState"=FALSE) -> ("error out"=w3153:errorcluster)  [unwired: 1 out]
              n1542 = local read "START"() -> (w3167:bool)
              n1543 = call "myRIO_BRig_RT_dataExp_IblockUntilReward.vi"() -> ("output_I_blockUntilReward"=w3177:i32)  [unwired: 11 in]
              n1544 = Index Array(array=w3163, index=w3177) -> (element=w3161:u16)
              n1545 = Not(x=w3167) -> (.not. x?=w3168:bool)
              n1546 = local write "error out"(w3153) -> ()
              n1547 = Not Equal To 0?(x=w3161) -> (x != 0?=w3175:bool)
              n1548 = Compound Arithmetic op=OR(w3170, w3168, w3169) -> (w3156:bool)
              n1549 = call "myRIO_BRig_RT_dataCurrent_nRewTrials.vi"() -> ("output_nRewTrials"=w3173:i32)  [unwired: 11 in]
              n1550 = call "myRIO_BRig_RT_dataCurrent_iTrial.vi"() -> ("output_iTrial"=w3174:i32)  [unwired: 11 in]
              n1551 = Select(t=w3173, s=w3175, f=w3174) -> (s? t:f=w3172:i32)
              n1552 = call "myRIO_BRig_RT_dataCurrent_TpB.vi"() -> ("output_TpB"=w3176:i32)  [unwired: 11 in]
              n1553 = Index Array(array=w3164, index #1=w3176, index #2=w3172) -> (element #1=w3165:u16, element #2=w3166:u16)
              n1554 = Less Or Equal?(x=w3165, y=w3166) -> (x <= y?=w3157:bool)
              n1555 = Or(x=w3156, y=w3157) -> (x .or. y?=w3154:bool)
              n1556 = Select(t=myRIO_BRig_RT__Case_Exp_stateList."saveData_dataBlock" ("Enum"), s=w3154, f=myRIO_BRig_RT__Case_Exp_stateList."dummyState" ("Enum")) -> (s? t:f=w3162:T2)
            }
            frame "endBlock" {
              # "R"
              # "L"
              # "idxDataBlock"
              n1557 = Equal?(x=w3197, y=enum16{"Left", "Right"}."Left") -> (x = y?=w3196:bool)
              n1558 = call "myRIO_BRig_RT_dataCurrent_idxDataBlockL.vi"() -> ("output_idxDataBlock__L"=w3200:i32)  [unwired: 11 in]
              n1559 = call "myRIO_BRig_RT_dataCurrent_idxDataBlockR.vi"() -> ("output_idxDataBlock__R"=w3199:i32)  [unwired: 11 in]
              n1560 = Increment(x=w3191) -> (x+1=w3190:i32)
              n1561 = local read "START"() -> (w3216:bool)
              n1562 = local read "STOP_endBlock"() -> (w3211:bool)
              n1563 = local read "STOP_endTrial"() -> (w3214:bool)
              n1564 = local read "STOP_abort"() -> (w3213:bool)
              n1565 = Select(t=w3200, s=w3196, f=w3199) -> (s? t:f=w3194:i32)
              n1566 = To Unsigned Word Integer(number=w3190) -> (unsigned 16bit integer=w3192:u16)
              n1567 = Not(x=w3216) -> (.not. x?=w3215:bool)
              n1568 = Replace Array Subset(array=w3195, new element=w3192, index=w3194) -> (w3193:u16[])
              n1569 = Compound Arithmetic op=OR(w3215, w3211, w3214, w3213) -> (w3212:bool)
              n1570 = Select(t=myRIO_BRig_RT__Case_Exp_stateList."endExp" ("Enum"), s=w3212, f=myRIO_BRig_RT__Case_Exp_stateList."dummyState_endBlock" ("Enum")) -> (s? t:f=w3220:T2)
            }
            frame "endExp" {
              n1571 = xnode "Read/Write Control"("FPGA VI Reference In"=w3223, "error in"=w3222, "A6_Act"=FALSE) -> ("error out"=w3224:errorcluster)  [unwired: 1 out]
              n1572 = local write "error out"(w3224) -> ()
            }
            frame "commConnect" {
              n1573 = call "myRIO_BRig_RT_comm_webdav_connect.vi"("input_password"="Host Password", "input_username"="Host UserName") -> ("output_Iconnected"=w3241:bool, "output_hSession"=w3255:T6)  [unwired: 7 in, 1 out]
              "Connected To Host?" <- w3241
              n1574 = case shown="False" w3241 {
                frame False {
                  n1575 = One Button Dialog(message="Connection Failed!\nData not being saved!") -> ()  [unwired: 1 in, 1 out]
                }
                frame True {
                }
              }
            }
            frame "commUpload_pre" {
              n1576 = Select(t=myRIO_BRig_RT__Case_Exp_stateList."commUpload_dataBlock" ("Enum"), s=w3262, f=myRIO_BRig_RT__Case_Exp_stateList."endBlock") -> (s? t:f=w3260:T2)
            }
            frame "commUpload_dataBlock" {
              n1577 = call "myRIO_BRig_RT_comm_webdav_uploadFile__data.vi"("input_fileName_prefix"=w3279, "input_fileName"="dataBlock" ("input_filename"), "input_hSession"=w3281) -> ()  [unwired: 8 in, 1 out]
            }
            frame "commUpload_dataCurrent" {
              n1578 = call "myRIO_BRig_RT_comm_webdav_uploadFile__data.vi"("input_fileName_prefix"=w3296, "input_fileName"="dataCurrent" ("input_filename"), "input_hSession"=w3298) -> ()  [unwired: 8 in, 1 out]
            }
            frame "commUpload_dataExp" {
              n1579 = call "myRIO_BRig_RT_comm_webdav_uploadFile__data.vi"("input_fileName_prefix"=w3313, "input_fileName"="dataExp" ("input_filename"), "input_hSession"=w3315) -> ()  [unwired: 8 in, 1 out]
            }
            frame "commUpload_dataLC" {
              n1580 = call "myRIO_BRig_RT_comm_webdav_uploadFile__data.vi"("input_fileName_prefix"=w3330, "input_fileName"="dataLC" ("input_filename"), "input_hSession"=w3332) -> ()  [unwired: 8 in, 1 out]
            }
            frame "commUpload_dataTrial" {
              n1581 = call "myRIO_BRig_RT_comm_webdav_uploadFile__data.vi"("input_fileName_prefix"=w3350, "input_fileName"="dataTrial" ("input_filename"), "input_hSession"=w3352) -> ()  [unwired: 8 in, 1 out]
            }
            frame "saveData_dataBlock" {
              # "idxDataBlockR"
              # "idxDataBlockL"
              n1582 = call "myRIO_BRig_RT_dataCurrent_idxDataBlockL.vi"() -> ("output_idxDataBlock__L"=w3372:i32)  [unwired: 11 in]
              n1583 = call "myRIO_BRig_RT_dataCurrent_idxDataBlockR.vi"() -> ("output_idxDataBlock__R"=w3373:i32)  [unwired: 11 in]
              n1584 = Index Array(array=w3374, index #1=w3372, index #2=w3373) -> (element #1=w3371:u16, element #2=w3370:u16)
              n1585 = Greater?(x=w3371, y=w3370) -> (0:w3369:bool)
              n1586 = Select(t=w3371, s=w3369, f=w3370) -> (s? t:f=w3367:u16)
              n1587 = Increment(x=w3367) -> (x+1=w3366:u16)
              n1588 = To Long Integer(number=w3366) -> (32bit integer=w3365:i32)
              n1589 = Array Subset(array=w3368, length (row)=w3365) -> (w3364:u16[][])  [unwired: 3 in]
              n1590 = call "myRIO_BRig_RT_comm_webdav_saveArrayToFile__2D_u16.vi"("Array"=w3364, "input_filename"="dataBlock") -> ()  [unwired: 10 in]
            }
            frame "saveData_dataCurrent" {
              n1591 = call "myRIO_BRig_RT_comm_webdav_saveArrayToFile__1D_u16.vi"("Array"=w3389, "input_filename"="dataCurrent") -> ()  [unwired: 10 in]
            }
            frame "saveData_dataExp" {
              # "runTime"
              n1592 = Get Date/Time In Seconds() -> (seconds since 1Jan1904=w3413:timestamp)
              n1593 = To Double Precision Float(number=w3413) -> (double precision float=w3412:dbl)
              n1594 = call "myRIO_BRig_RT_dataExp_runTime_seconds.vi"() -> ("output_RunTime_minutes"=w3411:i32)  [unwired: 11 in]
              n1595 = Subtract(x=w3412, y=w3410) -> (x-y=w3407:dbl)
              n1596 = To Unsigned Word Integer(number=w3407) -> (unsigned 16bit integer=w3406:u16)
              n1597 = Replace Array Subset(array=w3405, new element=w3406, index=w3411) -> (w3408:u16[])
              n1598 = call "myRIO_BRig_RT_comm_webdav_saveArrayToFile__1D_u16.vi"("Array"=w3408, "input_filename"="dataExp") -> ()  [unwired: 10 in]
            }
            frame "saveData_dataLC" {
              n1599 = call "myRIO_BRig_RT_comm_webdav_saveArrayToFile__1D_u16.vi"("Array"=w3428, "input_filename"="dataLC") -> ()  [unwired: 10 in]
            }
            frame "saveData_dataTrial" {
              # "idxTrial"
              n1600 = call "myRIO_BRig_RT_dataCurrent_idxDataTrial.vi"() -> ("output_idxDataTrial"=w3448:i32)  [unwired: 11 in]
              n1601 = Index Array(array=w3449, index=w3448) -> (element=w3441:u16)
              n1602 = Increment(x=w3441) -> ()  [unwired: 1 out]
              n1603 = To Long Integer(number=w3441) -> (32bit integer=w3445:i32)
              n1604 = Array Subset(array=w3446, length (row)=w3445) -> (w3447:u16[][])  [unwired: 3 in]
              n1605 = call "myRIO_BRig_RT_comm_webdav_saveArrayToFile__2D_u16.vi"("Array"=w3447, "input_filename"="dataTrial") -> ()  [unwired: 10 in]
            }
            frame "dummyState" {
              n1606 = call "myRIO_BRig_RT_dataCurrent_iTrial.vi"() -> ("output_iTrial"=w3467:i32)  [unwired: 11 in]
              n1607 = Index Array(array=w3468, index=w3467) -> (element=w3466:u16)
              n1608 = Equal?(x=w3466, y=u16 1) -> (x = y?=w3464:bool)
              n1609 = Equal To 0?(x=w3475) -> (x = 0?=w3476:bool)
              n1610 = Select(t=u16 13, s=w3464, f=u16 15) -> (s? t:f=w3461:u16)
              n1611 = Select(t=w3461, s=w3476, f=w3475) -> (s? t:f=w3474:u16)
              n1612 = Decrement(x=w3474) -> (x-1=w3473:u16)
              n1613 = Equal To 0?(x=w3473) -> (x = 0?=w3472:bool)
              n1614 = Select(t=myRIO_BRig_RT__Case_Exp_stateList."initTrial" ("Enum"), s=w3472, f=w3470) -> (s? t:f=w3469:T2)
            }
            frame "dummyState_endBlock" {
              n1615 = call "myRIO_BRig_RT_dataCurrent_iTrial.vi"() -> ("output_iTrial"=w3496:i32)  [unwired: 11 in]
              n1616 = Index Array(array=w3497, index=w3496) -> (element=w3495:u16)
              n1617 = Equal?(x=w3495, y=u16 1) -> (x = y?=w3493:bool)
              n1618 = Equal To 0?(x=w3504) -> (x = 0?=w3505:bool)
              n1619 = Select(t=u16 1, s=w3493, f=u16 3) -> (s? t:f=w3490:u16)
              n1620 = Select(t=w3490, s=w3505, f=w3504) -> (s? t:f=w3503:u16)
              n1621 = Decrement(x=w3503) -> (x-1=w3502:u16)
              n1622 = Equal To 0?(x=w3502) -> (x = 0?=w3501:bool)
              n1623 = Select(t=myRIO_BRig_RT__Case_Exp_stateList."initBlock" ("Enum"), s=w3501, f=w3499) -> (s? t:f=w3498:T2)
            }
          }
          n1624 = call "myRIO_BRig_RT_dataMTrig_main.vi"("input_dataMTrig"=w1586, "input_Solenoid_trig_L"=w1583, "input_Solenoid_trig_R"=w1582, "input_Audio_trig_L"=w1581, "input_Audio_trig_R"=w1580, "input_Laser_trig"=w1579) -> ("output_Laser"=w1520:bool, "output_dataMTrig"=w1585:u16[], "output_Solenoid_L"=w1523:bool, "output_Solenoid_R"=w1575:bool, "output_Audio_L"=w1577:bool, "output_Audio_R"=w1578:bool)  [unwired: 8 in]
          n1625 = Compound Arithmetic op=OR(w1583, w1582, w1581, w1580, w1579) -> (w1584:bool)
          n1626 = case shown="True" w1584 {
            frame False {
            }
            frame True {
              w1616 = FALSE
              n1627 = local write "MTrig_Solenoid_trig__L"(w1616) -> ()
              n1628 = local write "MTrig_Solenoid_trig__R"(w1616) -> ()
              n1629 = local write "MTrig_Audio_trig__L"(w1616) -> ()
              n1630 = local write "MTrig_Audio_trig__R"(w1616) -> ()
              n1631 = local write "MTrig_Laser_trig"(w1616) -> ()
            }
          }
          n1632 = local read "MTrig_Laser_Switch"() -> (w1518:bool)
          n1633 = Not(x=w1518) -> (.not. x?=w1519:bool)
          n1634 = And(x=w1520, y=w1519) -> (x .and. y?=w1514:bool)
          n1635 = And(x=w1520, y=w1518) -> (x .and. y?=w1516:bool)
          n1636 = Or(x=w1517, y=w1516) -> (x .or. y?=w1507:bool)
          n1637 = Or(x=w1516, y=w1515) -> (x .or. y?=w1506:bool)
          n1638 = Or(x=w1513, y=w1514) -> (x .or. y?=w1509:bool)
          n1639 = Or(x=w1514, y=w1512) -> (x .or. y?=w1508:bool)
          n1640 = Or(x=w1522, y=w1523) -> (x .or. y?=w1511:bool)
          n1641 = Or(x=w1576, y=w1575) -> (x .or. y?=w1510:bool)
          n1642 = case shown="False" w1596 {
            tunnel: w1593 -> [w1618 w1626]
            tunnel: w1595 -> [_ w1623]
            tunnel: w1594 -> [_ w1622]
            tunnel: w1497 -> [_ w1621]
            tunnel: w1573 -> [_ w1620]
            tunnel: [w1618 w1625] -> w1592
            tunnel: [w1617 w1624] -> w1591
            tunnel: w1505 -> [w1617 w1619]
            frame False {
            }
            frame True {
              n1643 = call "myRIO_BRig_RT__Case_Exp__recordLick.vi"("intput_state__trialEnd"=w1620, "intput_state__trialStart"=w1621, "input_lick__R"=w1622, "input_lick__L"=w1623, "input_dataCurrent"=w1619, "input_dataLick"=w1626) -> ("output_dataCurrent"=w1624:u16[], "output_dataLick"=w1625:u16[][])  [unwired: 4 in]
            }
          }
          n1644 = Or(x=w1577, y=w1563) -> (x .or. y?=w1553:bool)
          n1645 = Or(x=w1562, y=w1578) -> (x .or. y?=w1574:bool)
          n1646 = Or(x=w1597, y="STOP_abort") -> (x .or. y?=w1599:bool)
          n1647 = Select(t=w1543, s=w1544, f=w1542) -> (s? t:f=w1533:u16)
          n1648 = Select(t=w1504, s=w1546, f=w1545) -> (s? t:f=w1532:u16)
          n1649 = Select(t=u16 0, s=w1549, f=w1548) -> (s? t:f=w1535:u16)
          n1650 = xnode "Read/Write Control"("FPGA VI Reference In"=w1555, "error in"=w1554, "audioTrigger_L"=w1553, "audioTrigger_R"=w1574, "CueLed_Event"=w1521, "A3_SL"=w1511, "A1_SR"=w1510, "LC_Event_l1"=w1509, "LC_Laser_l1"=w1508, "LC_Event_l2"=w1507, "LC_Laser_l2"=w1506) -> ("FPGA VI Reference Out"=w1590:refnum<k20>, "error out"=w1589:errorcluster, "AnaIn_0"=w1526:u16, "AnaIn_1"=w1534:u16)
          n1651 = call "myRIO_BRig_RT_dataAnalog_enterData__PortA.vi"("input_iState"=w1497, "input_AI0"=w1526, "input_iEvent"=w1535, "input_AI1"=w1534, "input_iTrial"=w1533, "input_iBlock"=w1532, "input_index"=w1536, "input_dataAnalog"=w1552) -> ("output_dataAnalog"=w1551:u16[][])  [unwired: 3 in]
          n1652 = call "myRIO_BRig_RT_TCP__v3__PortA.vi"("input_hTCP"=w1540, "input_AI1"=w1534, "input_AI0"=w1526, "input_I_connected_TCP"=w1537, "input_iBlock"=w1532, "input_spout"=w1531, "input_iTrial"=w1533, "input_error"=w1538, "input_countTrial"=w1528, "input_iState"=w1497) -> ("output_hTCP"=w1539:refnum<k5>, "output_countTrial"=w1527:u16, "output_error"=w1501:errorcluster)  [unwired: 3 in]
          n1653 = call "test_myRIO_Exp_tLoop.vi"("input_error"=w1501, "input_Threshold"=w1498, "input_timestamp"=w1499, "input_state"=w1497) -> ("output_Threshold"=w1495:bool, "output_duration"=→"tLoop":dbl, "error out"=w1500:errorcluster)  [unwired: 5 in]
          "Threshold" <- w1495
          n1654 = node-c288() -> ()  [unwired: 1 in, 1 out]
          n1655 = Increment(x=w1535) -> (x+1=w1541:u16)
          n1656 = Increment(x=w1536) -> (x+1=w1550:i32)
          "cState" <- w1497
        }
        n1657 = node-c288(w1438) -> ()  [unwired: 1 out]
        n1658 = flat-sequence {
          tunnel: w1434 -> [w1483]
          tunnel: w1433 -> [w1482]
          tunnel: [w1481] -> w1426
          tunnel: [w1480] -> w1425
          tunnel: [w1486] -> w1427
          tunnel: [w1487] -> w1432
          tunnel: w1426 -> [w1487]
          tunnel: w1425 -> [w1486]
          frame #0 {
            w1477 = u8 0
            w1478 = u16 0 ("AudioLeft_phase_inc")
            w1479 = FALSE
            n1659 = xnode "Read/Write Control"("FPGA VI Reference In"=w1483, "error in"=w1482, "Counts_Reset"=TRUE, "audioTrigger_L"=w1479, "audioFreq_L_kHz"=w1477, "audioAmp_L"=w1478, "audioTrigger_R"=w1479, "audioFreq_R_kHz"=w1477, "audioAmp_R"=w1478, "A3_SL"=w1479, "A1_SR"=w1479, "A6_Act"=w1479) -> ("FPGA VI Reference Out"=w1481:refnum<k20>, "error out"=w1480:errorcluster)
          }
          frame #1 {
            w1485 = FALSE ("START")
            n1660 = local write "START"(w1485) -> ()
            n1661 = local write "STOP_endTrial"(w1485) -> ()
            n1662 = local write "STOP_endBlock"(w1485) -> ()
          }
        }
        n1663 = stacked-sequence {
          tunnel: w1411 -> [w1457 _]
          tunnel: w1409 -> [w1458 _]
          tunnel: w1408 -> [_ w1463]
          tunnel: w1407 -> [_ w1462]
          tunnel: w1406 -> [_ w1461]
          tunnel: w1405 -> [w1451 _]
          tunnel: w1387 -> [w1448 _]
          tunnel: w1386 -> [w1447 _]
          frame #0 {
            n1664 = call "myRIO_BRig_RT_dataCurrent_idxDataLick.vi"() -> ("output_idxDataLick"=w1452:i32)  [unwired: 11 in]
            n1665 = Index Array(array=w1451, index=w1452) -> (element=w1454:u16)
            n1666 = Array Subset(array=w1448, length (row)=w1447) -> (w1449:u16[][])  [unwired: 3 in]
            n1667 = Increment(x=w1454) -> (x+1=w1455:u16)
            n1668 = call "myRIO_BRig_RT_comm_webdav_saveArrayToFile__1D_u16.vi"("Array"=w1458, "input_filename"="dataMTrig") -> ()  [unwired: 10 in]
            n1669 = To Long Integer(number=w1455) -> (32bit integer=w1453:i32)
            n1670 = Array Subset(array=w1457, length (row)=w1453) -> (w1456:u16[][])  [unwired: 3 in]
            n1671 = call "myRIO_BRig_RT_comm_webdav_saveArrayToFile__2D_u16.vi"("Array"=w1456, "input_filename"="dataLick") -> ()  [unwired: 10 in]
            n1672 = call "myRIO_BRig_RT_comm_webdav_saveArrayToFile__2D_u16.vi"("Array"=w1449, "input_filename"="dataAnalog") -> ()  [unwired: 10 in]
          }
          frame #1 {
            n1673 = case shown="True" w1463 {
              tunnel: w1462 -> [_ w1465]
              tunnel: w1461 -> [_ w1464]
              frame False {
              }
              frame True {
                n1674 = stacked-sequence {
                  tunnel: w1465 -> [w1467 w1474 w1476]
                  tunnel: w1464 -> [w1468 w1473 _]
                  frame #0 {
                    n1675 = call "myRIO_BRig_RT_comm_webdav_uploadFile__announce.vi"("input_addText"=TRUE, "input_fileName_prefix"=w1468, "intput_fileName"="curExp_end", "intput_hSession"=w1467) -> ("output_Isuccess"=w1466:bool)  [unwired: 6 in, 1 out]
                    n1676 = case shown="True" w1466 {
                      frame False {
                        n1677 = One Button Dialog(message="!!! Warning !!! Your data is located at C:\\BehaviorRig\\commTransfer") -> ()  [unwired: 1 in, 1 out]
                      }
                      frame True {
                        n1678 = Wait (ms)(milliseconds to wait=u32 20) -> ()  [unwired: 1 out]
                      }
                    }
                  }
                  frame #1 {
                    n1679 = call "myRIO_BRig_RT__endExp_sendData.vi"("input_fileName_prefix"=w1473, "input_hSession"=w1474) -> ()  [unwired: 8 in, 2 out]
                  }
                  frame #2 {
                    n1680 = local write "Connected To Host?"(FALSE ("Connected To Host?")) -> ()
                    n1681 = call <vilib>:"Close Session.vi"("session handle"=w1476) -> ()  [unwired: 14 in, 1 out]
                  }
                }
              }
            }
          }
        }
      }
    }
    n1682 = local read "STOP_abort"() -> (w44:bool)
  }
  n1683 = case shown="True" w5 {
    tunnel: w4 -> [_ w3524]
    tunnel: w3 -> [_ w3523]
    frame False {
    }
    frame True {
      n1684 = call "myRIO__TCP_disconnect_forWrite.vi"("input_error"=w3523, "input_hTCP"=w3524) -> ()  [unwired: 9 in, 1 out]
    }
  }
  n1685 = xnode "Read/Write Control"("FPGA VI Reference In"=w16, "error in"=w15, "FPGA_Stop"=TRUE) -> ("FPGA VI Reference Out"=w21:refnum<k20>, "error out"=w22:errorcluster)
  n1686 = xnode "Close FPGA VI Reference"("FPGA VI Reference In"=w21, "error in"=w22) -> ("error out"=w20:errorcluster)
  n1687 = call <vilib>:"Reset myRIO.vi"("error in (no error)"=w20) -> ()  [unwired: 10 in, 1 out]
